vi "MPI2_continious_implementation.vi"() -> ()   [LabVIEW 2019]
uses:
  <vilib>/DAQmx/write.llb/DAQmx Write (Digital 2D Bool NChan 1Samp NLine).vi
  <vilib>/Analysis/baseanly.llb/Mean (DBL).vi
  <vilib>/Waveform/WDTOps.llb/WDT Number of Waveform Samples DBL.vi
  <vilib>/measure/maspectr.llb/FFT Spectrum (Mag-Phase) for 1 Chan.vi
  <vilib>/Utility/file.llb/Write Delimited Spreadsheet (DBL).vi
  <vilib>/Analysis/baseanly.llb/Mean (CDB).vi
  <extravilib>/ChannelInstances/Tag-dbl/Instantiate.vi
  <extravilib>/ChannelInstances/Tag-dbl/Endpoint.vi
  global_variables.vi
  <vilib>/DAQmx/create/channels.llb/DAQmx Create Channel (DO-Digital Output).vi
  <vilib>/DAQmx/miscellaneous.llb/DAQmx Fill In Error Info.vi
  <vilib>/measure/NI_MAPro.lvlib
  <vilib>/Analysis/NI_AALBase.lvlib
  <extravilib>/ChannelInstances/Tag-dbl.lvlib
panel:
  in  "Rotation homing":bool
  in  "Align laser":bool
  out "V":dbl=119.6
  out "f":dbl=60.0
  out "Power factor":dbl=0.42
  in  "Enable power plotting":bool
  out "Waveform Chart":T1(graph)={"apparant power (watt)"=260, "active power (watt)"=110}
  in  "Pumps":bool=TRUE
  in  "Bed motor":bool
  in  "Motor":bool
  in  "Clear plots":bool
  in  "noise floor stop":dbl format="%#_6p"
  in  "noise floor start":dbl format="%#_6p"
  out "noise floor mean":dbl=nan format="%0.2p"
  in  "Notes":string
  in  "Shift amp":bool
  in  "TX amp":bool
  in  "reset daq":bool
  out "Main loop has stopped":bool=TRUE
  in  "Update global variables Button":bool
  in  "sampling rate digital out":dbl=40000.0 format="%#_13p"
  out "Duration of last non-idle state (sec)":dbl=15.425420761108398 format="%.3g"
  out "Start of current operation":timestamp=timestamp(3649930230.9464383 s since 1904-01-01)
  in  "points to cut off (spect, baseline)":i32
  out "waveform diagram":waveform(dbl)(graph)={"t0"=timestamp(3649930210.976007 s since 1904-01-01), "dt"=1.9999999999999944e-06, "Y"=array[1400 elements], "attributes"=variant("NI_ChannelName"=variant(string "DAQ2/ai0"), "NI_UnitDescription"=variant(string "Volts"))}
  out "current system state":string="Halt"
  out "readout pts":dbl=1400.0
  in  "TX cycles per readout":dbl=70.0
  out "fft phase":cluster{"f0":dbl, "df":dbl, "phase":dbl[]}(graph)={"f0"=0.0, "df"=166.66666666666714, "phase"=[0.0, 2.7540425593822215, -0.41774944944908105, -2.9917235526827883, -2.707459047470282, 0.6249454301823627, -2.370005265361227, -0.5147516054486614, 1.6292245581402647, -3.015048559086423, -0.03670352730802006, 2.393200344197681, -1.08044143469344, -2.6803908360592543, 1.0570394839460617, -2.5979273293198157, 0.3746003915660465, -2.5959706251713066, -0.19275351229231943, 2.329251585108698, -0.15760892412814748, -2.619444396039319, 0.6040257569791547, 3.1232384157346744, 0.07286862625539897, -0.8349761222120895, 2.491919747557329, -0.6723952580821412, 1.4219523114985915, -1.8829118421278235, 2.1285349521917487, 0.552356415038526, -2.875631612970751, -0.05342422351139544, -3.1202940735703035, -0.2709814792342252, -2.311185357352345, -1.811383998858392, -2.671748431800669, 2.9870683722179363, 1.2306850799385998, -0.6468134335002678, -1.870147290118833, 2.9036130612188034, -2.3983442820995076, 1.5668696744042487, -1.485293516020373, -1.774984487522115, 2.9625095772350805, 1.2114987717362917, 0.41687473942441583, 2.4687530236172606, -1.3355374526401789, -2.7968528807659343, 2.101943215520195, -0.44240091404557225, 1.9209832862953178, -2.4648296902330324, 1.5814005745822983, -0.011182563965032996, -2.3033844922829383, -1.063349381886634, 2.98362939203973, -1.1699060479297414, 1.692187942816072, -0.9709312181777011, 2.5840242996804395, -1.2778035123496316, 2.1573220622434386, -1.454711675166049, -3.126308692769843, -2.9063943164949992, 1.8154945850625546, 0.5378211152892565, -0.5635004704527551, -0.5179360533926947, -1.0664830762078226, -2.85578162582117, -0.1307304567139906, -1.7830942043670113, 2.168572519489484, 0.2539399701165289, -1.761995933961074, -0.7037883915148042, 2.9248931112795344, 1.8880708587138288, -2.405324710669905, 0.4964528358342285, -2.2335794668638815, -1.8563013263901713, 1.1702254916879868, 1.346821279336611, -2.204173805999831, 0.24371100375848012, -2.7832475464457582, 0.5149589355035561, 0.8642594420795789, -2.138465254643337, 0.9421221120770275, -2.2015830793659377, -2.2320581146103033, 1.3064962642298776, -1.3403297469040394, 2.831661840993031, 1.203650750034212, -0.7830936947340748, 1.8935054792408772, -2.982278658911026, -1.4551705398152555, 1.4824075372105057, -2.0350358049171713, 0.0874608635446794, -3.0012334842500716, 0.7449814218063762, -1.0233846855331499, 2.8169824097043756, -0.8475187075508479, 1.7026399735381448, -1.5828785893756976, 2.411856644890007, -0.8925026524492577, 2.529100008950798, 0.29438318954641246, -0.7911902624060129, 2.7211777807148003, -1.4801195970408665, 0.32176108872110215, 0.8595087554168631, -2.91647820235481, -0.9096511107313615, 2.362809138152293, 2.907293981342496, -0.19224313497452372, 2.021057879936991, -1.0532144735572766, 2.012519718095534, -1.9914830889397996, -0.940305290573743, 1.990900580773453, -2.8166056044414414, 0.009837509283864954, 2.6788318641404985, -1.2304335536026125, 1.4372667618862258, 1.9357764794837633, -2.2510950656975703, 2.4346628297411255, 1.5058836975878664, 1.3396962452554966, 1.447915869036184, -1.6397026839530333, 1.504171455527829, 2.6168212185699384, 1.5694053636606018, 0.8991085911788249, -0.0060969118270417086, 0.704108075898119, -2.194015123877586, 1.9294214533962404, 0.9906316293947478, -0.8888372568865064, 2.289162228251758, -1.011412315749929, 1.7752562681031894, -1.5581078939472532, 0.17859807760715082, 2.874735233191739, -0.15245359027497854, 3.0007011237769623, 0.47492116042589866, -1.9517413705962434, 1.7541787652288416, 2.871211783717952, -0.6988862767001006, 1.6592170814733889, -1.984724345919406, 1.000667097748792, -1.277392682860055, 2.300663190120588, 0.9406642267225795, -2.225627302386333, 0.8369524876201423, 2.1419482177162994, -0.42734478695542544, 0.4971445385035397, -2.7772254798843785, -1.608828736322811, 1.6012576563947614, -1.9311241954870342, 1.1601617761002088, -0.16565949427291773, -0.8987336035561053, 2.7497346870958994, 0.15519553252081572, -0.504666162696194, -2.8946094052857503, 0.278888380464233, -2.5469229535229547, 0.9428862750232928, -2.2147669202386036, -3.0087387411619897, -0.13435457211182855, 1.8814556021187567, -2.821844805764982, -0.23032398091776898, 1.9406188587639086, -1.8842189519459873, 2.2014589910538898, 0.07337478156413231, -0.2911302207205093, -3.0449435192482284, -0.09316913489557556, 2.7136612125692263, -1.3430930954792781, 1.5138143613458557, -1.8498842584956878, 0.5518502747380236, 3.0080618183329366, -0.707945162576425, 2.703170009927386, -0.6497057490505204, 2.855450909859158, 0.26942250168014553, -3.1380634262559677, -0.6082811318546472, 1.8516114361794906, -1.668703750723555, -1.1764032056055431, 2.167716520633288, 1.407463459861506, -1.1939240181202087, -1.96033710810533, 1.187929862874151, -2.1284796193857574, -1.1135935933886567, 2.240393949288565, 0.7996933890629445, -2.57345171230255, 0.8624884057397524, -0.18394354977004865, 1.8027756604193184, -2.6673785459645694, -1.557213278823325, 2.5061775387898675, -0.7343428839851375, -0.17210152756946395, 0.24209791907571915, 2.385818454154299, -2.3543740463234584, 0.6542443429026227, -2.3887773967085653, -2.6994947310507627, 0.16374411301341452, 1.0844343637975538, -2.6690989874740985, -2.1301846552924837, 1.1305365372322789, 0.09211758596205234, -3.0431302638218725, 1.7433946946046488, -1.1964783090414477, 1.8527259341334916, 2.6471322822092316, -0.1747334806929663, -2.4861274055177014, 1.4236536162233422, 0.3224756043586924, -2.282310592209435, 0.3675863113242476, -3.062406752340649, -1.8048033049988987, 1.0339783508118279, -2.09586975663964, 0.7136083863527781, 2.7684330693562704, -0.7197481447382043, 2.670741867219946, -2.7957835404308424, 0.4756994642649445, -0.7547478534353032, -2.68586463998786, 0.11520506082972987, 2.3080887100868286, -0.5193216124366172, -2.9418065387151104, 0.8233942001211878, -2.3666441340336672, 1.9683026725269523, -1.084741955010314, 2.569431696746155, 1.8755768382902336, -1.735947948757583, 0.9158590456066058, -2.2488121057461252, 0.41900190348061833, 3.075960180992822, 2.4449872373857415, 0.3478853662006557, -2.3868864643332484, -0.7271255775728059, 2.4025639827624645, -0.6435555179469675, -2.900614106450232, 1.2388665786563127, -2.177306974845179, 1.2653133914574806, -1.132271539866567, -2.548990032776874, 2.370901279573129, -2.621199170173867, 0.6351848695609148, -2.309600610728719, 2.0369830137151075, 0.3265170729861214, -2.4499662648349423, 1.0087071287256246, 2.933669450086174, -1.417787571775661, 0.9076499105418954, 2.2043305075404036, -1.095109907014107, 2.050631628894733, -0.43008279174513486, -2.646699898696328, 0.5058833203755909, -2.110149021934083, -0.018918678796171286, 1.6366055531490655, -2.9565156100247982, -1.7980864195189612, -1.787336416541855, 1.6658447403981775, -0.6423657898020487, 2.7228871600915094, 2.497696300061502, -0.5646022220607995, 2.5896486310731213, -0.9023305265342931, 1.2845535414267544, 2.491477036620103, -0.793986898054272, -2.3598613453772, 1.8413389615810676, -0.7684267125264834, 2.986826489821479, 0.20901586046963358, 2.6427706874636714, -0.6754994858774919, 0.7912549355498941, 1.7487296459784962, -2.1072546596021295, -0.9966227622577787, 1.6328904486354898, -1.440773592697903, 1.9527647218101232, -0.9457649334446133, 2.4632987804112476, -0.3489955760626715, 2.5485323033875837, -1.005446962543904, 1.8683396278373134, 0.5531580992213784, -2.0682094583995325, 2.1785865491901446, -1.5253052839334211, 0.5315754829936222, -3.1250591763931, 0.15293660563839134, -0.5606359064596489, 3.1207390055910844, 0.25130904796050746, -2.9637815190386334, -2.5906696773361673, 0.743539865125924, -2.0635632215919726, 1.178460956556411, -2.2543432193778905, -0.5532661646812833, 1.7664410828245412, 2.0111450533039394, -1.120565684900094, 1.7986953093227194, -2.5415433153559417, 0.510868468073799, -2.7591935826661134, -1.3427432839709943, 2.0382642767004566, -0.8394413776070548, -2.537338985742467, 1.002033243911298, 1.8091856452425523, -1.7674405584336437, 0.35920606546557676, -2.4706157972378286, 0.7392519149737825, 1.7831960704815513, -1.8258580537840825, 0.7959328221750316, -3.0725238341834538, 0.01686990355077934, -3.0583047227202322, -0.589141148651516, -1.0606439709776083, 1.6681409593854466, -0.8869758395603837, 2.332987799635121, -1.681743700117981, 0.13265483928652452, 3.121424240790634, -0.4302490296605881, 2.0535402105381864, -1.5961317869067708, -0.3662549325580801, 2.416822962602054, -0.2904396313468742, -2.889336327493639, -0.23429968311574736, 2.545959095082067, -0.7096192469411521, 1.964741364163201, -1.730041669682325, 0.7090398077350987, 1.179690399659869, -1.8155853465290495, 1.2571528050807952, -2.6132504193125614, -1.1657097950185642, 0.9898389298050183, -2.1610027927415176, 1.1238212113010064, -2.7622547361674354, -0.38620274248449354, -2.984491475078884, -1.1801494512425614, 0.5079510451233106, -3.023239660006938, -0.14793964854238115, -1.0028641759351438, -1.8298714248779389, 1.431752830327668, -0.372604565289599, -2.111976907728673, -1.6051535714270946, -0.627399219833397, -1.5783940037689044, -1.6151441217412108, -0.9497452635424707, -0.8340388727489995, -1.6981535879152772, 0.38263659597426025, -2.968210990658363, 0.1730726497601832, -1.9153705321290466, 3.057546157287166, 2.205291722470598, 1.6134501828765986, 1.250953281266258, 0.9601343829974033, 0.5343499781125347, 1.3276675906004771, 0.5965879699558632, 0.14414069135444182, 2.8560398694614886, -0.40870446717026343, 1.542638627591486, -1.7960924268234595, 1.7145806375689276, 2.500728281163647, -1.3474489556512186, 0.6253773444357569, 2.1805456021135634, -0.0017853382921967362, -2.3700748617367458, 0.7717998892014187, -2.4682854842096864, -2.688099696833425, 1.4569756741555677, -2.022850117504677, 0.18146352087647405, -2.968035460087035, -0.3241793599380396, 2.2471208533035325, -0.8831825977854595, 2.830504149007527, -0.33506201397387, 2.8351405178488847, 0.2776696262316505, 2.9016066946593515, -0.8334126357193999, -2.507987526741747, 1.7426671623773033, -0.5417289161786527, 1.9224500719008697, -0.41496442296770203, -2.740802203027978, 0.00014411662639131332, 0.9885353149138045, -2.414084469045593, -0.14674622925736786, 2.1172083456191193, -0.5764227996247283, -2.19817138362822, 1.3689091158563123, -1.3322519629050043, 2.083166488628662, 2.75850235428238, -0.49569633158574966, -0.6091556660993676, 2.566654679807459, 0.5386278640586663, -1.7642954489637717, -0.2708519584868171, 2.6279278558234584, -2.76052145328226, 0.48234061791548194, 2.5679926362186523, -2.6064532140875, -0.02976639846895066, -2.3184427483744505, 0.33310384188549014, 2.379566379985213, -2.4465268020446604, 0.39191389408301736, -2.526036530944832, 1.7502630624088855, -0.6756243250094364, 0.7496052763980502, -1.4311402830397941, -1.684638761248864, 2.508989348459718, 2.1318749250863065, -1.627395188562372, 1.69214376606126, 1.3279942776168816, -0.8967371816826627, 2.674525668922968, 0.7278845134135274, -0.7453134817296895, -3.127933580573263, -1.4559858116436293, 1.5324073348385072, -2.2623698937484877, -1.2139904917323259, 0.3321865326835266, 2.774517907470611, -2.3834916405953406, 0.3775992516468575, 2.618557600355517, -1.1193506746267166, 2.4056012218302683, 1.0953081251316885, 0.0807635245525032, -2.8650175176315202, 0.06633059915074543, 3.108255648457706, -2.6281555013584885, -0.6728493883792693, 0.8982170775552722, -2.467911848936858, 0.2251130879432983, 1.3094095682743723, -1.7452461822975973, 1.9037671101602498, 0.2692816197561913, -2.60491544045963, 0.9509370482944391, -1.5596027897702691, 1.4429396515357684, -0.6550794488655424, -2.7970786630866233, 0.9465406749391486, 1.6972717539201554, -1.2358512552745493, 2.859757330129867, -0.651431969761258, 1.7813157508986759, -0.30018991623442065, -2.458829645707201, 2.4969055139900473, 0.13417138886497348, -2.7272428970903015, 0.27959215724505854, -2.713140546404327, 1.353315685896636, -1.4000699525981828, -3.023919861797397, 0.2139738186814114, -2.823704653256064, 1.7619580750329171, 0.14704980762164735, -1.367346362825192, 2.512174923849862, 1.292702694201784, -1.1543087848414244, 2.9685391033225974, 0.7220485420721938, -2.0570513351693864, 2.909710283102838, 0.17750819285937092, 0.9325849307591031, -2.501919311348002, 0.2171392757353715, 2.7197205937735576, -3.0015410466578762, 0.07892066384111603, -0.7734069722456183, 2.7946610195263304, 3.0212781609776433, -0.8017779037675032, 1.1969569933354216, -1.9859464554741195, 1.939696103455967, -1.479006377403267, 0.019995563226488648, -3.1230115438008226, 0.4342424774532695, -0.6952728305939098, 1.0229816409655819, -2.0603758042900426, 1.5631148611946764, 0.08252682658156427, -2.9946476005647775, 0.4541553124739888, -0.9826447835513735, 2.568571608998873, 0.5034463974116944, -2.2512370293978603, 1.9247937512429683, -2.758186529451972, -0.16328327349004884, 2.745227824640305, -0.27600472719070634, 3.0600663251670555, 0.5779793580418898, -1.9351508978905139, -2.944062127388997, -0.20463752723418507, -2.448553547905565, 1.6282989165337824, -1.080180309237574, 2.3032306343237092, -0.9351289289356145, 2.4810288227515636, -1.734998585032266, 1.934163102502813, -0.45517004339773137, 2.6260983195493113, -0.6252942634230008, 2.05345376947151, -1.2052358411757857, 1.5851434346391662, 2.9155968859671746, 0.8752613202637856, -1.6525755089363785, -0.18463853833227828, 2.7234047295485433, 1.0988545465606525, -2.242297665425119, -1.3937619510909733, 1.7504658443134995, -0.7807866519805128, 2.121795666896204, -2.4988185645044565, 0.43643795207773683, -2.5623206804319585, 1.9672319186012786, -0.4313809716611365, -0.7503110065885348, 2.6056452791860774, 1.8652931339656367, -0.485714124275401, -2.539908636212827, 2.1509984636830866, 0.617245296619356, 2.104623489256656, -1.6261802407185368, 2.1039289728202717, -1.470700521706089, -0.2510745221059939, 2.8155156715551573, -1.062791518472392, 0.8526886580626974, -2.2270616100970773, 1.7939297977550315, 0.16220909589713345, -2.7184764916022828, 1.0984464241275225, -2.040486566556227, 1.9740729635161505, -0.6049131727905106, 2.7647763575194975, -0.31890901315428244, 2.6595529123025985, -0.6554028882543155, 2.702171327717349, 0.15427593482135468, 1.9407164797032128, -0.7116792237513718, -2.9193685159956813, 1.1603672499589228, -1.253714460479042, 1.935104327522088, -0.9520698051053289, -2.945208479144284, 0.35300344973637643, 2.992141452530448, -0.9510545269233662, 1.9083188149179684, 1.882296639370573, -1.4127340898414624, 1.6581147173382742, -0.544081968873865, -2.9563735924869357, -0.23792907945643266, -0.08664421899668712, -3.0511665382909405, 2.3505331162555323, 0.3512590798471839, -2.203577644317914, 0.9243401829327751, 0.6905016989305272, -2.3172011699802906, -2.986497393871459, 1.4895757424726912, -0.7053727827563905, 1.4737838061842574, -1.5915714213345427, 2.260194344780683, 1.5371012239548374, -1.3671078645599828, 1.7701943352995453, 2.9799474066776237, -0.6169901641100062, 2.68023055792731, 0.6180074382376435, -1.6846735239867856, 1.021292517899627, -1.0321392572442891, 2.2387531179741296, -2.2775262175929574, 0.6730136922793635, 2.705524130615674, -0.5254342180261299, -2.398299277522749, 1.8867356604206764, 0.11037861917104375, -2.942603830022654, 1.2291602551064613, -0.04643970966507774, -2.6051215703608994, 0.3948810976564284, -2.7638261340669663, 1.3927119884264614, 0.9648717030418312, -0.6733534746885191, 3.0699125697465384, -0.7954344221272802, 2.665745109387664, -0.7524637482497626, 1.8833978480366045, 3.026059640211306, -1.0207202873714734, 2.3918077211986306, -0.4732538429732604, -2.5493565318250697, 0.3097434901148436, 1.4755826933358034, 2.8996652120089963, -0.4639338999555499, 2.6481298733314644, -3.0481693440909443, 0.5639195937204325, -1.758123653081914, 2.0929164865234466, 1.0493983313679878, 0.4312341153399969, -2.5133529048769514, 0.31115309972833816, -2.205936725953789, 2.1468878985231394, -0.19671651990435773, -3.0141022994885893, -0.011128100459949448, -2.5164803826644926, 1.0175456302091626, -1.3745587291818357, 3.0138020218299157, -0.863730804102301, 1.8539905645950367, 2.678613356195852, 0.012121176241664998, -2.9737392540851046, -2.0563045653546963, 0.5660548089094544, -2.839787969747755, 0.7374086590379478, -1.6218177124508901, 1.4298262102156536, -1.771981769179663, 1.7931352101075406, 1.1105421554248707, -1.837566617004617, -0.6081073819394741, 2.5754499806209328, 0.14414269190237375, -2.5381041776371185, -2.1671892146822347, 1.1297651827584954, -1.7667261074505065, 1.2808578780285342, 1.9383859858025012, -0.4572259173897579, 2.8353034618734463, -0.9824569319790475, 1.667026318737601, 3.1215096968456053, -0.773559819860795, -2.9251112684627536, 0.6384286174678868, 0.8474754773092013, 2.9824953300218984, 3.0981295192162523, -0.5756120764182968, 2.5802849339589327, -0.5168310323829991, -0.07536248392628349, -2.543567087752712, 1.330719873268674, -0.672328576433985, -1.7115541995753467, 2.4084502255455558, 0.17957388304270258, -1.0380143874522993, 3.1252796220180765, -0.13901807785019424, 2.900568902256346, -2.6746660644621723, 1.6812325032291666, 2.5936178017610914, -1.0577483903197933, -0.8583091787121501, 1.515660036925533, -2.288459367658298, 1.3343629995939172, -0.4274448443593649, 2.4571136013982002, -0.4514562840751234, -1.2459111684655748, -2.4490661605501023, 2.5527831908431486, 0.5136959710916381, -2.1107549720777308, -1.0368956909031488, 2.9033136714750096, -0.21460476883399254, -2.689728080190454, 3.0439216936452156, -0.09795262227017294, 2.495749703976162, -1.7337508509795796, 0.25146923034204327, -2.0885774040569083, 0.8030869762721157, 2.919646309739889, -0.6783614578476972, 2.65700015425027, 1.6630001934159717, -1.2705251868450735, 0.7130202847030426, -3.0636444516065895, 0.011216775739950453, -3.1074220264578942, 0.010653244934669395, 2.176503184995665, -1.042058025631164, -2.67562504444696, 0.9654930883022897, -1.4312407947889514, 0.31867196180608687, -2.888467320932099, 0.613547057450556, -2.7482398180779217, -0.34003922390177443, -2.8630408227079833, -1.4663748131970828, 1.1978104188470686, -0.338750516641942, -2.5354950119151165, 0.39584642658634744, 2.2511823430250395, -1.5206567069495636, 0.5330347182308556, -1.6083717577366752, -2.475568169172881, 2.2796480203603227, -1.5156290974975193, 0.8345075361033615, -1.3669377623560492, 2.529509560230595, 2.09492643521411, -1.0205181753606163, 2.2327577001586647, 1.9726293368884513, 0.2029707975484194, -2.962900764202443, -0.5912851593807913, 3.105708278247044, 2.057255299370193, -0.3900127338099452, 1.7886451892465023, -2.059711724130614, 1.3011946673805337, -1.5158133970234138, -3.071927339455458, 1.0784354873987443, -1.4414952745849792, 1.9024703445658466, -0.38953015878567476, 2.315543251618792, -0.3270227324776918, -1.819402089828396, 1.1714367420411165, -1.7380447678460644, 2.0226154246428876, -0.5656353587346558, -1.6388821641965623, 2.6647644706072753, -0.3697828832600953, -2.5990669276454588, 0.3394265001700578, -3.0871215131184915, -0.03350977552078354, -0.47388143557915846, 2.148618508348748, -2.460425643942731, 0.43227270022262343, 3.1306384331474457, -1.1054930079495384, 1.2915146249735612, -0.555730780954817, -2.5163788057804783, 1.5968331686665074, 0.2477077194166366, -1.4569263346723451, 2.8151633575495674, 2.458755159018332, -2.059473678369277, 1.9881149241942575, -0.10954623369266984, -2.638069181200175, 1.884271559232175, -1.638827624975623, 0.9442813603265399, -2.8954472852291118, 0.6539096133858422, -2.025487143592496, 1.3076127014601728, -3.110745479326435, -1.8108764067652123, 1.2535816088577916, -2.200309258511845, 1.7704029552736777, -0.10815007670568688, -2.1757302998662493, 2.069671606981699, -0.4040626261929413, 2.313319809828219, -2.8691010275234, -0.11070784799500669, 0.7580114702723455, -2.6368150447497802, 0.7786284956298831, -1.1688754608227738, 2.916639989523171, -2.968274492665614, 0.4757893735327881, -2.7930321897916777, 0.33977081228081796, -2.360076014238439, 0.784272132681561, 0.3816169080494048, 1.4138255765856176, -2.2095040314658436, 0.6429916063604616, 2.7099700619726868, -1.3024182827089108, 1.4084463395259685, 2.0120981573443775, -2.4824353152453513, 1.1189687853754873, -0.6621056013313161, 0.17405887909554316, -2.811518724102276, 0.5404116271585312, -0.971592405781462, -3.1101754651938243, 0.424513927079209, 2.8877867311961305, -0.5701659100467101, 2.161845744491495, 1.0255431872389773, -2.885417486370385, -0.6725110302329639, 0.7605370190311493, -2.1756109466854046, 1.39592471681857, -1.18718719947846, 3.071881788840178, 0.06928131896478305, 1.5515471497920168, 2.2534137223650204, -0.7509931241834826, 2.9870296745806155, -0.9699385683796223, 1.690007832778289, -1.5566776002508034, 1.9742269720166967, 1.5123133398558415, -1.1211534391671651, 2.775941078499385, 1.824535890111235, -0.627882744192828, 2.0628455538485078, -2.7163450356766727, 0.3900351550836249, -2.3565912542326815, 1.5862569686623909, -1.6820567568245655, 1.2656930128045998, -1.248767728135985, 2.3269802892746276, -2.643033485675305, 0.17989784769887698, -2.1922092890411435, 1.4690893308703339, -1.5379352487014688, 0.6572453052429962, 1.6842351250708696, -2.365675887125544, -0.31369855067107055, 1.7403172098317616, 0.5746113943672305, -2.250536359076875, 1.422406633442669, -2.406467601746575, 1.4163252865729303, -1.0137162472144192, 2.8248943291717987, -0.4829320883796166, 0.9556509464491407, -2.2728204359978195, 1.0958698376082479, -0.6943175232570544, -2.070141542478213, -2.6302750708447316, 1.0480219071710373, -2.6654695672821624, -0.3026625700254163, 2.411045156197171, -1.0747427904257583, 1.2585000062890082, 2.5376691764983175, -0.5072232455501554, 1.7118305492921926, -2.19296103703589, 1.5654690366761803, -0.8063444602960661, 2.346707883955403, -1.010870306036241, 0.26652490258268285, -2.6988212917660372, 1.214597876704182, -1.505599104941634, 0.9543231399620783, -1.9837536099576925, 0.9247294624069821, -3.0448114616357485, -0.16654781886801737, 2.7048675120923535, 3.0162008538548313, -0.6920223381518189, 2.136141031576818, -1.3435825844179943, 1.7613672789484416, -2.1323832154962212, 0.8937603953136487, -2.551934824567234, -0.032141997296331146, -2.0702708085515096, 0.3569935562951153, 3.138823246315803, -0.28677655612910685, 1.0937418839126127, -1.84696097134991, 1.2565218073270858, -2.1285667574718055, 1.7121777620402516, -0.7402364284457075, -0.5091012029515373, 2.679852230441668, -0.4663018106384946, 1.9646665176016138, -2.3490534053699594, 0.7434703495975993, -2.9270735344351753, -2.2192593699371357, -0.20343072390159692, 2.245202462760766, -0.8495160616648074, 2.736318754992669, -0.21926089395165413, 2.5895536433032396, -1.7070096330032456, -1.0158083234055626, 1.452082148142477, -2.7189201079413565, 0.6923374549122202, -2.202556430943985, -0.9598405920890763, 1.788887017419821, -1.2338374014075575, 2.5965353632046546, 0.24860417664545903, 0.8924295752251784, 2.4073221061901533, -0.8770193558937903, 2.7618139550642233, -0.4435649705201455, 1.6471660768484968, -1.9748071660682311, 0.44248007716085386, 2.799384288444242, -2.226381010413999, 0.9494920655618904, 2.5196130139941197, -1.4032319700724956, 1.156495437663549, -1.8652931884384618, 3.0734659384121423, -0.26951929480409204, -2.8799692983307814, 1.303443303659596, -0.01978267175402987, -1.46811291567088, -3.051808792277222, 2.172311436021013, -0.8633480637476854, 2.431690186189021, -0.502751629385919, 2.9201500020941165, 2.5238871360192436, -0.4358777467265639, 2.5031055651863485, -1.5261691124512629, 0.8474355529033445, 1.8119516925067631, -1.695209497216864, 0.6062659246966707, 2.9278478628266438, -2.9096310368197797, -0.5264754350964214, 0.9743930725392232, -1.3552922412853734, 3.0768304028614333, -0.3045539459195762, 2.545587789637512, 1.0324084035309868, -2.8613728394988107, -0.22277134258671846, 2.1245439525922727, -1.7238869923731035, -1.4627701565418878, 1.5086505616512276, -2.794863290434653, 0.15568451237741993, -2.195604094562416, 0.7216988967484212, -2.8572756589490513, 0.07357909971429183, -1.8287009331454764, 1.9966034479124604, -2.0598928673726524, -2.7896496017022465, 1.0676418569974464, -1.743983906588147, 0.9794982349133036, -2.7542212982327983, 0.9422963219469825, -1.4370521423633564, 2.385856217689936, -0.7786724496108143, 2.551264284658099, -0.7874950333562143, 2.203748769329088, -0.7485047904414031, 0.8825489131884457, -1.4784413322922143, 3.13523734436019, 2.228584933254406, -0.5794369723331801, 2.1424595963295383, -0.6590298006070042, -1.7673187970416888, 1.3699134662551367, 1.0695962209127687, -0.960581932847277, -1.0390943138184625, -2.449443096911296, 1.614483550033886, -0.9830076477571836, 2.168992450309726, -1.370685572931924, 1.3565172872579825, -2.336386965297111, 0.6197910802692542, -2.344161346619624, 0.17559552046889557, 2.313696728982058, -0.5684404265838676, -0.7749491636146788, -3.08615199767987, 1.9320643623556393, 0.6634529752684392, 0.06654448657712722, -3.0846790730979867, -0.5053088046114536, 1.388371216006345, 1.5136242882194861, -1.51033316842799, -1.9438280385585442, 1.4695412483933843, -2.7450529165441306, -0.5450429483514694, 1.08821543163101, -1.1536503086138679, 2.453191802448807, -0.14335654642151924, 3.052322964862365, -1.7233507784018072, 1.3309913884654867, 3.1226591858947144, -1.9563531633252866, 0.14333284809700247, 0.6654675074875196, -1.7833475498409017, 1.5282033576705654, -1.0656760212139198, -2.7320419116991714, 1.6261894703171715, -1.934384938212058, 0.7871542119401843, 1.6891205955520372, -2.965472955499157, -0.3967496308230906, -3.0209591975850385, 0.7063283717786318, -1.413839697723809, 2.3047235633751937, -1.3456233748583486, -2.310748993303288, 1.3380455605483028, -2.252353133687334, -1.007578212142689, 2.3192984231574747, 0.9829741984675008, -2.3883495102595895, 0.985764991350256, -0.23856867868005707, -2.383074033654719, 1.4666665363684508, 2.9017309889736675, 0.3525688778641894, -1.757333800399145, 2.050124180950513, -0.4334326096421342, -1.9602427501701536, 1.929307400330661, -2.267822856698649, -0.7073421157798139, 2.4611492749524975, -0.36640557450473993, -2.6181500528549475, 0.40311055493507936, -2.434224007134926, -2.6465143721565436, 0.7134239266934059, -2.9196238148015814, -0.09897049078233182, 1.2226737642483225, -2.1801890748649915, 0.9638460741031623, -1.0292078704281071, -1.3161387756552627, 2.131340361529748, -0.7366771588514918, 2.6785776346815053, -2.431888850726272, 0.8510075408044548, -1.7215064324000349, 2.271449613138369, -0.9397678306538603, 1.4176857754442111, -2.458316780997201, 0.3333479386073043, 0.6466892932019946, -2.4887283094011505, 0.06595588362458445, 1.7759416516491897, -1.3156378756967018, 0.681677176848216, 2.767500360407054, 2.4290074442463867, -0.5584934107391647, 2.2838355888640103, -2.6693746295278897, -0.721500161550526, 0.8305472686604598, -2.888838211223999, 0.36049127801667946, -2.954461068886556, -0.29106076906884115, 2.4473111593457317, -1.1653984597050084, 1.6454200188089136, 0.1378818071348789, 3.124422709808076, 0.04655850838229611, -2.9936604660172463, -1.687842044638684, 0.33737683243916466, -3.081329400775572, -0.38940882241971325, 1.607881826268852, -1.4847441989561796, 1.6828010851600108, 2.727607794269626, 0.773393474612303, -0.939151684254625, 2.749308071835674, 2.4307800176874363, -1.396012027360456, 0.9399631537318961, -2.7377937319746755, 0.5961403313257109, -1.3913579604427555, 1.8523201530045845, -1.5796704556798358, 1.4513031618879204, -1.2044533178095884, 1.3291082982313418, -2.6513554186879857, 0.6763463839115226, -1.3223224094413768, -0.9027729644935903, 2.5402903148445195, -0.5026447652791285, 2.3899878465783746, -0.5887832929819106, -2.817503179132805, 1.1009979435117832, 2.2974331248869606, -1.2080094832204378, -2.2872069739795218, 1.5575981437099562, -1.9878334777061717, -0.038678558051125085, 2.989398615266818, -1.4773564061913294, 2.7737627042041018, 0.5980708974361006, -1.3624946494378485, 1.7763885881955879, 1.3667932276339032, -1.4625626897188568, 2.878017820047102, -0.11019615609114743, -0.21195385518571583, -2.8310117596111644, 1.1315727312499262, -1.1563589526596563, 2.40762124116393, -0.5690256392438064, 2.3944419607360867, -0.4956887515079857, -3.069507078353702, -1.0410117525010907, 1.130387664652052, -2.1975704116127805, -1.8636668302021266, 1.044772750789791, -2.9994187336065674, -0.7615262200237719, 0.4372035572332126, -2.1754524438731413, 1.7419915463934326, -1.1888370085726094, 1.1430422422881916, -1.614199113484965, 2.3859546088241785, -0.6687711925523698, 1.6593150552017215, -0.8217719041293505, 2.297889400522578, -0.5980122260232852, -0.030868183427800257, -2.8379302107248097, 0.89747935739299, -0.6849577627070423, 2.306817241582839, -1.4091867620722667, 0.15565424042509343, 1.957221035234614, -1.9367384535278211, -0.9734280147034378, -2.12430784881939, 0.9159536225275885, -2.189467486661428, 0.7078939097471529, -2.3986898995946593, -1.5683999989094228, 2.183702732591611, 0.047984705354305365, -1.1985977902963327, 2.3459461687072842, 2.164583253229524, -0.7529445870625288, 3.0021777991611143, -1.0097920527194986, 2.3810424364901537, -0.12342570756526414, -1.0740703664218525, 1.8949006922375287, -1.1214960989448763, 2.215564246850753, -1.4748614852061788, 1.3618809852566327, 3.120188806624154, -0.8508708903014319, 1.168379273243559, -2.445796003750018, 0.202400316559645, 2.999193446426725, -0.1894216674062962, -2.6000397626931386, 1.3115030806337187, -1.5295304473323301, 1.4445198466548173, -1.1222069380003843, 1.2476829207573232, -2.4211544681343677, 1.344471534164131, 0.7439596447231648, -2.9031710679521052, -0.06576970000470049, -1.569925849484693, 2.2423593955489034, -0.9691866068739777, -3.133832899196044, 1.2362132726018655, -1.8363430644515046, 0.38224286375236094, -2.7297120299135744, 1.073909406326477, -1.8094074377887333, -2.16647704505428, 0.8379742129973163, -2.8677096274666805, 0.0914608497055886, -3.0419340053702015, -2.7650747242481453, 0.23681574608022923, -2.835734101467477, -2.02158524567706, 2.4080064173132616, 1.5730195632065045, -1.4778688355793552, -0.36303301687268197, -1.4057781374689775, -2.8884924811780364, 1.290145701837535, -1.3133809334787196, 1.536818216317374, -2.351388669904487, 0.2948797207736677, -1.663353362631088, 2.8734673058340725, 0.7002148139700289, 2.911734354686056, -1.5149789152715065, -1.9601639064457783, 0.7583223995676716, -2.59053564326091, 1.755829764903252, -1.6007208412621265, -2.2676024351517583, 0.7397083027550687, 2.762988681409429, -1.923385581440203, -0.24646772608763412, 2.763215765590017]}
  out "fft magnitude":cluster{"f0":dbl, "df":dbl, "magnitude":dbl[]}(graph)={"f0"=0.0, "df"=357.14285714285813, "magnitude"=[0.0008504053868740763, 0.00038817631685509143, 0.00024200224947985637, 9.528178631548858e-05, 0.0002637879165738081, 0.00021266182371736548, 0.00026328121141686847, 0.00023246712294296184, 0.000170218058535424, 0.0002214629029401282, 0.00018340054429958835, 8.001472603600311e-05, 0.00013754196060766958, 3.217049878774864e-05, 5.537673098252246e-05, 6.655938865999862e-05, 4.616030095470193e-05, 2.1630531609063795e-05, 4.179763229329e-05, 1.8814796240273995e-05, 1.3861298250629736e-05, 2.9069300780021175e-05, 2.8472339253991566e-05, 1.8424246742207424e-05, 1.753088012974326e-05, 1.306056803504805e-05, 3.4577365984582725e-05, 5.301188067480479e-05, 1.6759110050633133e-05, 2.3101475044572646e-05, 5.177641082400739e-05, 3.394906563604761e-05, 1.3132867773952802e-05, 3.1681502670681254e-05, 1.9715168809233675e-05, 1.3985884261973671e-05, 1.837749235084362e-05, 1.9973617836840333e-05, 2.4255481464396008e-05, 2.4665173812009865e-05, 4.707620481503321e-05, 6.311647801194837e-05, 4.488684282424727e-05, 1.2885634548615734e-05, 2.4922302761336312e-05, 2.1431564830585327e-05, 2.786224096563646e-05, 3.020467484373902e-05, 2.054604085520399e-05, 3.169567673791574e-05, 2.0207728536922567e-05, 1.065141938217561e-05, 3.146617247110547e-05, 2.7916144407665383e-05, 1.4918503266654084e-05, 1.779704199661841e-05, 3.234136307047193e-05, 2.1721669900347797e-05, 9.931596116906507e-06, 3.259678771803358e-05, 2.1427156650808268e-05, 8.384285064686837e-06, 1.0228306764216333e-05, 5.611321058406616e-06, 2.207236556629755e-05, 1.3171723022762692e-05, 2.752768826710181e-05, 5.5957918917806525e-05, 4.502029999159639e-05, 0.005619981982229031, 0.011292260760809582, 0.005683551354431588, 4.169306727389849e-05, 2.7117617973734804e-06, 1.4351011125243378e-05, 3.8809428679766734e-05, 1.5026431605937022e-05, 4.477546265331766e-05, 6.044557416810212e-05, 2.17198760471519e-05, 2.9394807773491078e-05, 1.6546392552319972e-05, 2.4304501237231662e-05, 7.978493975242355e-05, 0.00015200741145628816, 8.851111017295075e-05, 4.01574178811118e-05, 1.4405739900073762e-05, 2.763186956702801e-05, 9.968710859956455e-05, 0.00012944367932850922, 8.373195405705675e-05, 2.5275541765656555e-05, 1.0649556422770253e-05, 1.2917727847079208e-05, 5.069113356592643e-06, 2.3994304009489225e-05, 2.187398289490739e-05, 2.096656747147603e-05, 4.423623994969366e-05, 4.1171463397910596e-05, 3.482156326989098e-05, 5.942741930762911e-05, 5.762216782730335e-05, 2.4321721886006758e-05, 5.704237228851119e-05, 4.2162101788859934e-05, 2.0603941385693077e-06, 2.3183737704646296e-05, 1.8358904874439327e-05, 1.8590670877773975e-05, 3.8885496597937974e-05, 5.5762053114025594e-05, 1.4795480266028205e-05, 2.949768542674144e-05, 3.5873556009240995e-05, 1.743836998440714e-05, 1.976981196044153e-05, 9.476564055011497e-06, 2.9238815828459964e-05, 6.449774684554353e-05, 4.207101647278669e-05, 3.142037692906569e-05, 5.299537341734831e-05, 4.633675735520215e-05, 2.3030155931717667e-05, 2.957672935163901e-05, 3.5212076306819656e-05, 8.920359888175078e-05, 0.00010229123186171714, 3.300444707240487e-05, 3.728184837628863e-05, 9.211726462222275e-05, 7.646964959447946e-05, 4.510166130725302e-05, 2.3660451819198002e-05, 7.280570680797218e-05, 0.00010304538586984465, 2.9559511964213285e-05, 0.0005302612178855428, 0.000957086970092551, 0.00039360471273656365, 7.939489173698186e-05, 8.052585547959751e-05, 9.818866379572031e-05, 3.652935902651936e-05, 5.050188736488592e-05, 0.00013718448142148118, 0.0005650845059801568, 0.0006688540170989411, 0.00020038969741937782, 3.5727710854349185e-05, 8.313583611856988e-05, 8.882564867739533e-05, 8.617858072815891e-05, 8.402619438125791e-05, 7.858205505848314e-05, 6.910274162172801e-05, 2.5445264798726963e-05, 3.374198789293683e-05, 8.01833040632245e-05, 7.768312604919405e-05, 6.108191397131242e-05, 2.4075771656088893e-05, 3.7410501260855885e-05, 6.591520518094664e-05, 6.402691133532337e-05, 0.00010847162480758214, 0.00015097701789772215, 5.54900845097092e-05, 5.82925246503782e-05, 8.502563495808675e-05, 9.410116125085737e-05, 5.062652087588863e-05, 4.0084336561493394e-05, 8.765242406699333e-05, 6.069280635502966e-05, 7.656586480117282e-05, 8.11655228618997e-05, 6.747021509081193e-05, 0.00013422141683655178, 0.0001198062145826111, 0.00011684791990073103, 0.00014844152847970344, 7.533987610526805e-05, 9.660461409681184e-05, 8.271380200944031e-05, 0.00010772005891389226, 5.1536215571431944e-05, 7.907349311220803e-05, 0.00011008713821217489, 5.611143506588776e-05, 6.835418850072209e-05, 6.468717931347631e-05, 7.011773167523613e-05, 7.844663236948679e-05, 0.00011517819669445895, 5.112016444436995e-05, 6.622821340550411e-05, 2.9948995853194973e-05, 2.0673669166364874e-05, 7.104805661608881e-05, 3.8231616126054805e-05, 7.757726527849755e-05, 0.00011120353079157232, 0.0001156544499805909, 0.00010321312170049135, 6.859189348948907e-05, 5.0093322970591856e-05, 0.09805481810720634, 0.19607444971142848, 0.09799131522534363, 8.185703633936342e-05, 9.023862981719941e-05, 8.33336613677052e-05, 3.072478653277527e-05, 6.91951632818372e-05, 0.0001193101316893837, 0.00014466470350483788, 0.00011092785548138803, 0.00010875137480783978, 0.00011969914531948508, 8.215402993794012e-05, 7.47869906957124e-05, 7.506346710047723e-05, 3.6922531938318056e-05, 2.798938380465293e-05, 4.476831381615353e-05, 7.397689244431366e-05, 4.251343909200035e-05, 2.125111643631236e-05, 0.00010354912674592199, 0.0001270532559199752, 6.246344224111225e-05, 7.544781595175229e-05, 8.934076974148615e-05, 9.245571713511173e-05, 9.194522743291552e-05, 9.269169948924399e-05, 8.940079122321851e-05, 8.413424002863418e-05, 3.569935933953516e-05, 5.2801825202616964e-05, 8.767393321188262e-05, 3.7093000702971066e-05, 2.0675807126056224e-05, 4.075699404161345e-05, 6.439280412661862e-05, 3.403202221626089e-05, 4.2125591233896484e-05, 5.551201427825648e-05, 1.514552491215281e-05, 7.667450752192568e-05, 6.660014083982042e-05, 2.7945379422364662e-05, 4.771594881983721e-05, 6.384064302783832e-05, 7.260835647492111e-05, 7.661940271132592e-05, 9.111068904890714e-05, 0.00010221905190175964, 4.166199919025971e-05, 2.376701383640949e-05, 3.8650808014525085e-05, 6.076001099427476e-05, 4.5788622084527096e-05, 3.088411725824502e-05, 5.2208172418654514e-05, 4.832997375680953e-05, 8.713855871748613e-05, 7.350415802712401e-05, 4.96541807530671e-05, 9.524379395252615e-06, 5.137184367304492e-05, 0.00010501977699402518, 0.0001420005982818947, 7.17138902652235e-05, 4.082250059735444e-05, 2.930210205538657e-05, 7.806720602514079e-05, 0.00010572842456426828, 8.096781583320538e-05, 9.510101184099318e-05, 0.00012592698016664847, 8.700092065809788e-05, 7.26066698595426e-05, 8.1782888095692e-05, 8.395272671305381e-05, 4.224770711871406e-05, 1.106995608081516e-05, 9.735532011103209e-06, 2.752067047021845e-05, 3.389009402906295e-05, 5.771250370036166e-05, 8.377723533434321e-05, 7.885387480125367e-05, 8.175670855436304e-05, 3.1600655612276425e-05, 3.450598909324276e-05, 4.290939774602672e-05, 2.6669391405114603e-05, 1.68522685967845e-05, 3.067982411031092e-05, 6.618659933038466e-05, 5.890041202681141e-05, 3.3847427911004505e-05, 2.416357143729828e-05, 5.378864338343087e-05, 0.00010485575228436024, 0.00010679460636927175, 6.235105363152511e-05, 3.5083076992758505e-05, 2.107406800742241e-05, 1.3643219728132798e-05, 3.0218836958947234e-05, 9.97024613781021e-06, 7.284950775457467e-05, 5.888651837412118e-05, 3.1798575870669756e-05, 8.158835166962577e-05, 8.962841353592735e-05, 8.585227163170281e-05, 5.5251147437784776e-05, 2.4121475161745472e-05, 4.93902500008769e-05, 1.950784341157193e-05, 9.66089261607798e-06, 6.890657493671837e-06, 3.1691775305223734e-05, 4.984740860185563e-05, 6.80353365408807e-05, 4.635014677054849e-05, 1.1835456329046845e-05, 0.00011900358050276759, 0.0001736711495213785, 0.00010111643667807346, 2.2198435819156723e-05, 2.7245105291417147e-05, 2.8229880152154535e-05, 4.054801820655859e-05, 1.4382785180247931e-05, 1.5969161307833768e-05, 2.2182213282728042e-05, 4.080347943463341e-05, 2.2234539668015663e-05, 1.2084971742605094e-05, 3.4316295494870145e-05, 3.670131560604153e-05, 1.6522860414520775e-05, 0.0005621855389392655, 0.0011356153109112618, 0.0005602914992824028, 2.5748031929675336e-05, 3.234209580549303e-05, 1.8826547170253713e-05, 2.80179066118143e-05, 6.820735393106553e-05, 5.508699792990793e-05, 3.0759346790288734e-05, 7.887914570387843e-05, 6.51701106922191e-05, 1.578292527457717e-05, 5.45020849734267e-05, 5.5694022062020294e-05, 4.6649772844886225e-05, 1.7283341404481173e-05, 1.028135108369353e-05, 5.585402391581478e-06, 4.5837578402369435e-06, 4.147931600126257e-05, 4.0202474065237335e-05, 3.166550631285438e-05, 1.7522614797695876e-05, 3.675341615834371e-05, 5.654836662448283e-05, 2.9684504589810096e-05, 1.8505556776919318e-05, 1.9136672812110446e-05, 1.768687700025057e-05, 0.00010809887977772355, 0.00017157487256434258, 4.833875665458884e-05, 4.8195550082155284e-05, 3.2247474474266684e-05, 2.8672173125613267e-05, 6.0884915638085164e-05, 5.602582274265342e-05, 2.5136238130678358e-05, 3.0415878632626595e-05, 4.543500978571658e-05, 2.7523964958585348e-05, 1.3386469008341228e-05, 5.4481619750101e-05, 4.646549255049017e-05, 1.151712538043073e-05, 2.6594414717295054e-05, 3.9666462427249815e-05, 8.900916346302209e-05, 0.00011184523880524173, 6.472635456014294e-05, 6.293479214924482e-05, 7.90811970183533e-05, 5.072803860129079e-05, 3.564046677987454e-05, 4.455846935125458e-05, 2.9364130445938775e-05, 3.212833041701605e-05, 3.581395252186786e-05, 5.8920552302750855e-05, 6.45996372951413e-05, 4.133376937005957e-05, 4.329886554525526e-05, 5.184334023142847e-05, 2.7424027626615903e-05, 2.0722945412498233e-05, 5.7158264530575136e-05, 5.27154073650942e-05, 1.935031224140796e-05, 3.089144286482608e-05, 6.160386992408601e-05, 0.00014746999328063543, 9.787542838493302e-05, 4.250435285254949e-05, 4.850204772869474e-05, 6.015330509580535e-05, 7.697386154134657e-05, 8.47750856428371e-05, 3.6594004857034096e-05, 2.4634825251164935e-05, 1.2769973518829531e-05, 1.60726077274541e-05, 3.5052709710912144e-06, 1.621976796916352e-05, 3.346264913041568e-05, 1.2827095751445078e-05, 4.6638511347322723e-05, 7.082701936700689e-05, 5.411978136925765e-05, 3.232025031229762e-05, 1.8547067903120952e-05, 2.9654809049573197e-05, 5.0472519607220736e-05, 2.7249092411692796e-05, 9.451239182563512e-06, 4.631696290538907e-06, 2.262099725639708e-05, 3.5427758789188625e-05, 2.6120838986808535e-05, 2.3772028723659084e-05, 3.25285488892181e-05, 5.396220335393653e-05, 4.371666831077389e-05, 2.913937020415729e-06, 1.1783834520303908e-05, 3.372532273285364e-05, 4.006804247953713e-05, 2.4042536866740067e-05, 2.4208066832615308e-05, 1.2362630968953705e-05, 1.350039513060691e-05, 3.7761874154309614e-05, 4.1973610634724215e-05, 3.2691619832150533e-05, 1.920539637566862e-05, 2.7164647213573363e-05, 3.634885030058057e-05, 4.504260711138182e-05, 4.335765403743918e-05, 2.327667301735946e-05, 2.6594993210638327e-05, 3.1133510738257684e-05, 3.926424019641516e-06, 3.078593878537193e-05, 1.7129283213898597e-05, 1.4288716593122456e-05, 6.391391665020673e-05, 6.275392662229087e-05, 3.1276493657505075e-05, 3.9113252308029405e-05, 4.194130558662805e-05, 4.302577350013769e-05, 2.9287255251252534e-05, 2.729791003655694e-05, 6.311314894487285e-06, 3.897728145406585e-05, 5.1268709760377625e-05, 3.576743621063281e-05, 1.0736936807043658e-05, 2.697134551141146e-05, 6.0191721476928825e-05, 0.0001439962378613182, 7.089966737334804e-05, 6.0608715480504826e-05, 7.663653401127794e-05, 2.2968911536415492e-05, 1.407027475189235e-05, 4.2372631474794e-05, 6.323245937576039e-05, 2.6337346366455088e-05, 2.8687019693985878e-05, 4.884782077029467e-05, 6.016658931742248e-05, 4.389443722679097e-05, 4.930099040893071e-05, 6.977151650782863e-05, 5.5062847782042744e-05, 1.6657132584743386e-05, 2.821629144641e-05, 4.8847259024579965e-05, 5.29865574551323e-05, 4.5453031478849455e-05, 2.2119244720076292e-05, 2.4800013316223815e-05, 1.7244631916191004e-05, 2.0701341058876933e-06, 3.681508498315361e-05, 4.301581971641044e-05, 3.0155639925542608e-05, 1.8061751205122377e-05, 2.4458012310502822e-05, 3.666385859534377e-05, 2.719410648094183e-05, 9.719001941892732e-06, 1.3826911660513322e-05, 2.2268447279996255e-05, 3.677061895664705e-05, 5.3049378363271676e-05, 3.607478811996826e-05, 1.3005751564593839e-05, 9.694954308124905e-06, 2.185895734337635e-05, 8.516677512829474e-06, 3.620430988931048e-05, 3.391567764971882e-05, 8.159046876776452e-06, 3.745781123007715e-05, 4.512815914443282e-05, 2.7912897280011637e-05, 6.282926231640148e-06, 1.9329347485299545e-05, 6.382133200139153e-06, 3.4189071423608084e-05, 5.567373548876568e-05, 2.883316748479494e-05, 1.6961771365628007e-05, 2.2433548689378163e-05, 1.5500884645303603e-05, 3.905156707169317e-06, 4.611957830613902e-05, 3.578827199958023e-05, 1.9434597480102564e-05, 3.145357964822395e-05, 6.0484736975962806e-05, 2.697536361348745e-05, 2.2452497062002406e-05, 2.2676833757295275e-05, 8.786566906500735e-06, 1.4643327204809236e-05, 7.9464662053584e-06, 4.735725200129054e-05, 7.234908313674271e-05, 6.235857535880426e-05, 3.257298376787719e-05, 9.296489340621918e-06, 3.1723235638130686e-05, 5.451918428291688e-05, 1.9274835271163513e-05, 3.208928330921603e-05, 3.0647063683683584e-05, 5.6801735726904286e-05, 6.714926749135017e-05, 9.305123346489931e-06, 2.0712052667821738e-05, 2.3774170289866914e-05, 5.6247718898855103e-05, 3.6460059399431974e-05, 3.5769115063194e-05, 4.195369989804205e-05, 5.1997160949290534e-05, 5.2015351379594674e-05, 2.1678348096713724e-05, 2.1570989517678162e-05, 1.643668917006741e-05, 1.4757022221229601e-05, 1.4783226911561635e-05, 1.321318212263641e-06, 3.0210585345182437e-05, 5.874362206721414e-05, 5.3172727899739295e-05, 1.3877898817333884e-05, 3.8161416405948144e-05, 3.3285033624813245e-05, 6.493997417096367e-05, 2.0744213793617707e-05, 1.7290257645911593e-05, 4.623138095352887e-05, 7.312836314927594e-05, 3.5852013981307135e-05, 2.2840578947657882e-05, 4.096748387798644e-05, 7.056071962307607e-05, 5.3285300638257326e-05, 2.6925842188115915e-05, 7.366957294430061e-05, 7.589581552833306e-05, 5.346548466536431e-05, 4.288298371628986e-05, 6.9921308968029455e-06, 3.515772140843475e-05, 4.3415847049174674e-05, 1.5440731614705207e-05, 2.3178370179579255e-05, 1.7201064201752106e-05, 3.1940563673175365e-05, 3.567010618726042e-05, 7.625315156501738e-05, 4.505294839275999e-05, 3.240197868481592e-05, 5.086239154781749e-05, 8.317105708544406e-05, 7.670133023678373e-05, 3.825841464188153e-05, 9.780909580195786e-06, 1.3985552726049318e-05, 2.8404107317782432e-05, 9.08354984816106e-06, 2.0618951098742127e-05, 1.594039511257178e-05, 2.47969765574026e-05, 4.079258554467134e-05, 5.468870777678257e-05, 3.9789393097952594e-05, 2.9647959131283526e-05, 6.997084715111444e-06, 2.631816172707088e-05, 5.078461620016969e-05, 3.593975703226265e-05, 2.751908753889979e-05, 4.2331408471695736e-05, 1.5415829287916997e-05, 2.356877813067819e-05, 5.3643696263827614e-05, 5.692739362717622e-05, 4.051848890519875e-05, 4.89834416669171e-06, 3.175567940302411e-05, 2.1824082193118197e-05, 3.5962746544065484e-05, 2.7732689212500068e-05, 8.948247058813237e-06, 1.2664529158273063e-05, 2.197238997754255e-05, 2.47544186034455e-05, 6.595592224436512e-05, 8.7954064655534e-05, 6.553591357765335e-05, 3.2061190149070775e-05, 2.0521980631400808e-05, 1.858781521375096e-05, 2.517892629824566e-05, 2.5516780842969552e-05, 1.7721279245148152e-05, 4.171770620879201e-05, 2.1864658070805503e-05, 1.2354047953016916e-05, 3.447493793138386e-05, 4.9610847224823115e-05, 8.073958759076097e-05, 0.00011348781046906026, 0.00011644189498858225, 6.19736432250079e-05, 2.6881895641903e-05, 2.0814102764006646e-05, 2.104182003413624e-05, 2.2089285346742604e-05, 6.842510763740099e-06, 1.4641252990510959e-05, 1.764337100429778e-05, 1.8231997929899562e-05, 2.4057659628292184e-05, 2.314952061142295e-05, 2.6892806492727255e-05, 1.5095401338525022e-05, 3.68138033269325e-05, 5.0509583921083104e-05, 5.874545086543323e-05, 2.876727690985915e-05, 5.614637527698609e-05, 5.2096394899762796e-05, 1.7728581574712396e-05, 1.9991682445634104e-05, 3.940282490343328e-05, 2.4510179559949423e-05, 3.852522663189162e-05, 2.060510581985858e-05, 1.9033714508901862e-05, 9.17402159137269e-06, 3.6658441755534646e-05, 2.466397389441931e-05, 4.486953676472393e-05]}
  in  "sampling rate":dbl=500000.0 format="%#_13p"
  in  "RX max amplitude (V)":dbl=1.0 format="%#_6p"
  in  "RX frequency":dbl=75000.0 format="%#_6p"
  in  "TX amplitude\n(peak 1 ch)":dbl=3.3 format="%#_6p"
  in  "TX frequency":dbl=25000.0 format="%#_6p"
  in  "stop":bool
  in  "Tab Control":T2(tab)=enum."Continuous imaging"
  in  "Save spectrum":bool
  in  "Pre-capturing readouts":i32
  in  "Baseline state":bool
  in  "Averages for baseline aquisition":i32=1
  in  "baseline magnitude":dbl format="%0.3p"
  in  "baseline phase":dbl format="%0.5f"
  out "current run":i32=100
  out "current RX magnitude":dbl=7.332822158634302e-05 format="%#_6p"
  out "f0":dbl
  out "df":dbl=166.66666666666714
  in  "N pts":dbl=50.0
  out "mean of last N pts":dbl=0.18767206857641183 format="%0.2p"
  in  "Save":bool
  out "standard deviation of last N pts":dbl=0.001285296995141931 format="%0.2p"
  out "RX magnitude last 150 points":dbl(graph)=0.1885932883138741
  out "RX magnitude over time":dbl[](graph)=[0.18071171426033708, 0.1806295862382275, 0.1805945439666382, 0.18065499912102864, 0.1806672291624708, 0.18068042999091788, 0.18065973956882186, 0.1806512627878157, 0.1806551534633707, 0.18071675128045425, 0.1806581448603021, 0.18061607799288348, 0.18073954056068664, 0.18069537449202294, 0.1807752004118897, 0.18067404932176095, 0.18067504427965456, 0.18077701968666124, 0.1807577166992314, 0.18078053486695478, 0.18066538523977957, 0.18073862826840398, 0.18069523602990617, 0.1807389886746621, 0.18082444371241782, 0.1807765898168463, 0.1807214417904601, 0.18077377886296683, 0.18077125051158946, 0.1807725552143666, 0.1807196322152533, 0.18074920650997867, 0.18071451667318186, 0.18073865692031144, 0.18075885233519176, 0.18072088129522215, 0.18076714322931708, 0.18067290550111323, 0.18073306330655844, 0.18076089616995158, 0.18077162836661828, 0.18082131459574285, 0.1808108615426075, 0.18087100197051845, 0.18074153862778608, 0.18085947146046183, 0.18087775655078359, 0.1808315268826828, 0.18083616926845966, 0.18087509115613135, 0.18080915175640838, 0.18083975477065833, 0.18085815353545137, 0.18084466514728742, 0.18087762137200689, 0.18092203695040435, 0.18086649771817406, 0.1808010293160264, 0.18081952617493618, 0.18082332894230918, 0.18086525416851706, 0.18082482961817548, 0.1808380479541731, 0.18092867783339306, 0.1808022613484011, 0.1808389211535022, 0.1808550361352409, 0.18085929399125278, 0.18094075026877685, 0.18083124043418383, 0.1808101602562139, 0.1808620719540214, 0.1809020985516764, 0.1808974333160103, 0.18093216031637005, 0.18091719370608766, 0.1808749600374749, 0.18097532722564502, 0.18083758735914673, 0.18089137083936033, 0.18093281803710287, 0.1809113682324388, 0.18093278622543904, 0.18090921017478753, 0.180956287719744, 0.18089772845823274, 0.1809290310068297, 0.18093117888625798, 0.18088233438895854, 0.18091213465638142, 0.1809106793814596, 0.18092438367655403, 0.1808818191911428, 0.18085678959311136, 0.18089667059281986, 0.18084724118247505, 0.18094879711244793, 0.18093062459505416, 0.18085138937647854, 0.1809643465876604, 0.18098510853373329, 0.18096845817011292, 0.18097027891432474, 0.18095821809331888, 0.18089935733060622, 0.1810412021855796, 0.1809278969560062, 0.18101007623388052, 0.1809386477311126, 0.18099345228743477, 0.1809503278414204, 0.18097047943498315, 0.18093987316466495, 0.1809393686232731, 0.18095113334994276, 0.18095279383213497, 0.18102818052993064, 0.18096637182298264, 0.18098404668609752, 0.18101940877246483, 0.18092058237260591, 0.1809862478311434, 0.18104725210051414, 0.18099054427757763, 0.18100387919268282, 0.18097619816221233, 0.1809679946055421, 0.18099632198195753, 0.18098101516624387, 0.18107389045503353, 0.18099201651863878, 0.1810831595759299, 0.1810550370560156, 0.18103517831083296, 0.18106079959205265, 0.18102857223279747, 0.1810483046917502, 0.1810567883882256, 0.18105986991681558, 0.1810112068256704, 0.18098897094520977, 0.18104339065356373, 0.18107676843929418, 0.18099960031535128, 0.18108504651173887, 0.18106105552711266, 0.18097471472648952, 0.18107227865970982, 0.18102648839825752, 0.18102474047476058, 0.18107152477911206, 0.1810429071820323, 0.18108219277861543, 0.18104279337648163, 0.18112277208424277, 0.18105492912591267, 0.18108698393336142, 0.18101082775457988, 0.18106132242689724, 0.18107408686462945, 0.18109787452688308, 0.1811270309410559, 0.1810596816470227, 0.18107165405033976, 0.18101853601839477, 0.181041943860035, 0.1811471067448838, 0.18106453783475995, 0.18106447451732977, 0.18113220247680242, 0.18111022528378157, 0.18105242910907188, 0.18107494685415032, 0.18106840837096105, 0.18109183884604382, 0.18102933681871589, 0.18109400408238846, 0.18107291882813167, 0.18104816677643124, 0.18110658490923404, 0.18114429336715906, 0.18114672035892684, 0.18110891414946378, 0.18108561035712564, 0.18109910162645368, 0.18107449957964888, 0.18106596396870311, 0.1810982709548884, 0.18114316734395056, 0.18107227001433596, 0.18107518449872126, 0.18110691187270023, 0.18108053024092616, 0.18115055555070805, 0.18105651195544184, 0.1810857041062547, 0.18105216069249683, 0.18105546542724088, 0.1811470430587457, 0.1811023228771779, 0.18108203475392098, 0.1811704651394306, 0.1811133219832466, 0.18115603819181034, 0.18124293337150355, 0.18118119377864053, 0.18111771129770898, 0.18115042168563136, 0.18110895982974162, 0.18116103844439424, 0.18115954823401278, 0.18115446344655767, 0.18115136857230543, 0.18116424629580893, 0.18116025327181046, 0.18114770725844218, 0.18110873328728236, 0.1811703870570109, 0.18116493210102802, 0.18117228281402123, 0.18121661651212, 0.1811857205010417, 0.1811876430261571, 0.18121230765055119, 0.1810941850490393, 0.18123124157032025, 0.18116968987650456, 0.1811533580457282, 0.18122659518407322, 0.18113790285589737, 0.18114822360131852, 0.18119144769545772, 0.18111422732868557, 0.18116335730590782, 0.18123322057772864, 0.18108787525234746, 0.181130382677336, 0.18118831504630287, 0.18121896989812844, 0.18121602105098356, 0.18118050369106914, 0.18116023508267917, 0.18121514490190396, 0.18118905597018184, 0.1812856704544695, 0.18123193035499363, 0.18122432437052027, 0.18120700295640277, 0.18127247000410734, 0.1811871290645795, 0.18109481481928746, 0.18117820619201447, 0.1811972928444361, 0.18115832927203435, 0.1811914133758988, 0.18113867501487946, 0.18121777534296532, 0.18117495479235898, 0.18114399913806659, 0.18111753215900253, 0.18116563314375045, 0.1811075653300969, 0.1811793564186496, 0.1812604543809976, 0.1811994967952489, 0.18111705938825506, 0.1811484429923335, 0.1811544986858272, 0.181148042386368, 0.1811292640508785, 0.18118909094843444, 0.18121262154021245, 0.18125234645230517, 0.18119229272865164, 0.1812340495224647, 0.18124456618285337, 0.18116828178524547, 0.18122701748432526, 0.1811897161800677, 0.1812037880108952, 0.18118161812124717, 0.18119856634379355, 0.1812003179692586, 0.18128792368006644, 0.18124627172605431, 0.1812787744546825, 0.18121783752988405, 0.18117795797567496, 0.18124109662881543, 0.18115451081226042, 0.18123680538244052, 0.18121670927364622, 0.181231635753146, 0.18128307872666577, 0.18130627971246044, 0.18108737502985117, 0.18128233652026507, 0.18127961943754037, 0.18124666026375025, 0.18121589903357557, 0.18125792403995689, 0.18128614217222977, 0.1811836492653025, 0.18128878565889348, 0.1812911532655779, 0.18122135931034683, 0.18130246991738594, 0.18123706401573514, 0.18128276950728492, 0.18125263915655881, 0.18118740121482518, 0.18126134700654076, 0.1813246571666952, 0.18126858997012207, 0.18127163723938938, 0.18127694378083004, 0.1812466109922302, 0.18128891650960682, 0.18134493158105897, 0.1812680136444105, 0.18129174686590507, 0.18127633257594888, 0.18135523668026268, 0.18130591092021556, 0.18133922088943533, 0.18124486816398053, 0.18124131240080074, 0.1812459167186123, 0.18125504005850107, 0.18123090495522806, 0.1812459412103266, 0.18134618610992032, 0.1811777832252072, 0.18117976305311712, 0.1812402748378442, 0.1812577783845129, 0.18124089929570894, 0.18129145349294096, 0.18131361533212542, 0.18127945335085763, 0.1813007658092286, 0.181239551855934, 0.18134146100181187, 0.1813191686479976, 0.181301720348739, 0.18130645308857854, 0.18121554413344373, 0.1813828962221768, 0.18132307340215703, 0.18133596607425922, 0.18132024954742743, 0.1812416764330517, 0.18135921315380854, 0.18132896639365653, 0.18127083483630746, 0.1812886682064729, 0.1812485139258228, 0.18126396086859536, 0.18123922523982655, 0.18125583162114164, 0.18132450966958616, 0.18129287131508773, 0.1812473366329377, 0.18135237072518717, 0.18130749676600105, 0.1814126424408844, 0.18130876520856778, 0.18137830887006892, 0.1812444743631227, 0.18131603898944149, 0.1813433309254331, 0.1813549202272179, 0.18132670987406274, 0.18132948709553323, 0.18126591514905044, 0.18132330908512004, 0.18128253199202554, 0.18131459827908927, 0.1813071422056732, 0.18124006639524562, 0.18131841434695936, 0.1812908451060215, 0.18127933688953282, 0.18135072676165015, 0.1812457897959418, 0.1813763170063063, 0.18130868866935684, 0.18131201054395538, 0.1812604864428751, 0.1812876319913642, 0.1812514227682337, 0.18129683756681814, 0.18122930990190475, 0.1813519529831781, 0.18134364617894969, 0.1812806618673501, 0.1812953625130372, 0.18130279285938763, 0.181257050348257, 0.1812406777538768, 0.18124170341804335, 0.18130833735892446, 0.18121750044935195, 0.18126300340333829, 0.1813374190384183, 0.18128235954407895, 0.18134325409009053, 0.18129545590440546, 0.18132058745397933, 0.18123898009527215, 0.18132137183239483, 0.18112246701852566, 0.18119189927067675, 0.1813419190259655, 0.18125706724673873, 0.18120632286032132, 0.18120411328034494, 0.18120365008034178, 0.18118574095203802, 0.18117275082702455, 0.18116231925903994, 0.18110746546983192, 0.18113845483494384, 0.1810344452596594, 0.18097097613228857, 0.1808794273233946, 0.18063848066053495, 0.1796385655353898, 0.17659203063866258, 0.17891552393564572, 0.1896492460647321, 0.19036454606183806, 0.19030571303368818, 0.19029426686251275, 0.1900860939427929, 0.1900793487234843, 0.19001735078820434, 0.1899937723160163, 0.18994180670751332, 0.1898898106532242, 0.18986133014282502, 0.18983033435381386, 0.18979537845410757, 0.1897164401789632, 0.1896556865146549, 0.1896140450523229, 0.18966226748499881, 0.18956816251068176, 0.18953844844199116, 0.18956369154842895, 0.189456989945009, 0.18943640388372035, 0.1894231052695876, 0.18947343755851795, 0.18944924617707132, 0.18940091957607377, 0.18936696999747996, 0.18935049395000092, 0.1892481598546331, 0.18933033405993377, 0.18925849429537173, 0.18924571641118, 0.189246769837628, 0.18918710703026562, 0.18917065653973292, 0.18917649270201695, 0.18914676603745967, 0.18913391820564018, 0.1891733459910634, 0.1891182195524257, 0.1891020754480345, 0.1891338018465054, 0.189089402833859, 0.18906094941774795, 0.18906125400604185, 0.18904029860034594, 0.18905078707328601, 0.1889637024051632, 0.18902343966304336, 0.18895852288388162, 0.1890126308317865, 0.18900073503868361, 0.18894650593777337, 0.18895397770001962, 0.18898337764154988, 0.1890377074325248, 0.18893438705148613, 0.1888474577699048, 0.1888163278848133, 0.18880717337626812, 0.18869876523419715, 0.18880871200440286, 0.1887269825400869, 0.18873845756515564, 0.18873551596248486, 0.18876044124381813, 0.18869281233539248, 0.1887877373693509, 0.18879856059314443, 0.1888565495712424, 0.18869844910199968, 0.18872129145072072, 0.18866556740429405, 0.18867756464702545, 0.18870826376874653, 0.18874054708893165, 0.1886969429396912, 0.18874103888738947, 0.18867678161089071, 0.18870087483420697, 0.18868566676305268, 0.18874606734568605, 0.1887248754388333, 0.18873856257242203, 0.18865644249188074, 0.18871107560953287, 0.18869759441889103, 0.18865526859671378, 0.18864157983491533, 0.1887274562646163, 0.18868360903166953, 0.18866200485361612, 0.1886919707692388, 0.18872158094691618, 0.1886833392004735, 0.18867219647168051, 0.18864536901068563, 0.18864463027037487, 0.18863115337482583, 0.18868914244067544, 0.18869882119834655, 0.18875346769804072, 0.1886601713366264, 0.18863726158866667, 0.18866638717427775, 0.18864887264025879, 0.18869750643597463, 0.18868318945472207, 0.18866741287251906, 0.18864170345340014, 0.1885976688696802, 0.18860101764116094, 0.18871192984070997, 0.1886505145603867, 0.18657358725036932, 0.1867940335449478, 0.18680043692216672, 0.1867579490210215, 0.18674910815993676, 0.18668167001641736, 0.1867735552890255, 0.1867299003682922, 0.18680792866496576, 0.1866278832978421, 0.1866902995342341, 0.18662416444121852, 0.18668297294429362, 0.18666326246435358, 0.1866803831958475, 0.1865644993706959, 0.18664105341749562, 0.18654090097138837, 0.18661599599982892, 0.18850144207909247, 0.18852481927557568, 0.18850388870064363, 0.18850608626702534, 0.18853499375352767, 0.18857327690806722, 0.188550245343189, 0.18853110482203927, 0.18860780971782706, 0.18856334432243668, 0.18851516322069825, 0.18855365835092777, 0.18850954896040073, 0.18858784830183065, 0.18846550273494997, 0.18854619392536473, 0.18588264559809173, 0.1858803788754565, 0.18593823209196084, 0.18585896021500212, 0.185871653082074, 0.18577272198981346, 0.18584540524341212, 0.1858363825711705, 0.18582983378459128, 0.18583561132814624, 0.18578199172792284, 0.1857482227754216, 0.18582587163113315, 0.18571073936369822, 0.1857359306750168, 0.18574047415158698, 0.1885203529936169, 0.18851107515624946, 0.1885122388418007, 0.18849939679452804, 0.188548705629937, 0.18856560974984007, 0.18853841603734037, 0.18853799389474174, 0.18859107015588406, 0.18851834911272367, 0.18858177780064522, 0.18853145532174667, 0.18853601877550533, 0.18852293817317237, 0.18856094659566133, 0.1885496318546354, 0.1885565045771865, 0.18855659423777837, 0.1885738237153145, 0.18853666422053394, 0.18859728845397725, 0.18860330526734218, 0.18858225332196057, 0.18857297732725176, 0.18847429562269996, 0.1884941419535366, 0.1885932883138741]
  in  "Start spectroscopy":bool
  in  "Update delay (ms)":dbl=100.0
  in  "stop 2":bool
  out "RX phase over time":dbl[](graph)=[-2.8596571196179235, -2.862323765463129, -2.86170278821058, -2.861828574960492, -2.862011401078119, -2.8616851606405342, -2.8617297413304006, -2.8616772114270757, -2.8612615794852925, -2.861681140167931, -2.8614665053007267, -2.861700640305066, -2.8614172345779636, -2.861444910027151, -2.8615778734579305, -2.861387589517673, -2.862136468645685, -2.861741278051226, -2.8614610323741, -2.861657279303831, -2.8613403747714896, -2.8613999686778753, -2.8617566189053063, -2.8615550756748553, -2.8612651009388785, -2.8614121825019936, -2.8614608030438755, -2.861521560135374, -2.861271805719829, -2.8617442197725778, -2.8615395236398116, -2.8615384443587106, -2.8616648488875076, -2.861619902487982, -2.861627630130816, -2.861563641378739, -2.861590817119336, -2.861757978315799, -2.8612002948202666, -2.8610999011189406, -2.861396138918561, -2.8614135556794014, -2.861101778906441, -2.8615162871593993, -2.8615789276533494, -2.861130159873596, -2.8610259103641096, -2.8612883518958308, -2.8615671513778187, -2.861518975045063, -2.860653454236013, -2.8616107612304393, -2.861474730820532, -2.861527289206144, -2.8609443246783197, -2.861416720953039, -2.860989118830583, -2.860943925964109, -2.861794515489786, -2.861314195146116, -2.8608758560920466, -2.861188283830703, -2.861024867513237, -2.860949675534225, -2.86123020703676, -2.8611869950014523, -2.861228822027011, -2.860891264231838, -2.8609481772966365, -2.8608477997378294, -2.861414801045146, -2.8612655982194117, -2.8609782020031758, -2.8612539965972963, -2.8608906645814622, -2.861171187161276, -2.8611967815705395, -2.861459120961476, -2.8614573683849946, -2.8611157044291686, -2.8609747259528477, -2.8614312426048394, -2.8613158378867634, -2.861185433226435, -2.8609917956670925, -2.8612473449889686, -2.8614415029012843, -2.861338182938724, -2.861319861522479, -2.8613165255399626, -2.861549833332613, -2.8611970035231953, -2.8611692388907786, -2.8611672962280563, -2.861274970717225, -2.8613220918940994, -2.861081861924192, -2.861401734245385, -2.8613093053159675, -2.861066577449263, -2.8610574375182285, -2.8613090715826655, -2.861321966024755, -2.8609403403345564, -2.8615605958068966, -2.8608469035310855, -2.8611336350987977, -2.8612721045079375, -2.861043867532413, -2.8608946109608473, -2.8608553272442543, -2.860964291041657, -2.8613411856607307, -2.8604745655772756, -2.8609023314683975, -2.8611599166425887, -2.861136758049831, -2.8610304789136007, -2.8607142321618175, -2.8608459299788973, -2.8608414741564037, -2.8617119019573996, -2.860690043195053, -2.8610937041468367, -2.860903295320639, -2.8609921298994703, -2.8609086013803537, -2.861283022426353, -2.860977028274479, -2.8618875406386133, -2.861256783731831, -2.861107717827371, -2.8610919749290056, -2.8610117625339315, -2.8606357042428727, -2.8610648200662463, -2.861188028527306, -2.861078673302018, -2.860842269325409, -2.86121911666453, -2.8604638173702988, -2.861145673944098, -2.8610899309255804, -2.8611770298188404, -2.86120616924844, -2.861036231555652, -2.861510621721016, -2.861112713964093, -2.86096675708872, -2.8611828481989687, -2.8611100823263746, -2.860572798499327, -2.860748248476926, -2.8607653769532, -2.8608966880907296, -2.86056760682939, -2.8613153535622944, -2.8608066555176976, -2.861024492993169, -2.860978002908593, -2.8611560415388504, -2.861072673901436, -2.860818355930893, -2.86095431685624, -2.8608740923215508, -2.8614967825805633, -2.8610361290142805, -2.8608187175639106, -2.861041136329764, -2.861236834106591, -2.8612293215276097, -2.861156352807614, -2.8612308004220974, -2.8611978938363514, -2.8609981935508575, -2.861261374186174, -2.8612398877597367, -2.8612945485816184, -2.86122701151401, -2.8612286818908292, -2.861224744788875, -2.8613337250350437, -2.8611805106679173, -2.8610432529427015, -2.860785702321269, -2.8614180002112968, -2.861230654088324, -2.861431014422059, -2.8614931923720794, -2.860986820315221, -2.86123885799673, -2.86119684512977, -2.86118625124614, -2.8607102627684746, -2.8612569663498917, -2.860958333575973, -2.8614619051180195, -2.8612432876580756, -2.8611909183551725, -2.8610787564955356, -2.8610216717323276, -2.861393429469502, -2.8607887917515593, -2.861196080863081, -2.8607208834306648, -2.860772863694099, -2.860966139963485, -2.860884877173167, -2.86130033741333, -2.860990589817347, -2.861317731280927, -2.8608351641116183, -2.8611273281632634, -2.8613260284448394, -2.861352762061404, -2.8610024466965847, -2.8609651292437666, -2.8611468997018514, -2.8610271250576527, -2.860610583974425, -2.861059863021833, -2.86136753167809, -2.8611790521861575, -2.8611502472645816, -2.8610942804839667, -2.8612018197307862, -2.8613980511249384, -2.8611036311931133, -2.860643925848332, -2.8609580324149877, -2.861151538695118, -2.8611192533583374, -2.860655129177655, -2.8612777044193294, -2.8607543885096955, -2.861546569014621, -2.860617248705374, -2.8613094843038938, -2.861007244569941, -2.861125132690763, -2.8614657541293007, -2.8612638861273156, -2.8608158583773755, -2.861075662874817, -2.8610787606704524, -2.8611879066771944, -2.8611586729285445, -2.861221267468657, -2.860777915266636, -2.8614328635086865, -2.8611219817222393, -2.8614581367140777, -2.8612264494171002, -2.860685813556829, -2.861039010042807, -2.8612300296841364, -2.8612019338462815, -2.8618520630414928, -2.8615782653409902, -2.861175162849438, -2.8614018029806974, -2.8614075300496924, -2.861217122381261, -2.8609809592579443, -2.8609841522919783, -2.8611404970457124, -2.861524117940169, -2.861188415115197, -2.861055811194346, -2.861423803421479, -2.8614159541298636, -2.861091105517175, -2.8614986397267783, -2.8611193304372375, -2.8608564131262555, -2.86125703292145, -2.861120435475263, -2.861133801604772, -2.8612071286145278, -2.861215525160664, -2.8610499960304407, -2.861452890939004, -2.861029837856134, -2.86121546978976, -2.861002301477109, -2.860829023312776, -2.8608385200666966, -2.86142178234212, -2.861293354240247, -2.86141992697942, -2.8612743701944523, -2.860476549235463, -2.861164006256009, -2.861279269249068, -2.860801137554809, -2.8613073575837524, -2.86085722804152, -2.8608598746690608, -2.8606832814926015, -2.8605973500929744, -2.8607618316714043, -2.8614576142246646, -2.860992842414469, -2.8612381865379555, -2.861235840647215, -2.8609073987152915, -2.860674036770495, -2.8608554162859225, -2.860945447991803, -2.8609546465087106, -2.8610601263477924, -2.8608428295994877, -2.860982115994759, -2.8613447314570686, -2.861052319988664, -2.8609856094860384, -2.861095350709741, -2.86065654895628, -2.860850690241891, -2.8608421930340375, -2.8609371588191292, -2.8608381239136063, -2.8609100153964224, -2.860882071394383, -2.860923279919965, -2.8608632261247395, -2.861222681218485, -2.861370995677928, -2.8609374266020904, -2.8610838760915276, -2.860958527373827, -2.861261208913744, -2.8611824260537673, -2.861085117524928, -2.861470366169364, -2.8613056968358808, -2.8613518478049476, -2.861153576570214, -2.861318486134273, -2.8609086337657956, -2.861298942574489, -2.8608304030525096, -2.8611117057164885, -2.8610123029449537, -2.8610171105855278, -2.8611708070872193, -2.8611829203364305, -2.861250068198196, -2.8613392348390563, -2.861700337879425, -2.8610211479844656, -2.861335186528882, -2.861012766483764, -2.8609455241124464, -2.861118973826703, -2.8610692741794677, -2.860711356636741, -2.8609405175366893, -2.8611024096358353, -2.86091025971498, -2.861014587204627, -2.8612850547349082, -2.8610274006918845, -2.860962360117887, -2.86093891153352, -2.860868405910219, -2.8608240429681597, -2.8613102564140176, -2.8609280434941935, -2.8612718122451106, -2.8611444642063026, -2.8613035515020293, -2.86073883254065, -2.8610949536079353, -2.8615857347353244, -2.8613156628278684, -2.861303952436204, -2.861230088235236, -2.8611321464518444, -2.8612193922204074, -2.86103140430392, -2.861572419524833, -2.861411523617615, -2.8615374384440586, -2.861315041478173, -2.861519582182388, -2.861761602528982, -2.8618057765520626, -2.8620239500777203, -2.8618286714988543, -2.861809456991183, -2.861777213702431, -2.861732313763203, -2.862110236199369, -2.862144524926653, -2.8617962096173803, -2.8616950384747404, -2.862263472976193, -2.8622825589037797, -2.8620686664164623, -2.8622726426231058, -2.8619493752865637, -2.8620894484330193, -2.861946880754778, -2.8621318757781546, -2.8622369100287157, -2.8620610101855006, -2.8625252952227114, -2.86154888593852, -2.8621821711675746, -2.861978563333011, -2.8624914070943386, -2.8623997221574955, -2.862571622047542, -2.862468419522348, -2.86270363731941, -2.8638499682817335, -2.863614982600467, -2.8623613811761297, -2.8623896572496443, -2.8628302321436343, -2.8625800898868174, -2.8625215042773897, -2.862754160682743, -2.8624280126982113, -2.860143309626619, -2.8577199601399252, -2.852600825797482, -2.842676817093324, -2.889783890051961, -2.988181874182653, -2.994221474937847, -2.994101978023332, -2.9927429076608862, -2.9925962063420597, -2.991667470231598, -2.9908974208716064, -2.9906445487882376, -2.9899030013317045, -2.989009589528313, -2.988633451922044, -2.987988564475887, -2.9872058443563096, -2.9871385037974263, -2.9866682826296054, -2.9862757350493596, -2.9858427443649793, -2.9853196615708226, -2.985391302343089, -2.984619980782481, -2.9844652424411455, -2.9837932597025354, -2.9837930524474343, -2.98335037460759, -2.9831405501862833, -2.98244404257898, -2.9828771251535797, -2.9822741677676627, -2.9820944588566083, -2.9817451005769615, -2.981691176787803, -2.9817897761681253, -2.980906089306404, -2.980607960106911, -2.980444489308288, -2.980607431870683, -2.9797196541955695, -2.980299299918824, -2.9798826144934445, -2.9799208015176157, -2.979356139749316, -2.9791953786945484, -2.9789230075815487, -2.978977884099307, -2.9788820267041904, -2.97862299815012, -2.978257235977707, -2.978335039239495, -2.9782845036725183, -2.978204130609513, -2.977892803419651, -2.9774510666514957, -2.9775448006752696, -2.977635066746888, -2.9773681105998437, -2.977276662171207, -2.977367034248695, -2.974536386561933, -2.9754039379491797, -2.9750815315491637, -2.974960346931717, -2.9747706348208376, -2.9746774569822447, -2.9743670664703385, -2.9746214243708002, -2.9743755437940718, -2.974097187891662, -2.974289645930741, -2.9745357838419535, -2.9738179298592846, -2.9742189232253775, -2.9735436613421062, -2.9735962157963436, -2.973849461985707, -2.9738174804202986, -2.973526165278322, -2.973435228620171, -2.9736813716376833, -2.973345560775806, -2.9733293870582114, -2.9732834124864516, -2.9731986299081425, -2.973018964386412, -2.9732532219129277, -2.9731375436778578, -2.9727564318199007, -2.973178269772945, -2.972778063331446, -2.972805540960119, -2.9727405308630575, -2.9724933171423134, -2.972509257713678, -2.972606913628341, -2.972428500597984, -2.972063825944276, -2.971896827473686, -2.9721319002347446, -2.971961523935226, -2.9719178543275606, -2.9721397561591396, -2.9718461764495325, -2.9715816520103906, -2.9717628855893303, -2.97156479877739, -2.97209387432493, -2.971225002329705, -2.971366174872713, -2.971499769205417, -2.9712159300316814, -2.971520736534657, -2.9715101261263612, -2.9709929318738455, -2.9709202974039304, -2.971394378286905, -2.9565306109150282, -2.9582378613851024, -2.9580179279855705, -2.957866142619506, -2.9575520333780334, -2.95730128219044, -2.957256333507507, -2.9570709558352646, -2.957375363002056, -2.957016744435458, -2.956787353545047, -2.9565347358461302, -2.956570204251436, -2.9564255905248698, -2.956435528938666, -2.9566416338759596, -2.9562901277911893, -2.956319921849815, -2.9560413700196246, -2.9700296876773122, -2.970378981900704, -2.970372887263842, -2.9705197427556493, -2.970149700638254, -2.969815938746915, -2.9700803447209654, -2.9700456148696284, -2.969883295870365, -2.970096431489268, -2.969931891626459, -2.9698313873390734, -2.9696423504716964, -2.9697786431388096, -2.9694415790387025, -2.969318206328848, -2.950826011645512, -2.95022125950892, -2.950524413538848, -2.950369234839547, -2.9502499768949604, -2.9496710384225575, -2.9498318727102313, -2.949132470833036, -2.949840450058807, -2.949260774724531, -2.9495058966040886, -2.9490129266984555, -2.949253037240115, -2.9485393858476674, -2.948967663317832, -2.948405800262922, -2.968934662403142, -2.968807892629948, -2.9690912929416724, -2.968546237415698, -2.969158403532218, -2.968709217214828, -2.96878385307042, -2.9683070172521515, -2.968427266947735, -2.96874899976643, -2.9684554414019453, -2.968444355609964, -2.968268537848087, -2.9684111774260873, -2.968188824728025, -2.968225849223435, -2.968411076168734, -2.967971305646961, -2.968120740704402, -2.968265745454912, -2.968013485111833, -2.9681981536662847, -2.9677744987055923, -2.968124964006254, -2.9681771515253335, -2.967824551462982, -2.968210990658363]
  out "RX phase last 150 points":dbl(graph)=-2.968210990658363
  out "Measured repetition time":dbl=101.1366999882739
  out "saved in file":path=path "C:/Users/MPI/Desktop/tmp.h5" caption="selected path"
  out "Current readout #":i32=622
  in  "Shift delay":dbl=0.018 format="%#_6p"
  out "Projections completed":u8(slide) max=1 scale=0.0..1.0
  out "RX phase over time (1000 readouts)":dbl(graph)=-2.7047178811798154
  out "Imaging time":dbl=1.0
  out "pulse duration (T/2)":dbl=0.0009950248756218907 format="%#_4p"
  in  "Do recon":bool
  out "RX magnitude over time (1000 readouts)":dbl(graph)=0.14278572594648362
  out "Shift current":dbl(graph)=-0.002471926914444426
  in  "Save time\ndomain":bool
  out "Rotary position 2":cluster{dbl, dbl}(knob) scale=0.0..359.99
  out "raw sinogram":dbl[][](graph)=[[0.14278572594648362]]
  in  "current sense type":string(combo)="Imon IECO XPA175"
  in  "Save?":bool
  in  "name identifier":string="test"
  in  "Path":path=path "D:/MPIdata"
  in  "waiting time":dbl=0.8 format="%#_13p"
  in  "rotation duration per projection":dbl=0.4 format="%#_6p"
  in  "pulses per projection":i32=201
  in  "Rotation orientation":bool
  in  "Projections":i32=1
  in  "ROs per projection":i32=1
  in  "Ramping ROs":i32
  in  "Waiting ROs":i32
  in  "Shift stop":dbl format="%#_6p"
  in  "Shift start":dbl format="%#_6p"
  in  "Start imaging":bool
  in  "Shift waveform type":enum16{"None", "Stair", "Ramp"}(ring)=enum."Stair"
  in  "Abort Continuous aquisition 2":bool
  in  "shift delay":dbl
  out "Rotary position":cluster{dbl, dbl}(knob)={309.375, 36.63651315789473} scale=0.0..359.99
  in  "Time domain saving":bool
  in  "shift waveform":enum16{"None", "Stair", "Ramp"}(ring)=enum."Ramp"
  in  "Online recon":bool
  out "raw sinogram":dbl[][](graph)=[[0.0002520344919742642, 0.0002392251901874092, 0.00027427671512168485, 0.00012386443403863617, 0.00012743365849351166, 0.0001747686061692988, 0.0002657033389229414, 0.0003701157289063776, 0.00017216828913243538, 5.233399801548113e-05, 0.0002084394693673602, 0.00023925305089992624, 0.00020018812322713744, 0.0002135896610014819, 0.00019395655841452562, 0.00011420099914828882, 9.589020643281905e-05, 0.00019649691436760417, 5.9091751442979774e-05, 5.844557978420556e-05, 0.00017659848490247864, 0.0001324556778373849, 0.0002119191210536238, 0.0003696931318356979, 0.0002185464337020538, 0.000144340436877245, 0.00021428274555834853, 0.00040222616003528835, 0.00013204878511429346, 0.0002190564720573597, 0.00014935853186356807, 0.0001520577022765577, 0.00020791322776795174, 0.0002678722485329298, 0.00012377117223896442, 0.0001361871124286189, 0.00023292353398679294, 0.00020872313498227453, 0.00016481240606940604, 0.0002839576811193804, 0.00015584916298042248, 0.00011261284628910222, 0.00019770980319029372, 0.00014790439093411854, 0.00013515879420000903, 0.00016025004813855447, 0.00027444516142176425, 8.870043520895435e-05, 0.00010168661615864421, 0.00023878124279189851, 0.00017053496200841156, 0.00023052035441066147, 0.0001261416709536549, 0.0001538730018423611, 0.00017259091215145268, 9.856633688171829e-05, 0.00021021290846389085, 0.0002641220556796143, 0.0004161645379233865, 1.5059465094679794e-05, 0.00024582443183713637, 0.00022905460774567336, 0.0002707153026160613, 0.00023614892945249448, 0.00021692928437576825, 0.0002206694022698635], [0.00011937224785074532, 0.0002719684061273256, 0.00015289039053053994, 0.0002259509134566374, 0.0002647758152804597, 0.0002467066499382107, 0.00017765341836444126, 0.00011471992115914542, 0.00011201341560213609, 0.0001966265735321319, 0.00014834269169334373, 7.399001299090761e-05, 0.00012798850015182723, 4.919641751989194e-05, 0.00017465621145736844, 0.00012180044528953202, 0.0001366633842563154, 0.0002440462551220006, 0.00011522359734736639, 0.00022428101153556098, 0.00026920771171241436, 0.00025979936867439745, 0.00023690626374869823, 0.00021405350346453213, 0.0003317023946335758, 0.0001571755176092315, 0.00022051547230396792, 3.417428968227834e-05, 0.00025529759109221107, 0.0001859832673729814, 0.00021968583640419445, 0.00019447127792396953, 1.7650794982295124e-05, 0.00025231477394449715, 4.590248415427172e-05, 0.00029466956231871135, 7.251005726740787e-05, 0.0002171210396758677, 0.00014336731963410777, 0.00011340335549597944, 0.0002850107133786276, 0.0001756363020400664, 0.00013897426640444051, 0.0003043350691137698, 0.00019029076812396832, 0.00018571307503478283, 0.00029117588709761885, 0.00018971847915850477, 0.00015888654679300723, 0.00018284738632710218, 0.00010550370773963397, 0.0001877960663976608, 0.00013547580000702831, 0.0002816737770652221, 0.00023184969485034218, 0.0002266676885087277, 0.00016699531280656892, 0.0002607136905672485, 0.0002549028565229409, 0.00021811377109800075, 0.0002542756831955996, 0.00026712983228339087, 0.00012564374441126182, 1.1867423791704764e-05, 0.000251365854400131, 0.00018980541681521687], [0.00021101875599463955, 0.00020572186086650752, 0.00032921459953635777, 0.00024121149469453218, 9.905385124060501e-05, 0.00015832802779643015, 0.00019692296461964494, 0.00014947967096184034, 0.00023027052593794698, 9.992366807728154e-05, 0.0002952363253487392, 0.0001506858153328397, 0.0003101639421841099, 0.00013742322942535622, 0.00022881996545133165, 0.00017632180895223957, 5.6807537838283445e-05, 0.00020080206557481056, 3.377050558198256e-05, 6.695288292677049e-05, 0.0002322689577806874, 0.0002061673644257358, 9.231907200196298e-05, 0.0003669498056504682, 0.00023467934046455619, 0.00031306847806288936, 0.00019980644866270943, 0.00013407644635000574, 0.0001128009775864915, 0.0002798581063822435, 0.00031912099294962605, 0.00012071475638412842, 0.00019681181723660128, 0.00022942039215520976, 0.0001694267370459873, 0.00025354358884785655, 5.860646410660556e-05, 0.0002977298608866392, 5.751029707019648e-05, 0.00022550476339647363, 0.0002605513863114075, 0.00039648764703260924, 0.00020059238516525923, 0.0001505638658858161, 0.00024299421620701007, 3.057912923001116e-05, 0.00025067086914078255, 0.00017384323679596597, 0.0002748354188558557, 0.00012577920754872453, 0.00026331002638823377, 7.665885065037568e-05, 0.0003039808471694409, 0.00015568018004269286, 0.00025625422392926654, 0.00015172314683393678, 9.411688269950368e-05, 0.0003240873977255382, 0.0002723581423210947, 0.0002670024039442544, 7.818552650434377e-05, 4.0429437560505375e-05, 0.0001941721608222018, 1.302163503387773e-05, 0.00018150740340902187, 0.0002904369574225654], [0.00020200489264514211, 0.000296096463860825, 5.218598309663571e-05, 3.9536153566544235e-05, 0.0001836495007990095, 2.5490668378822403e-05, 0.00016569049399916402, 5.215689303421203e-05, 0.000149957200979745, 0.00016570121867623988, 5.049694873241188e-05, 0.0001703184440347066, 8.187210489867187e-05, 0.00011683789313346894, 0.00027776120913820617, 0.000119292012426013, 0.00017266802328772454, 0.00037931374642811234, 0.00020495757611646798, 0.00010294875420827071, 0.00013056530445999302, 0.00016716141494897327, 0.0001834901055913139, 0.00017439714962805785, 0.00026977234801867214, 0.00031928584478784145, 0.0003195888285431045, 0.0001683011861999516, 0.00030054679321006583, 0.00023971899557697786, 0.00037838656909142923, 0.00016873488476944784, 0.00012394155843811652, 0.00026578929298701356, 0.0002469067287284912, 0.00021967325020772334, 0.00024377312206525447, 0.0001912478010409971, 0.00017712998683113226, 0.0001669746332538392, 5.36462652658983e-05, 0.00022766440626159856, 0.00024272997110008824, 0.0001960831743411004, 0.0002880831130982354, 0.00021072269056507815, 0.00027468064447588945, 7.831143051971846e-05, 0.00011891594681769671, 0.00032360037423611086, 0.00035076868351735106, 0.0001673592314412177, 7.861547844325284e-05, 0.0001486842617800369, 2.9334014530663342e-05, 0.00017929459609388569, 0.00014154683446862822, 0.0002630526702055203, 0.00018097964009055101, 0.00015817305848877766, 0.0001036760811735975, 0.00013262021230859704, 0.00014586837904252467, 7.596025625684861e-05, 0.00011199734914463765, 0.00015462188020112357], [0.0003498975166676139, 0.0002973863847418687, 0.0003719993816218166, 7.858648303916362e-05, 0.00018804844835352907, 0.000282913760487601, 0.00021001055935868253, 0.0002112537745650918, 0.00023118521058016934, 0.0002927797798678436, 0.00035793889356169916, 0.00025155099222862697, 0.00019940560387648033, 0.00010664746057643955, 0.0001367837003462159, 0.0001520334419423297, 0.0001377815753592892, 0.0003157913558469038, 0.000250729825729532, 0.00019268075033278213, 0.00017483918806171774, 5.161730597567142e-05, 0.0002259241521396099, 0.0001241304005241871, 0.00010058191353420369, 6.752957764810239e-05, 0.00017915241545057132, 0.00010895630513926133, 0.00019470306287751627, 0.0002904642771769316, 0.00012241923582889024, 0.00020292078153773754, 0.0001636900128039699, 0.0001886271584972396, 0.00019856242315715585, 0.00027478232866211185, 0.00010157195712834866, 0.00015144851174585244, 0.00018762025233997178, 9.636999168039638e-05, 8.930162980742315e-05, 0.00023850131857682569, 0.00010842295752267314, 0.00012557952312724718, 0.0002556518135133353, 0.00013762074298890716, 0.00015663183277782455, 0.00018240950589497933, 1.6737839106231343e-05, 0.00033427928407848495, 0.00014608752406417827, 0.00011416568736282396, 0.00011622566810624525, 0.00021075638018343428, 0.00019666031187439076, 0.0002830440199958871, 5.827819747931926e-05, 5.501939584647938e-05, 0.0001658399406780088, 0.0002519700400430311, 0.0001846656041670625, 0.000285412181575088, 0.0001815958057016008, 0.00016159609524099666, 0.00020745568341074482, 0.0001206107293562154], [0.00021150579928310513, 0.00021986575459484537, 0.0003726265648068155, 0.00012110121273136194, 8.891707371801662e-05, 0.000312667191786764, 0.00019952349930438818, 0.0001266377912464029, 0.00011141451831495018, 0.0002495700953521742, 0.0002204776580444092, 0.00018423411472655925, 0.00013340497089380353, 0.00016059030868465334, 0.0002188156956715471, 0.000188171905839312, 0.0002157770807595594, 0.00021093848240571016, 0.00022237452184963234, 0.0002458848600729314, 0.0002643199041127756, 0.000181129323105082, 0.00022869311355971933, 0.0002615801284864831, 0.0001565718444257736, 0.00016563007520725812, 0.00020379291976307053, 0.00011982830646068133, 0.00022422289331560237, 0.00019302723290414754, 0.0003247223667284921, 0.00014133313158078964, 0.0001894881776995954, 0.00019285382813101522, 0.00017940045987657868, 0.000283522993697429, 0.0002843029592009321, 8.870769097035304e-05, 0.00034671934452149374, 3.5125762828703376e-05, 0.0001056541238302979, 6.851720897179962e-05, 0.00017296812829706754, 0.0001355419858681389, 0.0002027467287662181, 0.00015248455365984154, 6.508583281910386e-05, 0.0001563759529196497, 7.804462477160674e-05, 0.00029102365618746174, 0.00034591649436644696, 0.0002189032208116657, 7.737468086016422e-05, 0.0003742451795736056, 0.0001176531635734581, 0.0002269688247275097, 0.00020539994096723104, 0.0002132239699702824, 0.00027962520971139786, 0.00013256791650175951, 0.0001120571779429732, 0.00015349431647708188, 0.0002922443540332294, 0.00031098581969362803, 0.00018759756287828235, 0.00013427733421062622], [0.00038396386476260237, 6.559632922585503e-05, 0.0001647357539794786, 0.0002561175670896943, 0.0002445170395185292, 0.00032677774682878685, 0.0002458176746582054, 0.00021281269147635168, 0.0003104449380773708, 0.0002625483392489122, 0.00018677873249028608, 0.0001346810966485976, 0.00024606037670214705, 0.00020944771973090546, 0.00015376378572616543, 0.0002452488741968373, 0.00019326255826173673, 0.00012094653042906274, 0.00022355868158393662, 0.00018181309172793822, 0.0001724204302685257, 0.00017009656160525943, 0.00027291141402746685, 0.00028747878532492225, 3.973068508454545e-05, 0.0002635455573881934, 0.0002508244565969619, 0.0001571132427913017, 0.00013934172677851063, 0.00019296130596874056, 0.00018286642223934067, 0.0002130094156906907, 0.00012009840508830479, 4.56463549533984e-05, 5.137623529455702e-05, 0.00020614096514605794, 0.00017041953090186736, 9.656633915411619e-05, 0.0002221575713586313, 0.00015467272486744942, 0.00018489739743701106, 0.00012521460345131486, 0.00018593584900800244, 0.00018260763804294156, 0.00024293094855856932, 0.000156730148713988, 0.00015293051454663174, 0.00024157442688324537, 0.00010990080037603486, 9.317531401466753e-05, 0.00011710815426051719, 0.0002287164312256537, 9.421346177750172e-05, 0.00014503360920234775, 0.0002197340895764594, 0.0001388174213561448, 0.00022244746845210555, 0.00013113535657601941, 0.00019012531851081738, 0.0002547130693428105, 8.923499389882032e-05, 0.00016218366364547862, 0.00019994416359080772, 8.577548462270514e-05, 0.00015762816437863648, 0.00016555735005126484], [5.347494022026095e-05, 0.00031673004841145435, 0.00019114246029399231, 0.00021157370889885393, 0.00014298536439558642, 0.00014645211698627127, 0.00017022616695907124, 0.0001516737006045931, 0.00013065065459306246, 0.0001857497338442924, 0.00012833440456004784, 0.0001804040897771135, 0.00014049896006218117, 0.00011238059640190039, 0.000319500503116038, 0.000272210632849516, 5.304144987256627e-05, 0.0003315447791290014, 0.00021707111536020505, 0.0001202181964568813, 0.0003041780568929337, 0.00033730667572916983, 0.00015661197621863682, 0.0002799459314216504, 0.00018865726306267901, 0.00023432042812824395, 0.00015261305747690232, 0.00020944954958920537, 7.868536173582876e-05, 0.0001823070396595564, 0.0003984806288551552, 0.00023548319984967344, 0.00015366188193009412, 0.00010180411850124418, 0.00023015163371665017, 0.00021980734754000606, 0.0003593467119740215, 0.00011157320929783333, 0.00021029792278706285, 0.000276759817771882, 0.00020085931704547484, 0.00025001215004125896, 0.00012124990300701361, 0.00030194983384880227, 8.564066731671638e-05, 0.00028489175868373, 0.00016929236486448512, 0.0001399398560790169, 0.00025398432600783603, 5.5948004189077044e-05, 0.000255856675229221, 0.0001836382779400721, 2.7075455853929512e-05, 0.0001866552134329059, 0.00024712500142893136, 0.000295663909653608, 0.0003252758142243577, 6.904609034879416e-05, 0.00016878344859970303, 0.0003771382358283982, 7.527116938898227e-05, 0.0003187309836020001, 6.913203039714634e-05, 0.00020649110901955922, 0.0001271194443756484, 0.00021046030390424513], [0.00041347274657891486, 0.00010333808018215385, 0.00023970209780756557, 9.968400884529122e-05, 0.0001597584351651507, 0.00015193576771182143, 0.00016937393386256514, 0.00023323874843459623, 4.472708427375161e-05, 0.00018550797257886573, 0.00023003672871576205, 0.00013656386799270226, 8.014188590662531e-05, 0.0003397032810183936, 4.22193263055308e-05, 4.638390912382208e-05, 0.00013580498869606984, 0.000200327250164735, 0.00012454557994070453, 7.195185825113714e-05, 0.00014143481801832077, 0.00013104538170073096, 0.00020912064483801591, 0.0002105670334532992, 0.00014026987348616268, 0.00020279799221540085, 0.00023392764607858995, 0.00024400177061466335, 0.00031724125848123805, 0.0003864432078987363, 0.00019355731822859172, 0.0002495325990684387, 7.710248070289443e-06, 0.00013899642023349116, 8.147854410001723e-05, 0.00021698281435626488, 0.00011480149173725359, 8.482268420570011e-05, 8.977908261050236e-05, 0.00012675659167534962, 6.828574916018078e-05, 7.97996895034143e-05, 9.255994654237313e-05, 0.0001233183416350233, 0.00017082732250297785, 0.000325007737194015, 0.00010239906762479313, 0.00015611052737868057, 0.0002040325661242027, 0.00014732991956501002, 0.00019245240522453605, 6.92733838348965e-05, 0.00031054776478096305, 0.00012378849130372253, 0.00017175298651147757, 0.0002398003473731094, 0.0002143865750347127, 0.00017601076057455211, 0.00028218609038128674, 0.00020361935596331586, 0.00012330665102595382, 7.027367879034552e-05, 5.50769151935929e-05, 0.0002553596674863948, 0.00016992012023568892, 0.0001363595157579659], [0.00020362411386125296, 0.0002652912087903292, 0.00014654077611417842, 0.0003128695729590925, 0.00017333510719528227, 0.00019451013457955332, 0.0003055231969034568, 0.00032190398467257244, 8.303170749510013e-05, 0.00030401430001632474, 0.00022036675024334314, 0.00020434907770253675, 0.0002868243643798202, 0.0002993431526102582, 0.00014202590134591812, 0.00021303348720551265, 0.0004026463232600366, 0.000127991272050639, 2.0286289389858016e-05, 0.00016323647591212805, 6.648340579572122e-05, 0.0001435975601935589, 0.00035064677660120807, 0.00015223955711758265, 0.00033474492779251983, 0.00015637329683641665, 0.00027994854437804755, 4.096130734536303e-05, 0.0002108223797796339, 0.00019378711802132015, 0.00020486708100861007, 0.00037618138023414236, 0.00015228807251757513, 9.45052183012338e-05, 8.207375118149889e-05, 8.294550918886177e-05, 5.1821662785587675e-05, 0.0001431637710295545, 0.0003131530837582569, 0.00023446487780087066, 0.00016812514596494175, 0.00011711626514146226, 5.831287845540081e-05, 0.00023590484038380337, 0.0002269285641337681, 0.00024310896999516534, 7.338247981360298e-05, 0.00021302317427591855, 9.251526226768381e-05, 0.00021691612539974242, 0.0003693813132688302, 0.0002356575889010219, 5.1896984783017115e-05, 4.825459852342287e-05, 0.00018940951786263296, 0.00010251926651204464, 0.0001336097303263307, 0.0002548394446654841, 0.00020478810872992783, 0.0002462008627178753, 0.0002412005492778365, 0.0002337836184208563, 0.0003561930472507815, 0.00021165138537719124, 1.5118419462926238e-05, 0.00012043478385502724], [0.00021418800156153977, 0.00010753858735332461, 0.0003123738485064704, 0.00012163216183043805, 0.00023701376489822348, 0.00010853562749362758, 0.00029900702284947075, 8.601557754289603e-05, 0.00027048761755970316, 0.00015054383908242434, 0.00021602974786056814, 0.0001991337827970168, 7.143986980503157e-05, 0.0001704070390205019, 0.00011954724819324891, 0.00017907255492664902, 0.00015933039944790694, 0.0001785642498617774, 0.00020079771006216755, 0.00010305059857418913, 0.00012371490208438568, 0.00021274884827126404, 0.00010312821384892894, 0.0001772224486238434, 0.0002444251095153567, 6.964994706288653e-05, 0.00022264995650789234, 0.0002897205435271426, 0.00020508425002821302, 5.5240443627243454e-05, 3.8581316539053055e-05, 7.073373285983503e-05, 0.0003275927136823958, 0.00011301761750726653, 0.00017349566606568003, 0.00017322934576877684, 0.0003033553175449023, 0.0001656347360265496, 0.0001968124628955638, 0.0001153081002410111, 0.00021775793279122323, 9.204320247776634e-05, 0.0002737572864736736, 0.00015859670401156012, 0.0001889408258431826, 0.0002853793293512355, 0.0002793693594209517, 0.00017837400668409061, 0.00026143017978139035, 0.0002600086975555779, 5.385815585305511e-05, 0.00010649716773225473, 6.63244870534803e-05, 0.00015376261142434846, 0.0001318581932398952, 0.00012332832676118148, 0.0001610395265185759, 0.00026984280756833686, 7.372927883422066e-05, 0.00015102664974521682, 0.0001646203221074504, 0.0002877852039343774, 0.000186518315446727, 0.00017587788909158848, 9.157997763273869e-05, 0.00024248247862106894], [0.00012190713341317102, 0.0003063080001444291, 0.0002006166516705697, 0.00021158129672810413, 0.00025218316135910756, 0.0002082496764460119, 0.0002366989062343007, 0.00023825539404072804, 0.0003038284893163175, 7.303630751798147e-05, 7.491570497437393e-05, 7.6795485068746e-05, 0.00021205140331909656, 9.029336705098933e-05, 0.000158523259564453, 0.000190098539261227, 0.00016755593456721054, 0.00014731529163458686, 0.00031738147006343353, 0.00011918697974797465, 0.00017423589334926215, 3.1043181747418094e-05, 0.0002971051861863114, 0.00017667747418325047, 0.00019753263181475662, 0.0002667102173796532, 3.83896156607485e-05, 0.0001758786502987496, 2.519717845103413e-05, 2.6048711826394854e-05, 0.00021407602478459774, 9.063278669717704e-05, 0.00023662452535578156, 0.00024266241182820054, 0.0003016058636259916, 4.368460596654394e-05, 0.00018830523578174872, 0.00013474675826064556, 6.37120203463393e-05, 8.464669911743341e-05, 0.00017342305542224245, 6.183505995374773e-05, 0.0001810054984574156, 0.00017884277576353782, 0.00017874125971097866, 0.00016860108252131497, 7.972677629646529e-05, 0.00013844485342165116, 0.00018298059651408727, 0.00014267339090781738, 0.00031628455755270676, 0.0001860085058293014, 0.00012231786028111814, 0.0001929547480117297, 0.00010884207815585749, 0.00015310177368992695, 0.00018024464521440093, 0.00027400936625950815, 0.00023201200026728497, 0.00022820544619627788, 0.0002632754121105999, 0.0003049357008875231, 0.00011226956994085297, 0.00014115417886574112, 0.00021689966925684577, 0.00020294224255247264], [0.00021391927935946755, 0.0001289282427015137, 4.7526408356385516e-05, 0.00010891614406748632, 0.00035698769145506314, 6.36059119081397e-05, 0.0002035151362040064, 0.0002618852121254337, 0.00013254055396619155, 0.00023386650100757126, 0.00035172264738296457, 0.0003467484053142214, 0.0002913419740344722, 0.00015102247648074226, 0.00016796532244088246, 0.00015784047723428816, 0.00017417843733988857, 0.00015666239763866067, 0.0003510110199244796, 0.0001550271175419939, 0.00014057784947509226, 0.0002703210086213272, 3.855063692147461e-05, 0.00017264997244147097, 0.0001527420032498936, 0.0001537582244512635, 0.0002429048282175626, 0.00012563341299608627, 0.00016293732626460362, 0.0002112601963582417, 0.00014225816119471733, 0.0002890700258395413, 5.325522042090415e-05, 0.00015452898503810018, 0.0003016103622942094, 0.0002712945418561776, 0.0001788471477214375, 0.0001946109278809558, 0.0003488714746366663, 6.789453746853486e-05, 0.00019096179076729555, 0.00013396213845903287, 9.44588299294714e-05, 5.464090441848195e-05, 0.00029792451761934265, 0.00034112168024661924, 0.0001894863968571357, 0.00021057253546884796, 0.0001687427247044011, 6.191006730956037e-05, 0.00010118656651461108, 0.00016559181304768702, 0.0001803784476265058, 0.00024038348726813602, 0.0001520620554599467, 0.00028403199596618877, 0.00017610611042690266, 0.00024716645967101544, 0.000102072777712464, 0.00026607790570371437, 9.420870971748731e-05, 5.2259789833838777e-05, 0.0001303844818709276, 0.00010947521404157074, 5.939765927983638e-05, 0.00019384426730232975], [0.00011211280110228875, 0.00015517100513819156, 0.00019698021050293038, 0.00014900196701783354, 0.0001507957379196028, 0.00016091859840710275, 0.00015032902012943787, 0.0002189232348728043, 0.00015177315447213708, 0.00015798911653039244, 0.00022964094290898928, 0.0003705010630059375, 9.969250479072789e-05, 0.0002010089779367766, 0.00010363778265498043, 0.0001330815162233624, 9.551013622224652e-05, 0.00013010103855407758, 0.00034137664948944867, 0.00011904816511703803, 0.0002647803230943665, 0.0002564056329021994, 0.00019033010962000717, 5.0845391446880985e-05, 0.000274840890312479, 0.0002880702674515737, 0.00018898316757821318, 0.00013637803290024645, 0.0001180240106252033, 0.00023797385673021877, 0.00019012303654355518, 0.00015478651531687708, 0.0003985722221542952, 0.00027557208254860795, 5.244736806963044e-05, 0.00016940778889542604, 0.00020581298139680487, 0.00014638422837282895, 0.0001128399263018979, 0.0002527602025723739, 0.00011648200127900636, 0.00022172240094745733, 0.00010897906359450721, 0.00019387657066569975, 0.00015702508578370158, 0.00031199073512514733, 0.00025808015784675373, 0.0003122837198481137, 0.00017707765814096814, 0.0001264304627200105, 0.00017210086342971185, 0.00011418125944659405, 0.00032599766777299295, 0.00016247695626325288, 0.00015926620527590056, 0.0003505507729833773, 0.00020889959030003628, 0.000256989979246258, 0.00021366022130134878, 0.00010272040243045949, 1.9730010021108156e-05, 0.00011869426398124104, 0.00025758390030574286, 0.0002472718640203504, 0.0002767589911410999, 0.0002337680127079602], [0.0002395053245734177, 0.00016855423708686347, 0.00011349701719713033, 0.00029572434992536936, 0.00025153470036565553, 0.00023530100381327648, 0.000236276291615045, 0.00023828344089384478, 0.0001912780808785324, 0.00010142831471095562, 0.00022223829304380993, 0.00021318031371658796, 0.00025853699843502527, 0.00018758871262431693, 0.00024770124663965707, 0.0003480400615633877, 0.00014157225395477487, 9.998947914784477e-05, 2.3697801600034435e-05, 0.00013267606996328641, 0.0001619561343480096, 0.00013033468247923533, 0.0002754291466310944, 0.00023590609292995808, 0.00012534597876850997, 0.00013560184241734604, 0.00020032806987473927, 0.00016500266775503955, 0.00011311793505496951, 0.00011173023040815421, 0.0001187370846254074, 0.00025822640349352013, 0.00019622830524357283, 0.0002134865686084045, 0.00019554065517125765, 0.00012836541507946138, 0.00017204172121994016, 0.0001767837217732019, 0.00019875440207180818, 0.00018639077365631562, 0.00013358407163432734, 3.8091543855946496e-05, 0.00021684339920192524, 0.00021481562242000275, 0.00034910524553510597, 0.000300715173186934, 0.000342992767595513, 0.0002429716577427914, 0.00016915091680880223, 6.833439669399815e-05, 0.0003446724069654124, 5.0788477370729984e-05, 9.313200826822073e-05, 0.0001730202121045075, 0.00020366333513275632, 9.768916338897441e-05, 0.0001680508508711809, 0.0002639196411836486, 0.0003445641270083052, 0.0002758132206009291, 0.00041356155122307273, 0.00023606908663071027, 7.914592271910375e-05, 0.00015970981728955926, 0.00019792137696853732, 0.0001276409363627914], [0.00010027549636222205, 0.00017517925539211937, 0.00011016267506079678, 0.00019239585374086074, 0.0002197595638696512, 0.0004021038246202908, 0.00013138138746964949, 6.210546421884403e-05, 0.00022248945482391107, 0.0002898642511373359, 0.0001560806914650115, 7.184586563769268e-05, 0.0002252005119509021, 0.00013981839025372665, 0.0001065691775239145, 0.00013743039851396504, 0.00012575435530005514, 0.0001703125923722699, 0.00018480011345850105, 0.00021365627388237804, 0.00012191228695386144, 0.00011782246762823394, 0.0002711335419537922, 0.0002993564021799183, 0.0001919491546053182, 0.0001358570461349546, 5.491663238068893e-05, 0.0001761311080420339, 0.0001477054894431699, 5.254046775751607e-05, 0.00010864697640818548, 6.73293302169782e-05, 0.00028954236805298853, 0.0003742267607875452, 0.00019617759171275615, 0.00028267657760481195, 0.00015522544285743992, 0.00036047648707449265, 0.00013046315855736736, 0.0002928399767389843, 0.00013443165547393548, 3.9469012566255177e-05, 0.00016487417212606112, 0.00018142728664163345, 0.00022686094060739604, 0.00010833646837687723, 0.00010396489048275338, 0.0003220333738285162, 0.00023178638194560047, 0.00017985582186066818, 0.00012184826222353973, 0.0003107761609655587, 0.00039247317196270493, 0.0002572089266840132, 2.1737824799400615e-05, 0.00015908750207220697, 0.00019368899273703726, 0.00010999103250866171, 0.0002591220254397075, 0.00022408948362966015, 0.00016102461973846994, 0.00012344482966620207, 7.546010418502652e-05, 0.0003419458788371139, 8.476114755639746e-05, 0.00016533273829081688], [0.0001071959225360941, 0.00019579233628296819, 0.00042078251702261187, 0.0001470661280582238, 0.00025513916104456596, 0.00016864848476597538, 0.0002275469465957082, 0.00010403401800604727, 0.0001970956340435115, 0.00010622535352341603, 0.0001635867193342596, 0.00018284650451609222, 0.00015079961777651467, 0.00019735587569034302, 0.00027415925085164355, 1.2580212838365323e-05, 0.0001355925899744754, 0.0002595590285403571, 0.0001787106109537199, 0.0002458081907220341, 0.00013995128870737702, 0.00029356922709737816, 0.00019309374305244282, 0.0001934750006012583, 0.00020849488412695628, 0.00010091268764540047, 8.206036009874693e-05, 0.0002853846578373628, 8.57851116224766e-05, 0.00012936752533315255, 0.00016944237774460177, 0.00026206708183156897, 0.00026639413247928957, 0.00022531119369108936, 0.000209072008643009, 0.00032836969245078444, 0.0001336236237253826, 0.0002863362904281232, 0.00019380856795401548, 0.00026216233051242236, 0.00022276696406030067, 6.983799340766692e-05, 0.0002105214983553283, 0.00015410073441068025, 0.0003924733805394494, 0.00028143927145069816, 0.00031929749826828076, 0.0002047351279843967, 0.00022213870508467406, 0.00022842634327486212, 0.00022132039672403264, 0.00022995513382737245, 0.00018056382833497083, 0.00011898671344161059, 0.00021329742438586907, 0.0003003356623135767, 9.115450322436631e-05, 0.00015029785995932044, 0.00014286971456182982, 8.03696930026604e-05, 0.0003011449750610645, 0.00014155461361969247, 0.00021570171631748184, 0.00035609015926698116, 3.272090896917208e-05, 0.00011563268234582227], [0.00029435633930748376, 0.0001156715990523805, 8.812306387825728e-05, 0.0003209669042721289, 0.00012589422707003304, 0.0002722836899944156, 0.00015061284947155237, 0.0002188090025646225, 0.00018621590069560303, 0.00013809287837718555, 0.0002779383681654464, 0.0002182155501740673, 0.00022837786246533416, 0.00010747739204354573, 6.629579625295352e-05, 0.00024476669323917336, 0.0002450975212198626, 0.00012230720590135206, 0.00019572863393890123, 8.225929628155127e-05, 0.000261915801550554, 0.0002557329767153307, 0.00011590393664168333, 0.00011193849510099367, 0.00012043941842554927, 0.00014919372500903774, 0.0002088880860604928, 0.0001840334562030579, 8.324230490363637e-05, 0.00022807922933940644, 0.00025369587605486186, 0.00026188668577782447, 0.00019733254304435104, 8.695852923987315e-05, 0.00012719787290916691, 0.0002621746414081519, 0.00023610095173258615, 0.00016577954160433605, 0.00016609218213553892, 0.00019347368546168686, 0.00029522622477438465, 0.0002315784034834263, 0.0001504285347680098, 0.0003311868014689179, 0.0003465967076614175, 0.00034037173198810913, 0.00022043663054169483, 5.458847293845347e-05, 0.00015939377548721692, 9.283462079960531e-05, 0.00032531294760820584, 0.0003571860626770056, 0.00017485424692222415, 9.890001218893979e-05, 0.0002395094401336625, 0.00013574813965483526, 0.00012431052548097685, 0.0002905554753748517, 0.00031112661963444976, 0.00012712106173609047, 0.00027497487609646907, 7.974217260133296e-05, 0.0001872376675200961, 8.02746075763675e-05, 0.0001553251514184199, 0.00023670598929042928], [0.00021587512203119909, 6.484874485462764e-05, 0.00023755474082699972, 0.00022110962612750828, 0.00019973141452872106, 4.967034448230485e-05, 0.00024346990247005513, 0.00017127587010858854, 0.00020591238962016262, 0.0003644173568183504, 0.00015233653911073876, 0.00013755374314831763, 0.00010566727626348876, 0.00016304560347098115, 0.00017177573458055924, 0.00015650044621156193, 0.0002917825898096208, 0.00028730746852701736, 0.0004088002618024239, 0.00016216754348532598, 0.00020914573989234443, 4.657333526610495e-05, 0.00017978702062466364, 0.0001377394877244123, 0.00026169673131062096, 0.0002885604089747442, 0.00010063498702338688, 0.00010331023448669053, 0.00024785164444728866, 0.0002310686197634721, 0.00018828279049457367, 0.00011650823412565966, 0.00011046285606837903, 0.00013027490867138043, 0.00021158837919078803, 6.842196566202615e-05, 0.00016176001641650888, 0.00018091944738453462, 4.012385422313394e-05, 0.00023713254987190856, 0.0001210577460178057, 0.00022384401086627753, 0.00021536167703393823, 0.00015888154848715135, 0.00029366611528393907, 8.14971766544313e-05, 0.0001457801677882983, 0.00018013975862051618, 0.0002290689704345468, 0.00023022175754618425, 0.00025403926587277005, 0.00018061093244558634, 0.00028015961520725063, 0.00010609615470559544, 0.0003316551060937302, 0.00014016841666554224, 8.102601734345943e-05, 0.00016878021775600745, 0.0002574009028853193, 0.00012416550598061169, 6.667208987842705e-05, 0.00019903643526928194, 0.00015393592577287658, 0.00021261766244027648, 0.0001704756077335506, 0.00039571538379501567], [0.0002296362364958285, 0.00014830205813486729, 0.0001086802182550272, 0.00022975398618412492, 0.00028531703515726284, 0.00013384310846415503, 5.0341111651847244e-05, 0.00014680438710875794, 0.00014684874204377665, 0.0002533354509343738, 0.0002351186947526514, 0.00018396043253255756, 0.00011767630395270027, 0.00022525204202680947, 0.0002189953854244711, 0.00011561187996321948, 0.00023453467237471092, 0.0001535478203318279, 0.00028627922714487145, 0.0001817634600260064, 3.9815626281552684e-05, 8.784357805559431e-05, 0.0002316698046751224, 0.00013575355214177914, 4.617182925809603e-05, 0.00011959320454411296, 0.00014741073806185344, 0.00022064723279350428, 0.0001080050142151553, 0.00018919065951937867, 0.0002203821847638718, 0.00022024352569214808, 0.00019797299605020047, 0.00024800969057984433, 0.0001491909727452349, 0.000355167540683687, 0.0002921778655208145, 0.00022594994226972958, 0.00023016957632657824, 0.00010886785726022761, 0.00021996615922765777, 0.00019781517214229066, 0.00010310680606093366, 0.0003959018520985811, 0.00022073961516820703, 0.0001770655159660477, 0.00028522502896823743, 0.00013301316611266827, 0.00024009634432619898, 0.0002032027479979359, 0.00013494011230181187, 8.42135691749183e-05, 0.00020606635684196128, 1.3752091617219546e-05, 0.00018996899973071861, 0.0002548632133336567, 8.163192855245638e-05, 0.00014098538103129182, 0.0001148007936589669, 0.0001229536266393755, 0.00021354159041385993, 0.00015037886433948936, 0.0002495870976780894, 8.772496886996581e-05, 0.00018727620187751858, 0.00012532455715035044], [0.00020798617941945774, 0.00013133720661881703, 0.00011745616601305039, 0.0001035535229083765, 0.0003330265349530744, 0.0001305421613003023, 8.704206217324099e-05, 0.00013173041162385185, 0.00031905557738587273, 0.0001630748027665616, 9.839082637043471e-05, 0.00032546246719608834, 0.00019070705703754914, 0.00028198685498583443, 0.00013954062829202695, 0.0002860775783684732, 0.00022864136575844062, 0.00020646290287218164, 0.0002747366117253661, 9.826947117060893e-05, 0.00020519067466684822, 0.0001459361041416755, 0.00022166282149303044, 0.00013764647551241563, 0.00012982318699692954, 0.00011342262821883512, 0.00026704498281908406, 0.0002796661312281741, 0.00017966780230887727, 0.0002863267352490457, 0.00037252621615447944, 0.0002541705405294019, 0.0001910759514976959, 0.00016619115483703642, 0.00028981633020939453, 0.00017452698751759018, 0.00025470284926015915, 0.00040699170181534715, 0.00020294665117708599, 0.00018240093065706908, 0.00024175002932199855, 9.692640933091182e-05, 0.00014315738949854397, 0.00010153561790235853, 0.00017496221591222568, 5.211891972388272e-05, 0.00021920699694821176, 0.0003056520078623817, 0.0003100805287975374, 0.0004143535781173285, 6.528351164768683e-05, 0.0002526394297502327, 0.00012526671985588084, 0.000112473279420572, 0.00020824345138606106, 0.00015242500135935548, 0.00032024746190228623, 0.00011453683714827475, 0.00018813271212750167, 0.0002172926458837534, 0.0002514400646392744, 0.00014871925062147102, 0.00024847605379368714, 0.00017339116528226314, 0.00023478195527502172, 0.0001466667137845355], [6.134096342826363e-05, 0.0001785847153031786, 0.00016927456449728485, 0.00024357625130527793, 0.00014268916191898868, 0.00019166183931794203, 0.00014771185914420925, 0.00016638856319127577, 0.00015645453760773883, 0.00017135898436727818, 0.00026265211676609765, 8.471395122505397e-05, 0.0001243258103431333, 0.0002667897650025494, 0.00013423973828196464, 0.00013285003042948728, 0.00017157937331795645, 8.624086091117816e-05, 0.00015754883282249795, 0.00013076575265577126, 0.00026242138809145235, 0.00026753508229292346, 0.0002598589631304061, 0.000322888941039104, 0.0002821302054079261, 0.0001688488247141177, 0.0003325880473138452, 0.0002333683106135055, 8.119430688667559e-05, 0.0001530514496160135, 0.00015866590632174741, 0.00027487026318429475, 0.00010604242169219699, 0.00025076621533513663, 0.0002852609459781383, 0.000243527355163965, 0.0003492842537488168, 0.00011552050248608842, 0.00020235281791351344, 7.929572162087816e-05, 0.0001741766298841308, 0.0001356793354739961, 6.65840620060005e-05, 0.00024744490742914537, 0.00021141454485641218, 0.00016018003970745694, 1.957382812254098e-05, 0.0002429774281622478, 6.708069421131186e-05, 0.0002554077557128126, 0.0002686585806835437, 0.0001519459855160178, 0.00010059088786684458, 0.00017598913431131634, 0.0002647594492473439, 0.00017113025441958847, 0.000340204663047452, 7.517906887594327e-05, 0.00023582378037660494, 0.0001758397911119648, 7.653919878298512e-05, 0.0002428774366163319, 0.00017329397134673268, 0.0002651649477531775, 0.00017931078686058072, 0.000281979241185083], [0.00013760239136313625, 0.00027859950432632103, 0.00035097252880626783, 0.0002684307326482456, 0.00022723082702377358, 0.00026258044078561726, 0.00019819749673872256, 0.00022839467796658007, 0.0002678698406242378, 0.0003648795777009287, 0.00014884355167768128, 0.0001578422523549695, 0.00019417398741042405, 0.00024590599830296654, 0.0002371930307183096, 0.0002851358506931702, 0.00023080418755883005, 0.00016069819782378093, 0.00012052673358685614, 0.000382128038300539, 0.00015598824562763748, 0.00016627424591742808, 7.860722673206304e-05, 0.0003805246513237446, 0.00013472053497620034, 0.00017049345172244837, 8.62893872450106e-05, 0.0001230101920381096, 0.00015580146807178455, 0.00023271489252897528, 0.0004079356376055671, 7.146114676101797e-05, 0.0001174754964083839, 0.00035780173525428637, 0.00028700413562255853, 0.00021192080469480267, 0.00044429823893760574, 5.9212398109367014e-05, 0.00025692688166360105, 0.00014985500809078751, 0.00015644296166971434, 8.884399018257839e-05, 4.824205620354887e-05, 0.00016023385742499114, 0.00024084973854940318, 0.00013909115939520842, 0.00015722234429047525, 0.0002081853873442893, 0.00014706450170406824, 0.0002718708144600228, 0.0001390997856101677, 9.347479370232087e-05, 0.00016079657392586037, 4.478987302820714e-05, 0.000135221305409036, 0.00023958850620724506, 0.0001951034952909737, 0.00022492912525256078, 0.0001333085909401691, 0.00019390933441796454, 4.081531000388871e-05, 0.00023462460110947658, 0.00028003663801238397, 0.00020886008487218995, 0.00013988008666582366, 0.00025464567104606215], [0.0002278445145535245, 0.00035985749378283227, 0.0002640891184304369, 0.0001850066765048952, 4.8954762814791245e-05, 0.0001484182672767134, 0.00013018083432321428, 4.087391382336111e-05, 0.0001817872691597016, 0.00024971278319353815, 0.00026892122496215257, 0.00029615809164372145, 0.00017059816693416153, 0.0002117609739944073, 0.00023928090476970894, 0.000249309081166052, 0.00022042409690471585, 0.00035171586920672396, 0.00013310665394211093, 9.069939399311352e-05, 0.00020706017929645882, 0.00028599868075003103, 0.00014605398422893985, 0.00020366328688130032, 0.00025738745939760994, 0.00012783042220198054, 0.0002631802160293458, 0.0002569033608361631, 0.0001737330746384783, 0.00019017899867089286, 9.57745100313453e-05, 0.00023734930326393649, 5.741720172510755e-05, 0.000276896539750326, 0.00018212002088407702, 6.80850887689653e-05, 0.00010160840238258775, 0.0002654885976179928, 0.00012980768760680305, 2.8590038582235264e-06, 0.0001902105727425846, 0.0001733219465787003, 0.00023392385990340264, 6.724762038003263e-05, 0.00017559850013381482, 0.00022569055114673986, 8.576466185761301e-05, 0.00033320840916898644, 7.525615795494953e-05, 0.00017063280424444338, 0.00015050787387926764, 0.00016353916020028555, 0.00012926338071738734, 0.00013387044531620415, 0.0001265790365498811, 0.00014056259941089665, 0.00020045406627514163, 5.5873287860655944e-05, 0.00011073961701118832, 0.00028730310380553674, 0.0001856844460480152, 0.00022555841813801428, 0.00024673309338718916, 0.0002635571825533992, 6.602284477491463e-05, 0.00030743730905621994], [0.00027979350185013775, 0.00011788375155194212, 0.00010500993077176784, 0.00020008516218906268, 7.569629579753652e-05, 0.00022979635199820467, 0.00022814631660982444, 0.00016361316579288946, 0.00022273457705776842, 9.370032340801638e-05, 0.0002149865668507043, 0.00020261415092131868, 0.00010739056562381261, 0.00027644241829260797, 7.64839252803822e-05, 0.0002413457612924892, 0.00011212893689248762, 0.0003565010816734081, 6.68952644359375e-06, 0.000271164226743062, 7.851423810405915e-05, 0.00016398666405561567, 0.00017047307731233642, 1.615944558253179e-05, 0.00013089651947741608, 0.00011831212747061151, 0.00028398758814389646, 0.00013318209635631786, 0.00045795347797704904, 0.00024787476012972417, 0.00019921631222300366, 0.00020610917450028326, 0.0001605173898358449, 0.0003164625850974614, 0.00033772331236294975, 0.00012311959762526483, 0.00010950017767353133, 0.00013515519441898794, 0.0003234225919866282, 0.00026226451530280136, 0.00014279392397975122, 0.0002614055211426866, 0.00010621062159496917, 6.500430128987115e-05, 0.0001685532998793131, 0.00025733323432838357, 0.00010226330687218444, 0.00021759683706384342, 0.00018297610956637385, 0.00028652528405844765, 0.00014825294233867473, 0.00023027238688862442, 0.00018081110033394112, 0.00022291146659494964, 0.00018340331134876803, 0.00032593355834916864, 0.0003098676400418868, 8.978028575509798e-05, 0.00029142221834869893, 0.0002836099268623741, 0.00018433582490808652, 0.0002039313973219544, 0.000147284748121667, 0.00027851806406037344, 0.00029501093139706864, 0.00026068173631896106], [0.00031106336869794467, 0.00014463172005575595, 8.934537995461602e-05, 0.00021376082907999477, 0.0001957301870518714, 8.875900287392326e-05, 0.0004428825414038402, 0.00021759795592440564, 0.00023402437617684035, 0.00013317376358309537, 0.00018859970013873875, 0.0003147580461651552, 0.00014951519595102027, 0.00021740194534969478, 0.00023865927970625995, 0.00025708059992903134, 0.0001345864308479865, 0.00035765748502805244, 0.00013463375050368093, 0.0002665310007014655, 0.00020920224484655752, 2.4557717805522102e-05, 0.0001082462798225774, 0.00018930794388121786, 0.00024917188445040226, 0.0002613851099986191, 0.00019596584641854778, 0.00013692536068715352, 0.0002750546058591742, 3.8694403567461776e-05, 9.354433398704485e-05, 0.00021131914248632917, 0.00020190072272734366, 0.00022823548053327894, 0.00019037361131349104, 0.00012226869492662775, 0.0003667440179744244, 0.0002719601685013388, 0.00014610706657325985, 0.00032315453110267337, 0.00011925448657897247, 3.7437052609132234e-05, 9.43789586675348e-05, 0.0002621216022109447, 0.0002961639581364244, 0.00015278462584184172, 0.0001626088997225662, 0.00015660569725743425, 0.0002306983466085236, 7.809981145952143e-05, 0.0003028550823939565, 0.00026685332054025103, 0.0002557335625084758, 0.00020343398356224994, 7.998031433940808e-05, 4.8408844460270273e-05, 0.00014567580470453234, 0.0002309496410322721, 0.00014105664843915182, 9.984834619080395e-05, 0.00015702836941081127, 0.0002988352031088428, 0.0003186370570832686, 0.0001881341740511767, 0.00023025447099617367, 1.1337325209365225e-05]]
  in  "Continious baseline set":bool
  out "RX phase over time (1000 readouts)":dbl(graph)=1.2344327608269208
  out "RX magnitude over time (1000 readouts)":dbl(graph)=9.741807744388551e-05
  in  "current sense type":string(combo)="Imon Techron7548"
  in  "stop 3":bool
  out "motor pulse duration (T/2)":dbl=0.0011274336283185842 format="%#_6p"
  out "Rotation on":bool=TRUE
  in  "Disable rotation":bool
  in  "Rotation orientation":bool
  out "shift on":bool=TRUE
  in  "Enable shift":bool=TRUE
  in  "Start swinging imaging":bool
  out "Images completed":i32
  in  "Readouts per projection":i32=66
  in  "Shift start":dbl=0.505
  in  "Shift stop":dbl=-0.635
  in  "Ramp ROs":i32=16
  in  "Wait ROs":i32
  in  "projections per image":i32=26
  in  "Number of pulses":i32=6780
  out "Readouts per image":dbl=2548.0
  in  "Max images":i32=20
  out "shift voltage over time":dbl(graph)=-0.0023831443093680228
  in  "Save enable\n(before start)":bool
  in  "Path":path=path "D:/MPIdata"
  in  "name identifier":string="data"
  out "image repetition time (sec)":dbl=5.669999518431723e-08
  out "imaging time (sec, calc)":dbl=15.288
  in  "Patch enable":bool
  in  "Baseline set":bool
  in  "Time domain saving":bool
  out "Rotary position":cluster{dbl, dbl}(knob)={70.3125, 202.53700657894728} scale=0.0..359.99
  in  "shift type":enum16{"Sine Wave", "Triangle Wave"}(ring)=enum."Triangle Wave"
  out "shift voltage over time":dbl(graph)=3.554769813848372
  in  "current sense type":string(combo)="Hall sensor"
  in  "Shift field delay":dbl=0.016 format="%#_6p"
  in  "Stop continuous imaging":bool
  in  "Abort Continuous aquisition":bool
  out "raw sinogram":dbl[][](graph)=[[0.19549226273406128, 0.19538181614559044, 0.19530040464410808, 0.19539359726509595, 0.19538880471847528, 0.19542296055711336, 0.1955502580659331, 0.1954381492244175, 0.19553773212044398, 0.19562191910742396, 0.1956324738402911, 0.1955279533279669, 0.19556186031946823, 0.1956264585836143, 0.19565544746727553, 0.19576355613897797, 0.1956914359248519, 0.1957318600646704, 0.19586291457924251, 0.19599562776994217, 0.19609615896790072, 0.1964833396054637, 0.19720806176532107, 0.19818533747948971, 0.19937328167140958, 0.20067599475410736, 0.20185625389283282, 0.20256128319892447, 0.20276381064588175, 0.20264505087807966, 0.2022118405510993, 0.20175540485207344, 0.20148624197549247, 0.20115991658013369, 0.201303280858969, 0.20163533364282887, 0.2023324142778564, 0.20376565439038763, 0.20580715196119315, 0.2086256528209724, 0.21228532905022168, 0.2153821290241441, 0.21656123416393183, 0.21518533442937238, 0.21253378469606524, 0.2087533142784679, 0.20446499530699538, 0.20054671952815334, 0.19762610623765767, 0.1961257704787953, 0.1953917567781755, 0.195173944295948, 0.19505117616403536, 0.19504185415439634, 0.19510884853872063, 0.19512225400732403, 0.19518503967346199, 0.19539466689757393, 0.19523745351237973, 0.19523899395367322, 0.1953233470308697, 0.1953089826992995, 0.19537033289687486, 0.19529581533722357, 0.19521238163606575, 0.1953097771971158], [0.19545013388052976, 0.1954320949992509, 0.19546170156158363, 0.19546912234703137, 0.19552443655590465, 0.19553181948013829, 0.19560633433891234, 0.19557005354865553, 0.19558794349944592, 0.19565358393470056, 0.19557844290515272, 0.19551636067088263, 0.19565905344377496, 0.1956544031158922, 0.1956853915307911, 0.1957993697577148, 0.19584947115368434, 0.1958851877569113, 0.1959117601139635, 0.19610793267236076, 0.1963936641964479, 0.1970013083708546, 0.19801018804703638, 0.199095734661593, 0.20044142324920042, 0.20162982269900748, 0.2024922180079537, 0.20277866981108203, 0.20277780456973193, 0.20229605980442925, 0.2019021198635188, 0.201462109346816, 0.20146923513018283, 0.20167763577915282, 0.20205797342994072, 0.20280996557358494, 0.20394993846183565, 0.20537948898953431, 0.20717515854158636, 0.20915215795856734, 0.21130459499949755, 0.21285730639390746, 0.21319548794156756, 0.2118901745972201, 0.20919779263160312, 0.20599695926037884, 0.20281985091665405, 0.19998001740622887, 0.19764733975233048, 0.19611909714458112, 0.1953202061637305, 0.19515581192280906, 0.19493729176853616, 0.19501240651460822, 0.19518480102285884, 0.19500622212875782, 0.195167357789126, 0.19507308976091417, 0.19514603340360015, 0.1952488486342525, 0.19523423768842196, 0.19523964843227376, 0.19519892359289545, 0.19525648092214068, 0.19527901452491853, 0.1953625974304368], [0.19553945066922918, 0.19566035763021752, 0.19549800983360524, 0.19554090174580827, 0.19556539780027912, 0.19558926359600418, 0.1955200106641303, 0.19569364627948624, 0.19550550614348386, 0.19562175942974866, 0.19566553343570414, 0.19565752371279652, 0.19565529823840255, 0.19569828355724692, 0.19575614911979883, 0.19589699780045758, 0.19583325634338594, 0.1959473343902328, 0.19598181595192268, 0.1962281475608839, 0.19683498312887607, 0.1975825544759194, 0.1987107842484649, 0.20001875398877406, 0.2012168031727526, 0.20224074842691642, 0.20268417711175116, 0.2027094418759796, 0.20252731213335567, 0.20219690456951334, 0.2018636285363957, 0.2017792797022445, 0.20201642120296096, 0.20228181992296235, 0.20296993261654303, 0.20384046116001642, 0.20496385194932587, 0.20604390852956658, 0.20720332750590154, 0.20850487849036847, 0.20971098558129656, 0.21068024703516167, 0.2109057420594212, 0.21040601402310397, 0.20860673174751945, 0.2061367527013964, 0.2035156979364943, 0.20092245006025178, 0.1986728425694953, 0.19671915430653175, 0.19581091290075878, 0.1953103266611753, 0.1951859705269937, 0.19522045648431152, 0.1951130861863159, 0.19512098751549345, 0.19521202326815063, 0.19517996914388952, 0.19531154528284836, 0.1952334390533388, 0.19535349288717654, 0.19527045245030605, 0.19534167913701264, 0.19528164367391593, 0.19526515200344624, 0.19530926029778528], [0.19557821742101844, 0.19553611751440053, 0.1956020149705838, 0.19555307549927595, 0.19550236030318124, 0.19566908276553047, 0.19562772604603207, 0.19570105621025216, 0.19562313167739187, 0.19570318451085192, 0.19564931638404376, 0.1956773353417936, 0.19575513624817048, 0.1956900534128699, 0.1957666417868161, 0.19575336219661085, 0.19591447374118262, 0.19606653229646043, 0.1962263546256377, 0.19665747279807913, 0.19740863583629667, 0.19840863486031643, 0.19962509081539062, 0.20080416094193254, 0.20199195922097787, 0.202609777862462, 0.20276661551610542, 0.20263321474100193, 0.2024417515771603, 0.20217195349998607, 0.2022534206531523, 0.2024109480383498, 0.20309289936215943, 0.20375843402245342, 0.20457975149253557, 0.20539014519175913, 0.20615366371932894, 0.20670571500549073, 0.20708698875455733, 0.20731696412226064, 0.207590361813468, 0.20766664840107843, 0.20771269106914253, 0.20717764406795802, 0.20615430406608817, 0.20427611854876251, 0.2019952924487371, 0.1999567226598653, 0.1981738894091872, 0.19673330981373588, 0.19577194668349496, 0.19542183279220465, 0.19509308787314342, 0.19500738349434144, 0.19513577551992062, 0.1950917543850516, 0.19516256497912102, 0.19522972057983634, 0.19523026233874338, 0.1952650133536124, 0.195235416758105, 0.19524476117056652, 0.19527327085030674, 0.19533219896113496, 0.19532546243966428, 0.19536981893853414], [0.1956716049819938, 0.19557979838606482, 0.19557141531656272, 0.19565857019176572, 0.19564163919923946, 0.1955800760550643, 0.19565147800110347, 0.19567641940545139, 0.19564699754131884, 0.19578941996878058, 0.19578043250654062, 0.19579747863778604, 0.19590929204161942, 0.19586037945406798, 0.19581269534809526, 0.19590164837805213, 0.19601817709643463, 0.19615409776374226, 0.19646065388378614, 0.19717119705285371, 0.1980172986171058, 0.1990578254586359, 0.20025278396930943, 0.20147866379855098, 0.20227883892164453, 0.20262641635199488, 0.20292237608143596, 0.2028586098746582, 0.20274035301422888, 0.2027108778121989, 0.20299392243389844, 0.20359913646675085, 0.20419584263883042, 0.20471698240332648, 0.20545315211718462, 0.20597902848878627, 0.20634646736338444, 0.2064639677901736, 0.20638489634974452, 0.20634020369840594, 0.2061513345578927, 0.20620152522106175, 0.20636150838648792, 0.20623860909685135, 0.2056100355912695, 0.20432079276385962, 0.20238035374351795, 0.20059257560460123, 0.19893080233627436, 0.19741010826569186, 0.19628388513212158, 0.19563852954863117, 0.1953282783625807, 0.195103062287851, 0.19519227276295803, 0.1952876530832093, 0.19518839961741416, 0.19531434262283978, 0.19534544114318478, 0.19540296634326584, 0.19529713450205366, 0.19534094892351755, 0.19526386547894795, 0.1953492279913631, 0.1953670510243499, 0.1954135534420298], [0.19555973461971607, 0.19558977335419575, 0.19565379049481935, 0.1956117017642111, 0.19566867176575667, 0.19567155028975755, 0.1957709425737125, 0.19567783609829198, 0.19567104907499372, 0.1958646807587309, 0.19573533298022908, 0.19586274007064214, 0.19589469886185715, 0.19593675563462984, 0.19597383185077763, 0.1959629188538957, 0.19609724376071286, 0.19628349613161128, 0.19680431279132898, 0.19750526601126525, 0.19841776814152867, 0.19971235585673922, 0.20090309077618265, 0.2018912484606632, 0.2025941463765954, 0.2029704346043427, 0.2030525888902015, 0.20322383832811936, 0.20335497080624523, 0.2035964422125877, 0.20410544837531594, 0.20468175510219427, 0.2053222342441563, 0.20568711524666364, 0.20601174390950142, 0.20600752996515628, 0.20588608769215358, 0.20562745633903687, 0.20529010458830257, 0.20475732966882731, 0.2045820286661195, 0.20445863418711002, 0.2046103735373898, 0.20454664595824873, 0.2038752662605164, 0.20272055847512646, 0.2010685116252333, 0.19940463501760008, 0.19801717077697245, 0.19694744038508402, 0.1959497274823825, 0.19544050488186598, 0.1952614732647389, 0.1952229745192129, 0.19529035787776944, 0.19523186303941079, 0.19534304153558743, 0.19533479891151934, 0.19529533140511765, 0.19536237713016158, 0.19526292801582892, 0.19533460227091642, 0.19527234286882098, 0.19537748673195257, 0.19536793889186152, 0.19537149022012074], [0.19556168998011536, 0.1956136236816117, 0.1957191028087368, 0.19560034843318974, 0.19570152137667182, 0.1956448759512887, 0.19570437256672374, 0.19563458991662155, 0.1957394229874114, 0.19573352130032035, 0.19579535528343198, 0.19586258850106628, 0.19580310794323674, 0.1958630641383197, 0.19586163412452465, 0.19606722257069964, 0.19626408675398688, 0.1964711949316961, 0.19708743432356818, 0.1979854300270073, 0.19898434321835012, 0.20024793352376288, 0.20141410276686966, 0.20242204494457078, 0.20305864980252883, 0.20354188649812213, 0.20385172141006597, 0.2040261381619223, 0.2043116188580864, 0.2047146878734997, 0.20494254400061468, 0.20534990891721278, 0.2057080131475956, 0.20599673209985161, 0.2060393828038637, 0.20578787061237042, 0.20555719253160623, 0.20505557374816796, 0.20456750271535304, 0.20413982598217034, 0.20394885958205383, 0.20375915291684632, 0.20390911078844698, 0.20400817132462548, 0.20357516584834803, 0.20247388871074032, 0.20116886458364594, 0.19959954493633378, 0.19831016101133025, 0.19723981647775493, 0.19634764779514166, 0.19565080840178184, 0.19535786426900517, 0.19530061576491717, 0.19525173885073782, 0.19536031640916454, 0.19538340008053023, 0.19536511081329563, 0.1954506209265686, 0.1953310761042483, 0.1954608676793766, 0.19536429214735826, 0.19546181778545102, 0.19532286245593158, 0.19533703301724814, 0.19543939656096368], [0.1956495233343685, 0.19559233478479443, 0.19568402770486032, 0.1956688698607975, 0.19573567783307963, 0.19569344735145022, 0.19567212059828012, 0.19576696441241034, 0.1957732035241121, 0.1957518069998699, 0.19581985218654951, 0.1958516677371906, 0.1959182033426052, 0.19590165302257942, 0.19598480895311537, 0.19619385956948016, 0.19638240056262818, 0.19669480823023933, 0.19748572946621892, 0.19839838345205796, 0.19964667067341324, 0.20083743220130765, 0.2020230007239202, 0.20302915594249255, 0.2036970796270424, 0.20422112903088593, 0.20465549735585145, 0.20471570957231533, 0.20497207089860803, 0.20527452164258345, 0.20552025924058193, 0.20587524787500122, 0.20602034053026896, 0.206098078276505, 0.20588584050610398, 0.20547742536761907, 0.20480915380546866, 0.2041770992944929, 0.2036284768383642, 0.20323384063119518, 0.20312369879533845, 0.20312816739238973, 0.20307518122403742, 0.20299636398747875, 0.2023103687383546, 0.20100232906437177, 0.19957625568603568, 0.19832665392579774, 0.19727675624112456, 0.19657275408629082, 0.19575190609098803, 0.19545601308806318, 0.19529693290642003, 0.19527084310988585, 0.19529484347252887, 0.19531764306201352, 0.1953992964116272, 0.1954744105963827, 0.19539530843808, 0.19541023629842558, 0.19537856655226227, 0.19536734309269166, 0.19540495148753542, 0.19536406269927592, 0.19553204800740864, 0.1954699624214713], [0.19572194334305906, 0.1957794035118349, 0.19574449584032025, 0.19583445278606562, 0.1957576139046684, 0.19576427518279768, 0.19582845872425186, 0.19578678780196945, 0.1957562728569285, 0.19587574959676052, 0.19593386776810268, 0.19598436224606466, 0.19604947409849505, 0.19608977636634783, 0.19607214128719475, 0.19627858372753154, 0.1964863077181192, 0.19694476584288187, 0.19776586332151452, 0.19876904335907247, 0.20015412881441458, 0.2016114595203914, 0.20291547615696837, 0.20387046551980664, 0.20472081671584208, 0.20519390832545625, 0.20537884181085592, 0.2053199681576998, 0.20541974164363275, 0.20554349979192627, 0.2059078783210052, 0.20600441998372757, 0.2061437361373141, 0.20635572062632399, 0.20602775854321745, 0.2053216552959123, 0.20458721612584438, 0.20391957576513967, 0.2033118155449042, 0.20297423346410245, 0.2028812125559748, 0.20284213109530502, 0.20284341587971816, 0.20256423699306045, 0.20198650936126444, 0.20089410045955605, 0.19956120690918938, 0.19853489477181901, 0.19745620964513536, 0.19659764672731495, 0.1960077697656232, 0.19553754824708056, 0.19543820376170634, 0.19531400622273537, 0.19540576216826028, 0.19535929170960833, 0.19540788720073987, 0.19540411799663474, 0.19543836627202407, 0.19540086890279038, 0.19541863395333736, 0.1954751932837114, 0.1955466930924993, 0.19554194704341057, 0.19541630827872178, 0.19546869467114503], [0.1958717599960696, 0.19579478209490264, 0.19585907689656365, 0.1957272105733347, 0.19569365722128004, 0.19581416921622768, 0.19581557210443962, 0.19582939705218505, 0.19594569662596875, 0.19590346796369995, 0.19590029410511572, 0.19610734659540258, 0.19601028847734378, 0.19604186109286895, 0.19623541578684753, 0.1963590589094464, 0.19660139522618406, 0.1972682983924159, 0.19806391088136693, 0.19930359217905272, 0.20084918168564636, 0.202381233103685, 0.20379891839863717, 0.20475518070042553, 0.2053457499287837, 0.20557389484506552, 0.20565080945358719, 0.20552366893961324, 0.20553106692101522, 0.20572866651257238, 0.20609967563277845, 0.20650193872946473, 0.2065442572230518, 0.20642526514906223, 0.20579985628997738, 0.20493977543096598, 0.20406589391999286, 0.20336690233098054, 0.20280883822433668, 0.20263050984183775, 0.20268706682219223, 0.20262694489860333, 0.20230372188996468, 0.20154820220565814, 0.20051133332198107, 0.19911790978821856, 0.19797034782538658, 0.1971173172386386, 0.19644286585301954, 0.19590033092961118, 0.19548834884967434, 0.1953253374233339, 0.1954716353751195, 0.1953328117910422, 0.19537126248876777, 0.19541127856185106, 0.1954525200737372, 0.19538829574987265, 0.19552560137911787, 0.19554331559869742, 0.1954462056948411, 0.1954562430832691, 0.19546894613393312, 0.19551939844067803, 0.1954702635019266, 0.1954896038488016], [0.1958544545897466, 0.19586828385333566, 0.19589156519970993, 0.1957967934344686, 0.19581074673945817, 0.19592553233539295, 0.19578869776570546, 0.19592290026760745, 0.19592567502163913, 0.19603289572965157, 0.19601279243754166, 0.19601799078702908, 0.1961461620967549, 0.1961377144408917, 0.1963117823794953, 0.19647789569319793, 0.1967528247780253, 0.19752485394988603, 0.1985189209595054, 0.2000249453209134, 0.20160725560425496, 0.20326549415325165, 0.2045737215159951, 0.20532633581679144, 0.20573523837002558, 0.20577866522433214, 0.20566552064834784, 0.20546780887950555, 0.20574506509153007, 0.20615761258273332, 0.20665705505088866, 0.20703998522863726, 0.20710919092542526, 0.20665223391487886, 0.20605579919394992, 0.20503529914039365, 0.2040220849825147, 0.20325527466911197, 0.20275154592257805, 0.20254046606004672, 0.20250348802871834, 0.20251676744703298, 0.20206391226777787, 0.20122054049038204, 0.200107293260657, 0.19895372051655202, 0.19785553361720937, 0.19712926454999716, 0.1965216411206966, 0.1958935622647422, 0.19553205568669876, 0.19555838577150478, 0.19542225106474215, 0.19556549098874712, 0.1955975507941777, 0.1955180815995767, 0.19548940063741924, 0.19556915622757767, 0.19551499828879018, 0.1955018748623988, 0.1955455336456706, 0.1954625120476559, 0.19553794676160866, 0.19551312219608474, 0.1956065177641797, 0.19550938985569463], [0.19582284090403976, 0.19588879912444615, 0.1958747159812398, 0.19578590533689086, 0.19587920327284677, 0.19590101451355701, 0.19597900138594174, 0.19594054885243728, 0.1959951924629498, 0.1960122452628873, 0.19612457663567923, 0.1961017422658942, 0.19616693357787754, 0.19617995267365124, 0.1963775129040337, 0.19657435951591232, 0.1971850492346625, 0.1979436417877702, 0.19926235907175063, 0.20077260734556474, 0.2024906373131278, 0.20400490007205224, 0.20500846820851554, 0.2055578958404222, 0.20573820669145135, 0.20561088272796918, 0.20538330099183533, 0.20559096676611832, 0.206120646416252, 0.2065998364940158, 0.20736285111422742, 0.2077483204042097, 0.20752246221458948, 0.20687691979643258, 0.20583272772234987, 0.20464471668129522, 0.20387114780990784, 0.20323606181442078, 0.20275809041023374, 0.20252578602569596, 0.2023439179222697, 0.20158399975910518, 0.200743642911267, 0.19941895847572721, 0.19836353293323092, 0.19736972813780532, 0.19669368426224698, 0.19598867565042832, 0.19568049434298004, 0.19563512509591124, 0.19550282664824517, 0.19557164806517444, 0.19556833313719044, 0.19563953640553486, 0.1955857055446456, 0.1956123277869323, 0.1955300203627159, 0.19549977665605922, 0.19557194203935768, 0.19566778413964037, 0.19560174876142494, 0.19564577881226916, 0.1956018643868073, 0.19568263540378808, 0.19557222113266545, 0.19542228524396754], [0.19588639224705506, 0.19586083221832767, 0.19587302984566918, 0.19590858732730215, 0.1958819368087013, 0.1959141802781214, 0.19592328122525365, 0.19588327546865605, 0.19600100185446484, 0.19602927176118917, 0.19606655990728722, 0.19611584097522244, 0.19616747501708448, 0.19632797604085148, 0.19650598006027648, 0.1969387086037985, 0.19751433573346688, 0.1984605584160461, 0.19972176406241535, 0.201290183956671, 0.20291535749188352, 0.20413730281640072, 0.20506684163575792, 0.20547842799789698, 0.20551778534925583, 0.20541503895850521, 0.20555391087478636, 0.20578718490278486, 0.2064568066014357, 0.2074561120897459, 0.20812481830608004, 0.20846937610841068, 0.20825220805553007, 0.20741295621636407, 0.20634703315646669, 0.20506702284284117, 0.2041551961889835, 0.20348864441080144, 0.2030426211363886, 0.20266041896468406, 0.20212431133822614, 0.20131478660331234, 0.20006328065688322, 0.198995924877175, 0.19802525053245645, 0.1972658574279644, 0.19658442352535185, 0.1959509465965461, 0.19569379740612444, 0.19549981729594995, 0.19556550072604786, 0.19559758049867085, 0.19551937443866746, 0.19557472661198924, 0.19559423736838355, 0.19561191479704312, 0.19565373119305876, 0.19559207634235867, 0.19569904397131446, 0.1955687185185958, 0.1956134079560739, 0.1955898931303983, 0.19564508307854145, 0.19561354588744778, 0.1956284890765389, 0.1955831331115866], [0.1958463568866597, 0.1958789419645674, 0.19590953742043227, 0.19589661877117398, 0.19591606962245045, 0.19601584617956513, 0.19596895270143913, 0.19594715695206721, 0.19605965697050326, 0.19615097428917067, 0.19616444298217134, 0.19610142796972926, 0.19622842958247946, 0.1963124443610207, 0.19660738633390482, 0.19706765854211158, 0.1979819418893161, 0.19912415626349605, 0.20049161300013674, 0.20190173971769898, 0.20326399455381897, 0.20434058022478405, 0.20497026527561485, 0.205259957699235, 0.20535837578546956, 0.20537892414191644, 0.2056873233430645, 0.206292908699465, 0.2072171565726776, 0.2081156466639216, 0.20901600033471954, 0.20927367356530188, 0.20878075125763393, 0.20774464959101105, 0.206617212694377, 0.20533556636421973, 0.20426159515859516, 0.20358780374931174, 0.20279955609431988, 0.20180342364081288, 0.20057921335797696, 0.19932248089321403, 0.1982372455911601, 0.19735129293591522, 0.1965401955537252, 0.196030744463701, 0.1956723642798791, 0.19561302527506017, 0.19561407275408685, 0.19567551834980285, 0.19564524090514948, 0.1956667103863022, 0.19563566485236597, 0.19570645125187178, 0.19572572344462622, 0.19568441221610702, 0.19570844857088218, 0.19567896675853924, 0.19565541507936526, 0.19565915134343762, 0.1956559667319494, 0.1955866144573994, 0.19562212277029908, 0.19560579893144678, 0.19570168828658985, 0.1956386121503105], [0.195940677155256, 0.19597613412383896, 0.1959318194139399, 0.1959809179573061, 0.19592752783154063, 0.1959969658005287, 0.1959934999291508, 0.19611119479548988, 0.1960267583416537, 0.1960361228935789, 0.1960938775146089, 0.1962180676669232, 0.19625754911807222, 0.1964900244927408, 0.19691224335314444, 0.19758837602174822, 0.1984315202277232, 0.19948136371682554, 0.20062323985844466, 0.20195698185556704, 0.20317858123749996, 0.2040654946686594, 0.20465898062065496, 0.20494693473830392, 0.2051468407839373, 0.20540414504337268, 0.20604973710883184, 0.20675263709045366, 0.2078715950075408, 0.20883577673514686, 0.20983652135554892, 0.21013399719080972, 0.20978117526147078, 0.2088710357654419, 0.20758334736430936, 0.2062329217166634, 0.2049524156745254, 0.20375020926771045, 0.20250605743251382, 0.20128780408895203, 0.19993825868315312, 0.19868069897418422, 0.19778577092746646, 0.1970270394659555, 0.19637375236126553, 0.19594555605275593, 0.19577046891606836, 0.19568562287236593, 0.19565296132738327, 0.195792877160424, 0.19584309768734265, 0.19584458470711116, 0.19582240709930743, 0.19573318313741203, 0.19590659162324095, 0.19584712271186053, 0.19585559770514624, 0.19571450309661798, 0.1958538957508728, 0.19579175087913167, 0.19572907842679182, 0.1957189320685667, 0.19578095259655165, 0.19567882523143418, 0.19573895153607568, 0.19568448438023522], [0.19583716741193502, 0.19588223112132494, 0.19597285469842016, 0.19603460659594815, 0.19605133072385328, 0.19601127037137123, 0.19587645572458054, 0.19602103286024897, 0.19604795807269065, 0.19601398675220583, 0.19617356902452765, 0.1962739076944452, 0.19638449158709573, 0.1966665077534511, 0.19710497213637937, 0.19788880811405415, 0.1988260546203749, 0.1998731880730205, 0.20117570916374825, 0.20228173884039638, 0.20332291162497684, 0.203881927156118, 0.2045158254475691, 0.20480287830591049, 0.2052232156573071, 0.20570290348036688, 0.20634648044685466, 0.20744755947429874, 0.2086743055792497, 0.20983676187117994, 0.21087102300926416, 0.21113723342948387, 0.21068646910825953, 0.20969649540032587, 0.2082753045065102, 0.20653273403236322, 0.20462627798338673, 0.20265171870022197, 0.20070963716292453, 0.1991187247089967, 0.1979952600562779, 0.19706220010983894, 0.19630528016223142, 0.19596692842067429, 0.1957146880767778, 0.19574324288623848, 0.19563091750203168, 0.19570888231865446, 0.19573761365623538, 0.19580216665197855, 0.19586773366175997, 0.19586771172027156, 0.19580021672504425, 0.19580377512823155, 0.19581670445607446, 0.19581348746990884, 0.1958118927919954, 0.19574080361521973, 0.19582119350618835, 0.19580630565086712, 0.19578542087878656, 0.1957344506910497, 0.19586163351774488, 0.19567091102999684, 0.19574920580923508, 0.19577814956041442], [0.19578133150386356, 0.19595849466571508, 0.1959753345127492, 0.1959244156004831, 0.19591885765427364, 0.1961011390666176, 0.1960322836801786, 0.19592788129629712, 0.1959624101420403, 0.19600364123938957, 0.19611316997341624, 0.19624831456367942, 0.19634818711922658, 0.1967206044704017, 0.19724261825655726, 0.1979584088167016, 0.198791407608125, 0.19996358752811283, 0.20107456722764305, 0.2021781192914683, 0.20308877178119128, 0.20372915070455858, 0.2042585660617817, 0.20463069576667842, 0.2052036503745199, 0.2059176998586735, 0.20677349790446722, 0.2080192600546677, 0.20945353239887826, 0.21074416653615421, 0.21187162411320226, 0.2124299115532118, 0.21202210548076564, 0.21097999976349555, 0.20918555872710776, 0.2069644297252227, 0.2043670706116968, 0.2019695463532055, 0.19999104137892365, 0.19854690642210512, 0.19749689222778555, 0.196662169169937, 0.19612952074647177, 0.19591241015195335, 0.19584361103383288, 0.19577597557626378, 0.19594418630099236, 0.1959084396850241, 0.1958967983438435, 0.1959815666352245, 0.1959574390739173, 0.19591678341496185, 0.1960104564903604, 0.19600533272502288, 0.1960373519462258, 0.1959481390071381, 0.19598905573203929, 0.19586574986355007, 0.19583129273117028, 0.19583284402706624, 0.19585972812916147, 0.1958565161297468, 0.19582707638473532, 0.19581627030060308, 0.1958472067141843, 0.19583257299177068], [0.19591475326353802, 0.1959263908161005, 0.19596499723034472, 0.19592676378958743, 0.19610252726516922, 0.19601663016896764, 0.1959997291931047, 0.1960777164235078, 0.19612442754995965, 0.19609200199442398, 0.19617118731426567, 0.19633197952688186, 0.1964915609382948, 0.19682974264029807, 0.19748095034670676, 0.1981802376646756, 0.19925472730678018, 0.20024894054780748, 0.20136473825520848, 0.2023536750015567, 0.20315261410144567, 0.20372725226340518, 0.2043081937023146, 0.20476237466112848, 0.20544158087428452, 0.20636239085361843, 0.20752074082591376, 0.20902283061626345, 0.2104431216009846, 0.2118117648400966, 0.21297455546049449, 0.2133646468161322, 0.21282794686111342, 0.2112430093646763, 0.20852544051114788, 0.20553131255484824, 0.20259479770932812, 0.20012024825173602, 0.19823005583333778, 0.19710243566460445, 0.19625821594204443, 0.1960949036012485, 0.19579940340083313, 0.1959240132522234, 0.19590301625565654, 0.19597155201828798, 0.19599273030244002, 0.19591441236451798, 0.19606355567747114, 0.1959421481238774, 0.1960115309608997, 0.19602782743037064, 0.19592417458055, 0.19599163316860224, 0.19593047418816273, 0.19590668886156662, 0.19580276506255737, 0.1959277981743506, 0.19590910844205453, 0.19592980542395746, 0.19581535010123552, 0.19573431080867718, 0.19567388842530378, 0.19575635310917583, 0.19574961349797146, 0.19578564634038395], [0.1959506896156131, 0.19592470902513215, 0.19594898578594144, 0.1959522649311971, 0.1958952314459901, 0.19591156626455095, 0.19602581202009245, 0.19603443749186317, 0.19610171086284853, 0.19602176281806977, 0.19610971747375003, 0.196115799878689, 0.19633799196553373, 0.19676628296317464, 0.19719345488226253, 0.19790530536902146, 0.19889725409901102, 0.19995138088529363, 0.20124992830713, 0.20230821629284684, 0.20330438058687106, 0.20391044134828784, 0.20445260205091736, 0.20517761953318644, 0.20593452937445486, 0.20700430920831336, 0.20843413384686263, 0.20999676209149748, 0.21149014631640173, 0.21294045878933088, 0.21380173230647675, 0.2137394360009825, 0.21269237919378264, 0.2107341707386367, 0.20797031479560646, 0.20498546040183183, 0.2022608486606614, 0.19981032827254636, 0.1979672552605319, 0.19696673199842685, 0.19638206998172916, 0.19624109625709105, 0.19612519363743008, 0.19612705725575302, 0.19615846268602571, 0.19608882215431583, 0.19605374548131574, 0.19609506224802511, 0.19616715881822458, 0.1962003374229375, 0.19617538686231473, 0.196231299524568, 0.19610883867602208, 0.1960306101223107, 0.19608904015066245, 0.1960313990370314, 0.1960802518943368, 0.19602784130231532, 0.19600367683012546, 0.19592864934957643, 0.1959382783518424, 0.19594280616185236, 0.19595644586565328, 0.19594224818161068, 0.19582608676698635, 0.19582731818606205], [0.19593038474616883, 0.19597524285640125, 0.1959661469134497, 0.19601089600896254, 0.19600419818666492, 0.19609339784396426, 0.19604669677091852, 0.19608516539247947, 0.19604751934092174, 0.1961191941440965, 0.19612810183751506, 0.19624710857866756, 0.19637618605664034, 0.19680856663845278, 0.19730856274038003, 0.19812443594823304, 0.19904908524930984, 0.20017378471998803, 0.20143060604727805, 0.20259681255571532, 0.20349928344891152, 0.20421654441891618, 0.20502494554153822, 0.205766151251103, 0.2067028613043059, 0.20810536921982514, 0.20967037931593646, 0.21143296735775252, 0.21291102827544495, 0.21376787821374738, 0.21357445739402175, 0.21255377795999456, 0.210788348026082, 0.20854152211721827, 0.20597776070380905, 0.20336163015402053, 0.20106810284161894, 0.19909829252151043, 0.19791717849172996, 0.19691208633204016, 0.19639066450480597, 0.19622852506853508, 0.19613078816412172, 0.19609942711506767, 0.1961011567864362, 0.1960181549290901, 0.196087512213321, 0.19600991487483319, 0.19611511490076258, 0.1960212519120363, 0.19611341258736956, 0.19602159989734952, 0.1959933290682106, 0.19605763380621352, 0.19613106232875943, 0.19603396474115697, 0.19601412452486344, 0.19601579427331253, 0.1960552403975275, 0.19587304982835418, 0.195843386217069, 0.1959237528385215, 0.19587795345314832, 0.195808011626421, 0.1958914324859299, 0.19591656646084646], [0.1960481034319594, 0.19593576466014415, 0.1959685661346937, 0.19601479810122255, 0.1958616671637085, 0.19595395075242492, 0.19599759317915721, 0.1960375234388699, 0.19609697992119596, 0.1960712564041331, 0.19607655294607643, 0.19612829870676515, 0.1962719429625012, 0.19636873215381104, 0.1967430222951325, 0.19736933577910687, 0.19818007164136442, 0.19934406284612724, 0.20092081224421085, 0.2023882312305243, 0.20382611917524218, 0.20521783642720864, 0.2062898506778971, 0.2073083320572061, 0.2085682611953272, 0.21006543930940869, 0.21148556893653458, 0.21261567812290094, 0.2132795779775117, 0.21297511815397727, 0.21182685852496763, 0.2103414175305243, 0.20875917828853674, 0.20689984485450671, 0.20503307227154946, 0.20343771710233233, 0.20158673067995228, 0.20004519505702595, 0.19877584302362317, 0.19767692062866715, 0.19700293807571173, 0.19661244175926632, 0.19640305253042303, 0.1963182483136667, 0.19645490034941485, 0.19634266938341383, 0.19621739301636196, 0.1962597319778938, 0.19626504347247847, 0.19622472275137645, 0.19624162361747322, 0.19622410917244285, 0.19618074528165452, 0.1961920484870725, 0.19612319613294507, 0.19609060389155908, 0.1961263759886187, 0.19622660141489018, 0.1960812904380945, 0.19605696028082828, 0.19599002456267706, 0.19597571697018248, 0.19605541550083266, 0.19597258331108444, 0.1958732026011546, 0.19586188584795075], [0.19595929288651415, 0.19611364568613818, 0.19613992374934303, 0.1960408622277184, 0.19597595858511177, 0.19605469195650932, 0.19608496136293324, 0.19609357409746125, 0.19617343990467137, 0.19613303432567528, 0.1960817144755744, 0.1961631286675147, 0.1961837906906616, 0.1963325617132317, 0.1967171049835478, 0.197343462807233, 0.19817861242578022, 0.19954255352011285, 0.20096567423442158, 0.2027233878519329, 0.20439143131423224, 0.2058881825158029, 0.20742478554664706, 0.20891645325218797, 0.2105721200945035, 0.21197352875421158, 0.2130532710043032, 0.21320070733361393, 0.21237543165011516, 0.21090402685959664, 0.20909745966629167, 0.20734461299257934, 0.2058863897788149, 0.20478769045184295, 0.20388552641044932, 0.2031339976641677, 0.2022661962914156, 0.2008646883429055, 0.19967293765833366, 0.19841419109206948, 0.19755520054029585, 0.19696718985071973, 0.19665314904648068, 0.196348893517311, 0.196304778756493, 0.1962119117495348, 0.19613585443919043, 0.1961148882787771, 0.19626286271895585, 0.1961892507026727, 0.196194234217203, 0.19618248322967788, 0.19610470560171558, 0.1960567119013606, 0.19615417112569022, 0.1960237219605578, 0.1960286554585883, 0.1960206838553716, 0.19599629581624112, 0.19594759284816632, 0.19601954807744032, 0.19597373645862792, 0.19592952878817657, 0.19604504262629072, 0.19590962030196826, 0.19586610939458612], [0.19595577100047482, 0.19595292626376007, 0.19597280767273012, 0.19608515175292895, 0.1960281363148339, 0.19608304760207793, 0.19610465154674356, 0.1960522057854947, 0.1960348293318492, 0.19603239531660765, 0.19595743856103545, 0.19598246410583742, 0.19595892582159619, 0.1960167993149684, 0.19613369087835272, 0.1964604187895999, 0.19707919200485977, 0.19811473883469902, 0.19977690029394474, 0.20190279188456528, 0.20439589488168794, 0.20716049955456534, 0.2100421747754471, 0.21238366298842692, 0.21398251254504824, 0.21464389032278985, 0.21406024205619525, 0.21245025745920948, 0.21043806092738734, 0.20829933399867992, 0.20629341016644479, 0.20477598879731415, 0.20408435427253493, 0.2037562997777192, 0.20378145914377968, 0.2036367064942779, 0.20290136883848553, 0.20202035218545036, 0.20073953700108832, 0.1995023879475032, 0.19838770955570295, 0.19744527653113686, 0.19699016620576168, 0.19666717692767932, 0.1966101936284767, 0.196422569968803, 0.19634803013323618, 0.1964482968089485, 0.19641116311908177, 0.1964079073863263, 0.19633242537840212, 0.19638809687603337, 0.19622462899837795, 0.19616628949209663, 0.19622144961682567, 0.1961884053343267, 0.1961940416368379, 0.19615026288686888, 0.19618901482768603, 0.19603013506878103, 0.1961234183035605, 0.1960347784092191, 0.1961287697997803, 0.19605663132873072, 0.19593885045760479, 0.19591230332277693], [0.19594214390854306, 0.1960382834622088, 0.19604675141170042, 0.19600086094241498, 0.19606833475024718, 0.19610782736360094, 0.19607761571947954, 0.19609971239134966, 0.1959477718069195, 0.19605665301292569, 0.1959728488564801, 0.19608334353897014, 0.19611274226677677, 0.1961131456120073, 0.19609401034325724, 0.1964442958164298, 0.1968773643867127, 0.1979392889934673, 0.19970345448052218, 0.20203781065074405, 0.20497449678539745, 0.20845804226864204, 0.21202236704969638, 0.2147953957139474, 0.21615242605980076, 0.21560421480325878, 0.21362994951289796, 0.2110399430160159, 0.20818560608718978, 0.20546365923693327, 0.2037684445542226, 0.20283948921617562, 0.2027881314578744, 0.20310199556361092, 0.20332581237979352, 0.20357187552124428, 0.20345316689007584, 0.20258174942639887, 0.2016837007206616, 0.20039989314035947, 0.19914424596261623, 0.19819741840630375, 0.1974128521822412, 0.1968686371637649, 0.19652847217586855, 0.19652201922635457, 0.19626055020571018, 0.19629912282153358, 0.19626361031452605, 0.19631360015475155, 0.19624639779314115, 0.1962008015866515, 0.19620181692527994, 0.19623674839119112, 0.19619657300623738, 0.1961992859827329, 0.19604886786062448, 0.19608852021717993, 0.19601291691266626, 0.19607500222294563, 0.19604126032353061, 0.19619232999113517, 0.19597713782673987, 0.19602124432051762, 0.19596836299086293, 0.19611288355742063], [0.19601591240561209, 0.19599590618319318, 0.1960733686059497, 0.19601209949720194, 0.19601997205492486, 0.19596210406779974, 0.19600573039429073, 0.1959852339649686, 0.19605401364957264, 0.19596404438356968, 0.19594354837792005, 0.19598430763203983, 0.19583433492709873, 0.19578395565220325, 0.19598840104743587, 0.19591565915726372, 0.19617537579202068, 0.1967908096224551, 0.1983020473220914, 0.20092784249825463, 0.20476880270310718, 0.20923225873660994, 0.21347991155369603, 0.2167028996172919, 0.21787843788877628, 0.21652011942592614, 0.21341498468459486, 0.20976019864039047, 0.20632134423263604, 0.20400762639379702, 0.20276749069743255, 0.20207188664286066, 0.20218337700241734, 0.20250860592992825, 0.20299119184708658, 0.20335862441070432, 0.20361128343633716, 0.2034709581680691, 0.2026980294598547, 0.2016384379954871, 0.20031173514814213, 0.19908750986126286, 0.19809062392746554, 0.1972920082949514, 0.19689954103822757, 0.19670421622979617, 0.19660430705889476, 0.19641626134225149, 0.19649238772585137, 0.19641838460269453, 0.19641491269690475, 0.1962912573826464, 0.19648969380691314, 0.19628622241111043, 0.19625983662060345, 0.19621900124344785, 0.19632017095571314, 0.19626684599531544, 0.19628143749878013, 0.19629781046317207, 0.19609819178368174, 0.19621794629765021, 0.19611991915435475, 0.19628516870411516, 0.19617087171035327, 0.19606811927622209], [0.19609664050938977, 0.19596061146776292, 0.19605512767769925, 0.19609498310543347, 0.19607712481052728, 0.19606834284008598, 0.1960067246896819, 0.19595679772495048, 0.19604140635346815, 0.1960073002372908, 0.19597160783713424, 0.19592883921350193, 0.19596400110513712, 0.1959409001199755, 0.19583021136487597, 0.19600312185726693, 0.19621635213335983, 0.19683623695244767, 0.198362300105355, 0.20130096300545905, 0.20554382881809277, 0.21014504061570236, 0.21401757068887794, 0.21679702758512703, 0.21755922252825802, 0.21590910769409977, 0.21254037204884857, 0.20844471792987276, 0.20536872944652934, 0.2033768313848089, 0.20233853216151929, 0.20188064336982692, 0.20183510216426756, 0.20203836186605573, 0.20236607745426963, 0.2029366262474682, 0.20337773450538, 0.20351850153252976, 0.20318441993550884, 0.20254151477361024, 0.201308418413794, 0.20002886520166432, 0.19880170914960874, 0.19794414437966973, 0.1972733997836439, 0.19692182101197514, 0.1966544894498799, 0.19656746894901833, 0.19642425452474221, 0.19650503296652955, 0.1962830147092313, 0.19625233116164126, 0.19617864641932375, 0.19632504056288633, 0.1963508963931171, 0.1962287244464372, 0.1962632876851254, 0.19624545350953293, 0.1961583674588591, 0.19615767864435874, 0.1960939418396171, 0.1961887528452899, 0.196191051137297, 0.19616057569509984, 0.19612571516173982, 0.19611726575224908], [0.19607444971142848, 0.1961898215105828, 0.19601794534881978, 0.19613269688183757, 0.1961115790071225, 0.19594797044225307, 0.19606060049942015, 0.19601649143183641, 0.19597117968108654, 0.19600638876654736, 0.19585852459355163, 0.19592987158748879, 0.19582747279527885, 0.19592104553233206, 0.1958682831669354, 0.19598332086854944, 0.19615225169112027, 0.1967838774701925, 0.19819486448997733, 0.20084172564989655, 0.20453998780643579, 0.20845655370367416, 0.21198728344842965, 0.2148873882480672, 0.21615934537757908, 0.21489274347491555, 0.21205462191790653, 0.20882030237821453, 0.20620280500936147, 0.20418167938482548, 0.20294472899264968, 0.2023932441616409, 0.20202318003705688, 0.20201125031642958, 0.20212929635222562, 0.20263187041710903, 0.2031365436421962, 0.20339549696421189, 0.20364806824036902, 0.20315412085529067, 0.2023225584137086, 0.20099695730986364, 0.1998064393751248, 0.19868537217754464, 0.1977823602121865, 0.1972001535939039, 0.1968637446241193, 0.1967000123370537, 0.1965303498833245, 0.19649829414028422, 0.1966050071366194, 0.19652201489364274, 0.19649120310187226, 0.19638046234338352, 0.1964448213978583, 0.1963468458790002, 0.19649997533935482, 0.19635072020703226, 0.19626907400642954, 0.19631798360830105, 0.19630977628555205, 0.19625576297777886, 0.19626365651755992, 0.19623638068297547, 0.19616082095080906, 0.19615395730801646]]
  in  "Projections":i32=27 min=1 max=1000 step=2
  out "Readouts per shift cycle":i32=132
  in  "Start continuous imaging":bool
  in  "Readouts per projection (pk-pk)":i32=66 min=2 max=10000 step=2
  in  "Shift stop":dbl=-1.8
  in  "Shift start":dbl=1.8
  out "Shift frequency":dbl=2.705627705627706
  out "Current readout":i32=5379
  in  "Number of pulses per image":i32=7013
  in  "Rotation orientation":bool=TRUE
  out "Time per Image":dbl=4.9896
  out "Motor pulse time (T/2)":dbl=0.0003557393412234422 format="%#_6p"
  in  "Max images":i32=3
  out "Images completed":i32=3
  in  "Save enable\n(before start)":bool=TRUE
  in  "name identifier":string="P_normal_test"
  in  "Path":path=path "D:/MPIdata"
  in  "Online recon":bool=TRUE
  out "Max ROs":dbl=5379.0
  in  "patch amp":dbl=0.5 format="%_3p"
  in  "patch phase":dbl=290.0 format="%.2p"
  out "patch freq":dbl=-1.0 format="%#_5p"
  # "Safety switches"
  # "Global variables"
  # "Receive parameters"
  # "Shift field control"
  # "Rotation control"
  # "Shift field control"
  # "Rotation control"
  # "Shift field control"
  # "Rotation control"
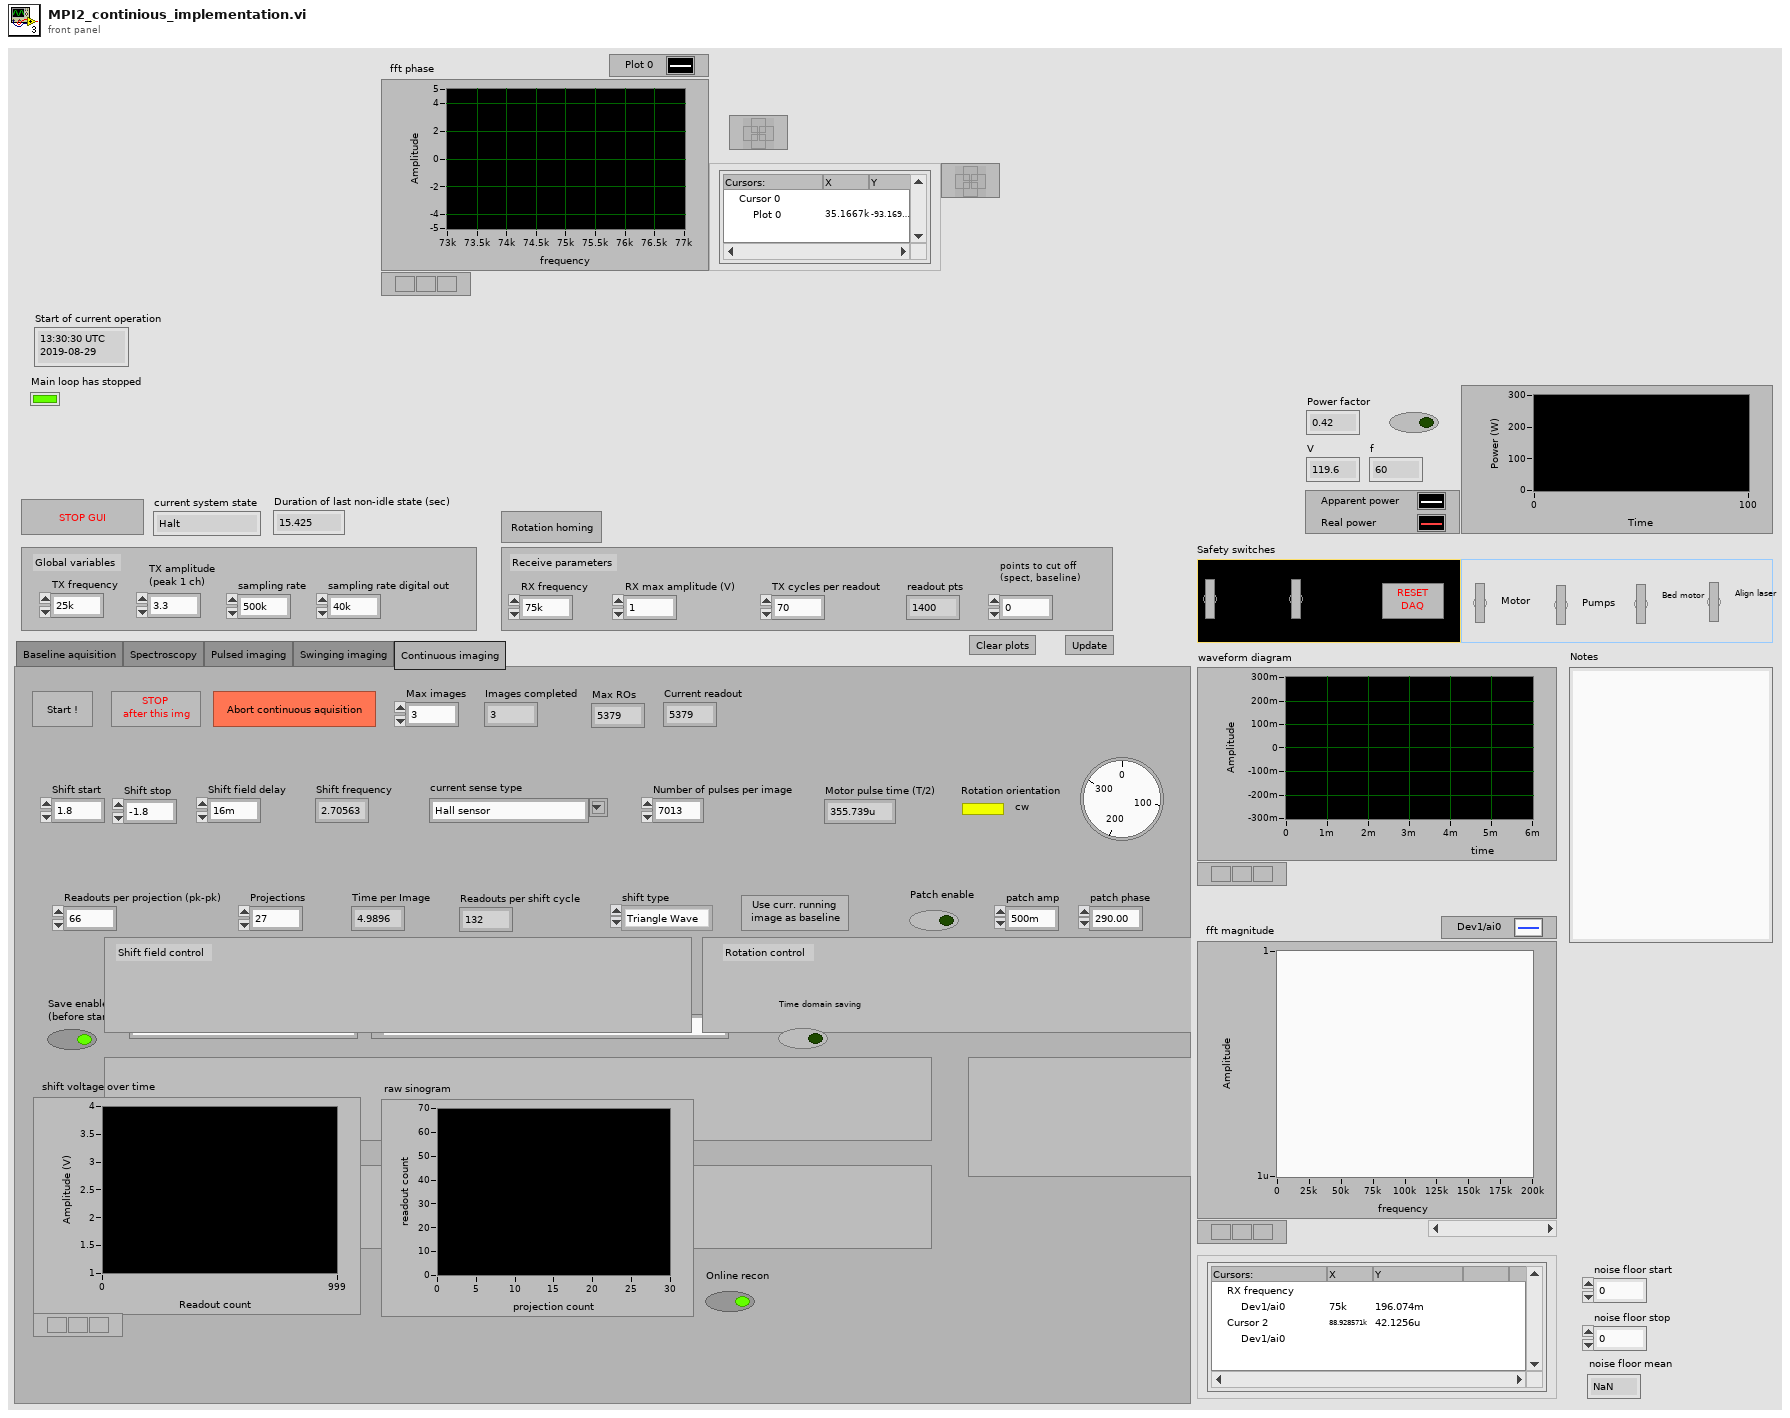
[diagram p1: front panel]
types:
  T1 = cluster{"apparant power (watt)":i32, "active power (watt)":i32}
  T2 = enum32{"Baseline aquisition", "Spectroscopy", "Pulsed imaging", "Swinging imaging", "Continuous imaging"}
  T3 = cluster{"Magnitude":dbl[], "Phase":dbl[], "Timing":dbl[], "Baseline magnitude":dbl, "Baseline phase":dbl, "Notes":string, "Cut-off points":i32, "Update delay (ms)":dbl, "Timestamp":timestamp, "Timing mode":string}
  T4 = cluster{"Magnitude meas.":dbl[], "Phase meas.":dbl[], "Shift meas.":dbl[], "cw":bool, "projections per image":i32, "ramp-up readouts":i32, "current sense type":string, "Number of pulses per image":i32, "Rotation enabled":bool, "Rotary position":dbl[], "Baseline magnitude":dbl, "Baseline phase":dbl, "Wait readouts":i32, "Shift waveform type":string, "Shift enabled":bool, "Time domain data":dbl[], "Motor pulse duration":dbl, "Shift start":dbl, "Shift stop":dbl, "Notes":string, "Reconstructed image":picture, "Rotary encoder type":string, "Image start":timestamp, "Image stop":timestamp, "readouts per projection":i32, "Recon enabled":bool, "Bidirectional shift":bool, "Imager mode":string, "Shift delay":dbl, "Shift frequency":dbl, "Image time (calc)":dbl, "Initial encoder position":dbl, "Recon data":dbl[][], "Trigger line values":i32[], "Bed position":dbl, "Sample image":picture, "Patch amplitude":dbl, "Patch frequency":dbl, "Patch phase":dbl}
  T5 = enum16{"open", "open or create", "create or replace", "create", "open (read-only)"}
  T6 = typedef "Tag-dbl.lvlib/))Channel.ctl" = refnum<queue>
  T7 = cluster{"relative position shaft":dbl, "relative position wheel":dbl}
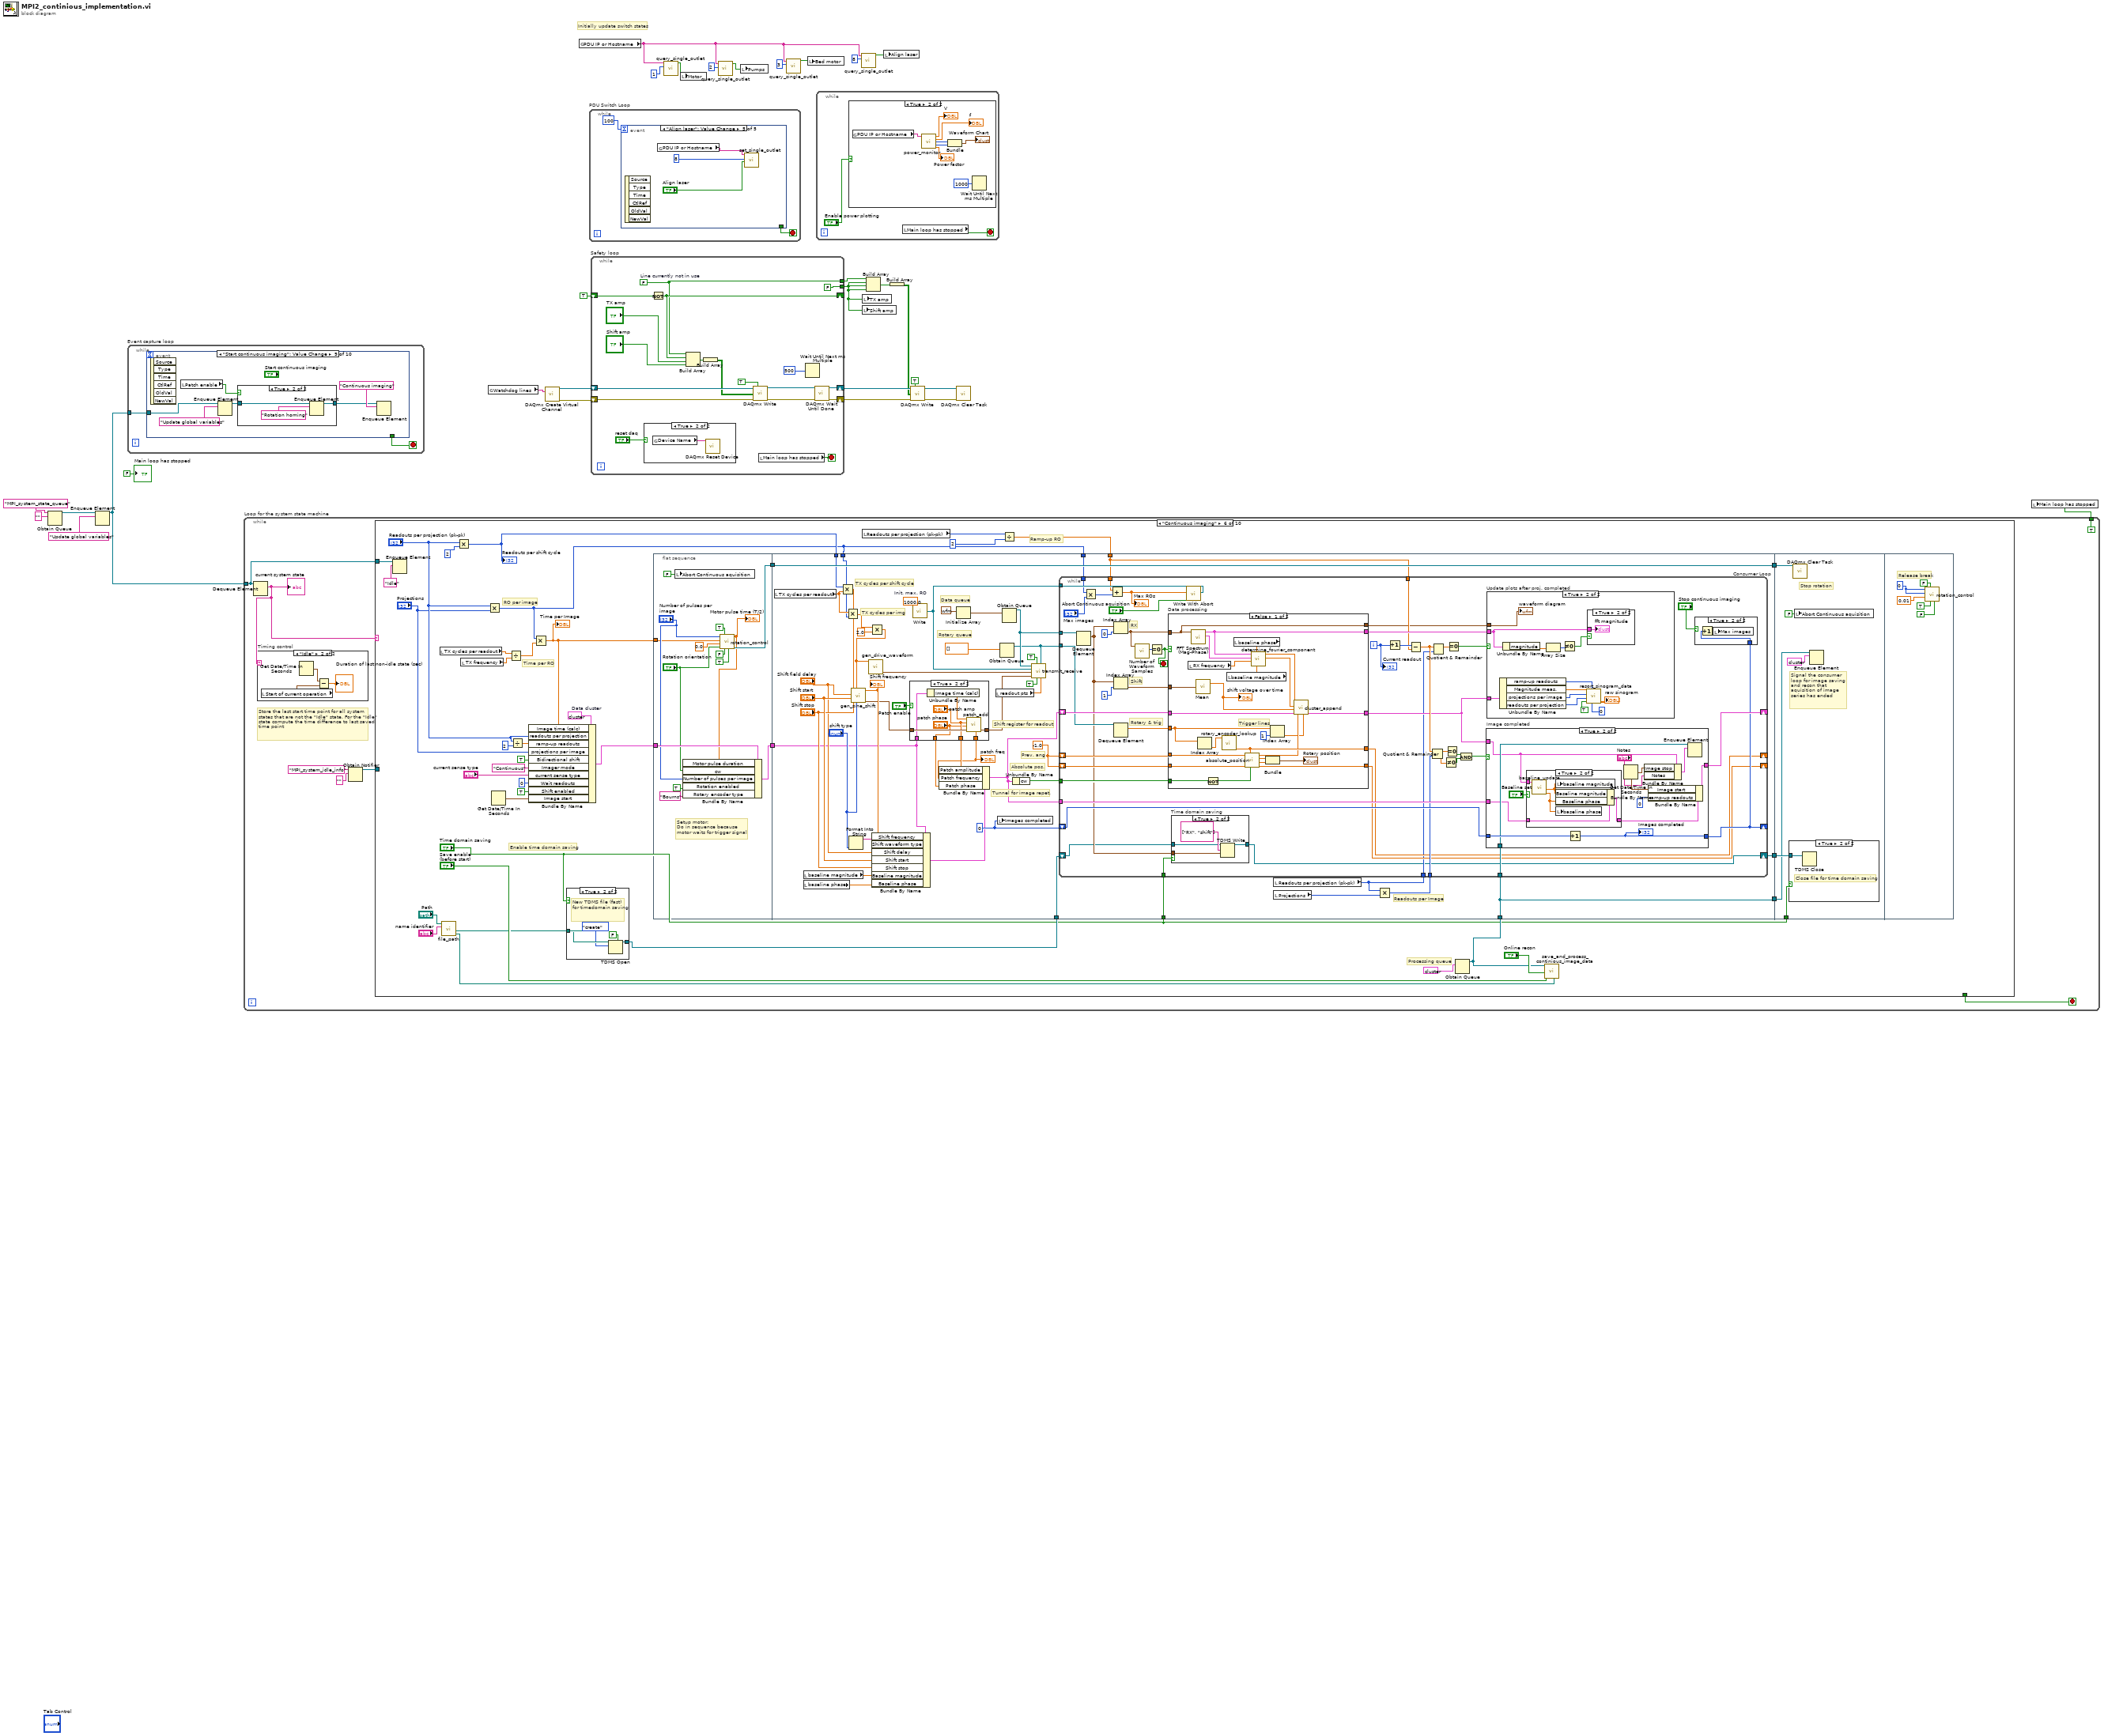
[diagram p0: block diagram]
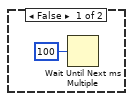
[diagram p2: hidden frame]
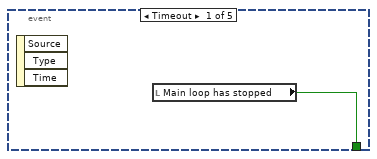
[diagram p3: hidden frame]
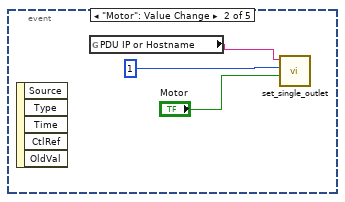
[diagram p4: hidden frame]
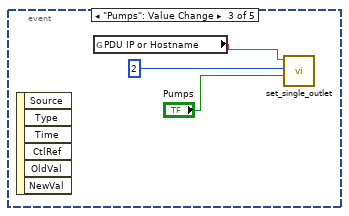
[diagram p5: hidden frame]
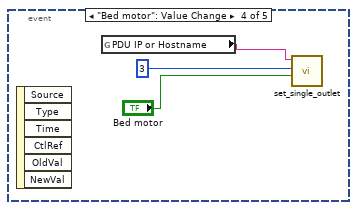
[diagram p6: hidden frame]
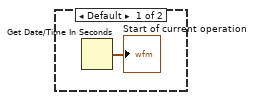
[diagram p8: hidden frame]
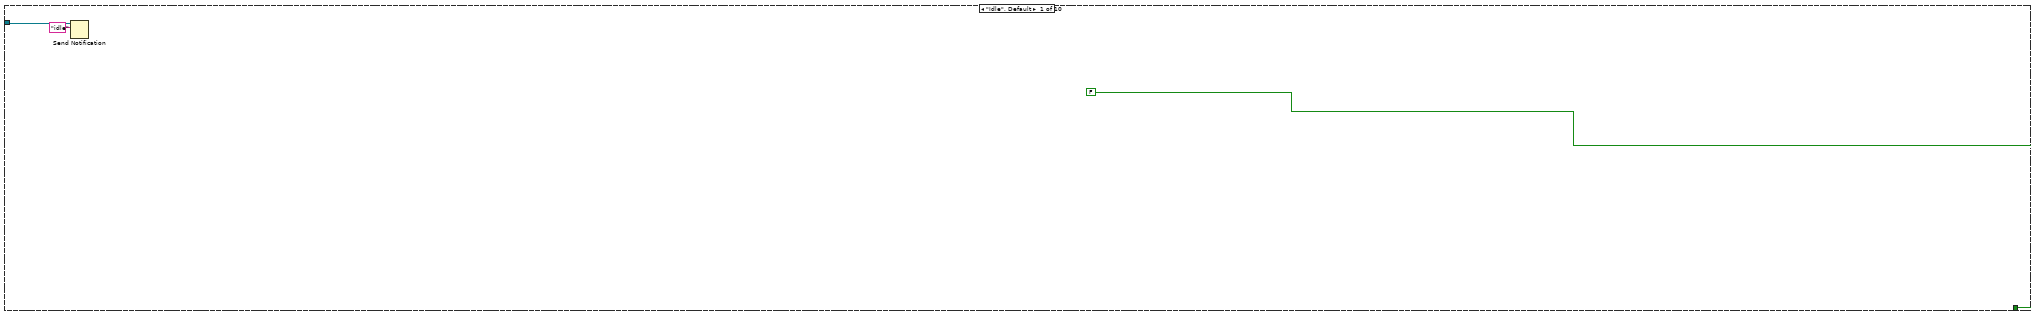
[diagram p9: hidden frame]
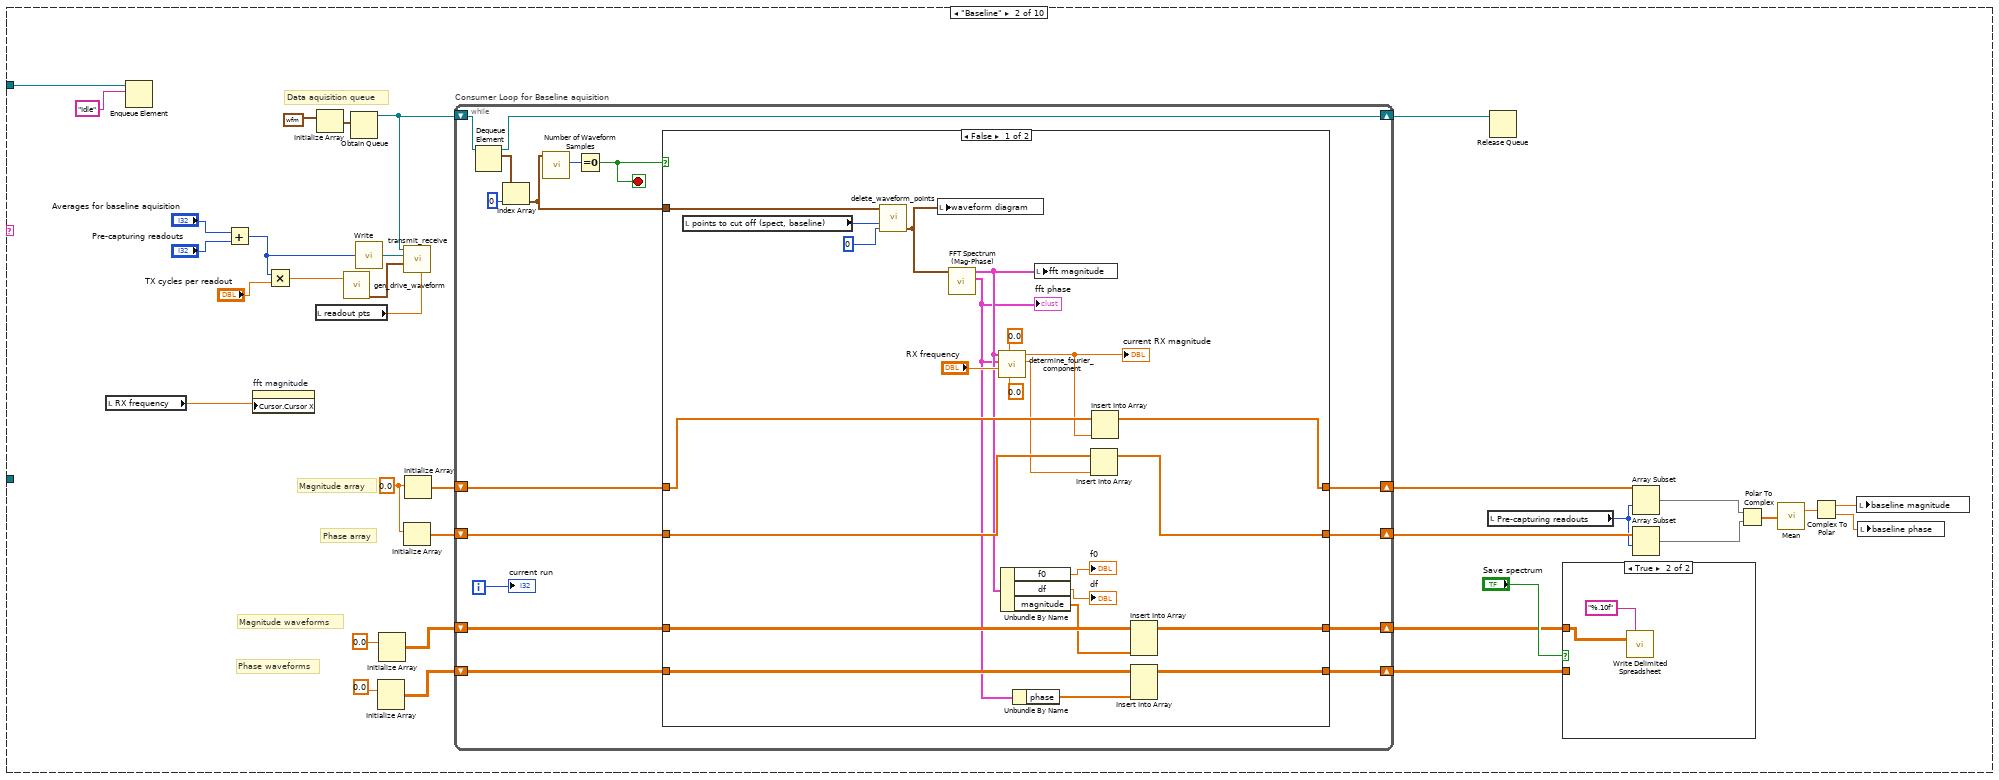
[diagram p10: hidden frame]
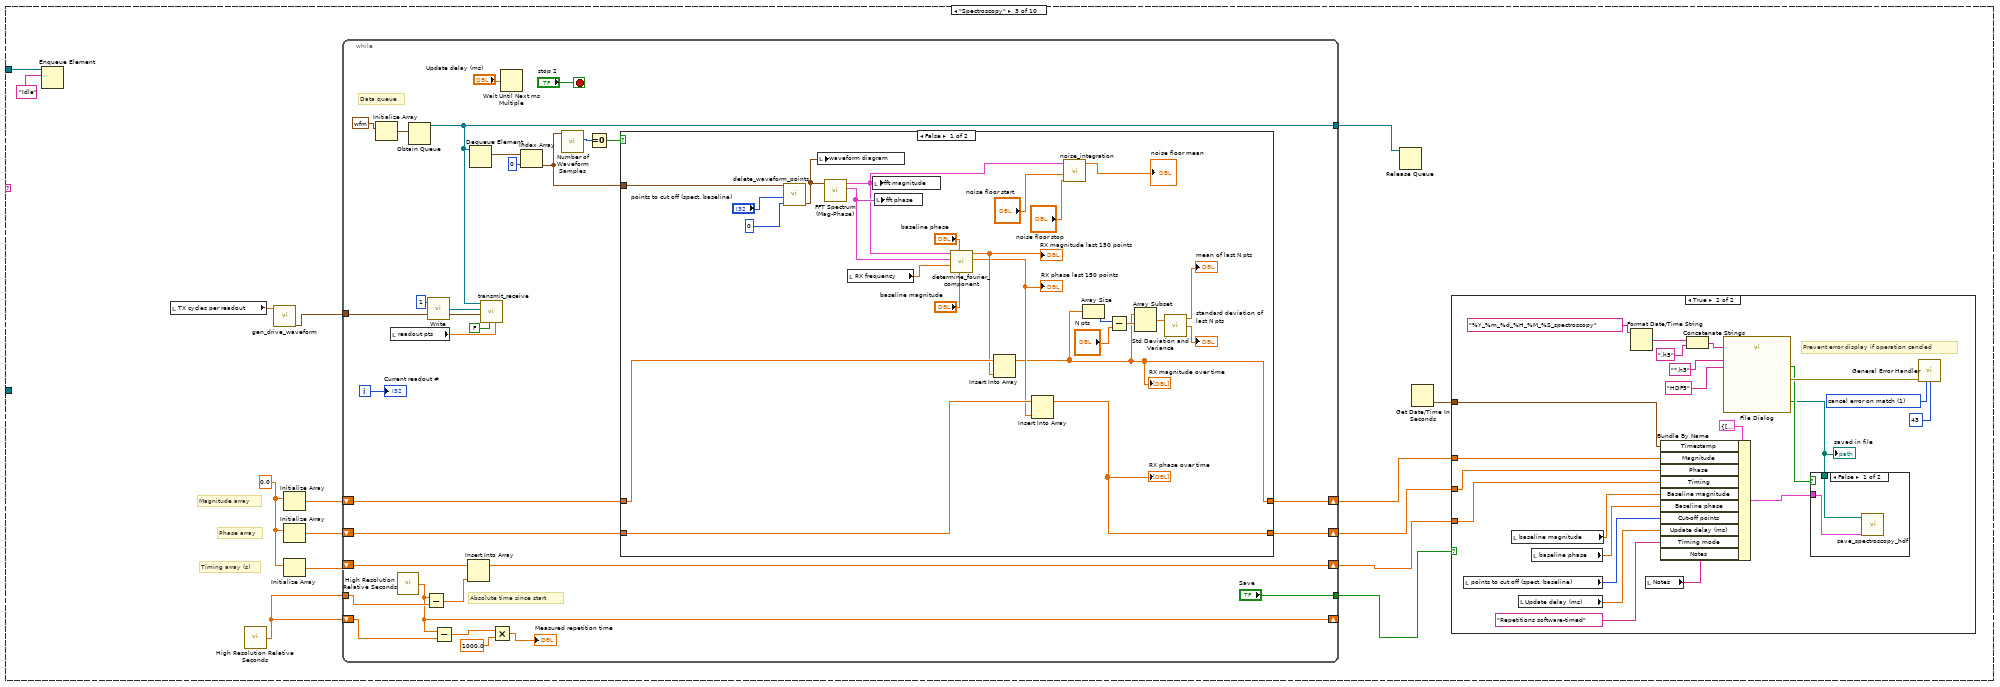
[diagram p13: hidden frame]
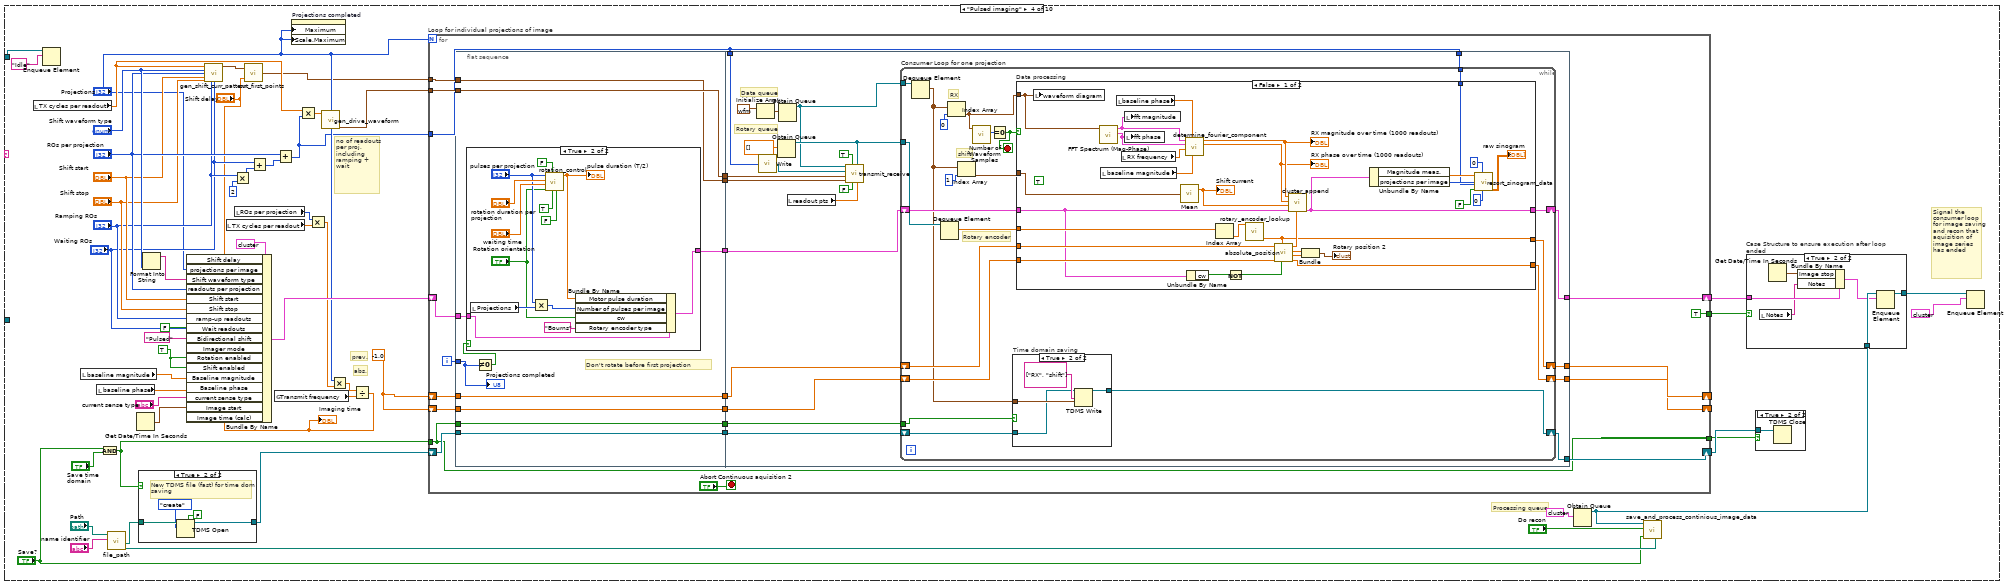
[diagram p17: hidden frame]
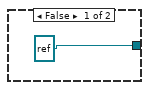
[diagram p20: hidden frame]
diagram:
  # "Initially update switch states"
  n1 = Obtain Queue(name (unnamed)="MPI_system_state_queue", element data type="" ("Type def")) -> (queue out=w25:refnum<queue>)  [unwired: 3 in, 2 out]
  n2 = Enqueue Element(queue=w25, element="Update global variables") -> (queue out=w27:refnum<queue>)  [unwired: 2 in, 2 out]
  n3 = while "Event capture loop" {
    tunnel: w27 -> [w30]
    stop <- w31 stop-if-true
    n4 = event shown="[8] \"Start continuous imaging\": Value Change" {
      selector: _ -> [_ _ _ _ _ _ _ _ _ _]
      dyn-events: _ -> [_ _ _ _ _ _ _ _ _ _]
      timeout: _ -> [_ _ _ _ _ _ _ _ _ _]
      tunnel: [FALSE TRUE _ _ _ _ _ _ _ _] -> w31
      tunnel: w30 -> [_ w34 w38 w40 w43 w46 w50 w55 w59 w66]
      event Timeout {
        n5 = event-data() -> ()  [unwired: 1 in, 3 out]
      }
      event "stop": Value Change {
        n6 = event-data() -> ()  [unwired: 1 in, 6 out]
        n7 = Enqueue Element(queue=w34, element="Halt") -> ()  [unwired: 2 in, 3 out]
      }
      event "Baseline state": Value Change {
        n8 = event-data() -> ()  [unwired: 1 in, 6 out]
        n9 = Enqueue Element(queue=w38, element="Update global variables") -> (queue out=w37:refnum<queue>)  [unwired: 2 in, 2 out]
        n10 = Enqueue Element(queue=w37, element="Baseline") -> ()  [unwired: 2 in, 3 out]
      }
      event "Clear plots": Value Change {
        n11 = event-data() -> ()  [unwired: 1 in, 6 out]
        n12 = Enqueue Element(queue=w40, element="Clear plots") -> ()  [unwired: 2 in, 3 out]
      }
      event "Update global variables Button": Value Change {
        n13 = event-data() -> ()  [unwired: 1 in, 6 out]
        n14 = Enqueue Element(queue=w43, element="Update global variables") -> ()  [unwired: 2 in, 3 out]
      }
      event "Start spectroscopy": Value Change {
        n15 = event-data() -> ()  [unwired: 1 in, 6 out]
        n16 = Enqueue Element(queue=w46, element="Update global variables") -> (queue out=w45:refnum<queue>)  [unwired: 2 in, 2 out]
        n17 = Enqueue Element(queue=w45, element="Spectroscopy") -> ()  [unwired: 2 in, 3 out]
      }
      event "Start imaging": Value Change {
        n18 = event-data() -> ()  [unwired: 1 in, 6 out]
        n19 = Enqueue Element(queue=w50, element="Update global variables") -> (queue out=w48:refnum<queue>)  [unwired: 2 in, 2 out]
        n20 = Enqueue Element(queue=w48, element="Pulsed imaging") -> ()  [unwired: 2 in, 3 out]
      }
      event "Start swinging imaging": Value Change {
        n21 = event-data() -> ()  [unwired: 1 in, 6 out]
        n22 = Enqueue Element(queue=w55, element="Update global variables") -> (queue out=w52:refnum<queue>)  [unwired: 2 in, 2 out]
        n23 = Enqueue Element(queue=w52, element="Swinging imaging") -> ()  [unwired: 2 in, 3 out]
      }
      event "Start continuous imaging": Value Change {
        n24 = event-data() -> ()  [unwired: 1 in, 6 out]
        n25 = local read "Patch enable"() -> (w58:bool)
        n26 = Enqueue Element(queue=w59, element="Update global variables") -> (queue out=w56:refnum<queue>)  [unwired: 2 in, 2 out]
        n27 = case shown="True" w58 {
          tunnel: [w62 w64] -> w57
          tunnel: w56 -> [w62 w65]
          frame False {
          }
          frame True {
            n28 = Enqueue Element(queue=w65, element="Rotation homing") -> (queue out=w64:refnum<queue>)  [unwired: 2 in, 2 out]
          }
        }
        n29 = Enqueue Element(queue=w57, element="Continuous imaging") -> ()  [unwired: 2 in, 3 out]
      }
      event "Rotation homing": Value Change {
        n30 = event-data() -> ()  [unwired: 1 in, 6 out]
        n31 = Enqueue Element(queue=w66, element="Rotation homing") -> ()  [unwired: 2 in, 3 out]
      }
    }
  }
  n32 = while "Loop for the system state machine" {
    tunnel: w27 -> [w73]
    tunnel: [TRUE] -> w23
    stop <- w74 stop-if-true
    # "Store the last start time point for all system states that are not the \"Idle\" state. For the \"Idle\" state compute the time difference to last saved time point"
    n33 = Dequeue Element(queue=w73) -> (element=w72:string)  [unwired: 2 in, 3 out]
    "current system state" <- w72
    n34 = case "Timing control" shown="\"Idle\"" w72 {
      frame Default {
        n35 = Get Date/Time In Seconds() -> (seconds since 1Jan1904=→"Start of current operation":timestamp)
      }
      frame "Idle" {
        n36 = local read "Start of current operation"() -> (w76:timestamp)
        n37 = Get Date/Time In Seconds() -> (seconds since 1Jan1904=w77:timestamp)
        n38 = Subtract(x=w77, y=w76) -> (x-y=→"Duration of last non-idle state (sec)":dbl)
      }
    }
    n39 = Obtain Notifier(name (unnamed)="MPI_system_idle_info", notification data type="") -> (notifier out=w69:refnum<notifier>)  [unwired: 2 in, 2 out]
    n40 = case shown="\"Continuous imaging\"" w72 {
      tunnel: [FALSE _ _ _ _ _ _ TRUE _ _] -> w74
      tunnel: w73 -> [_ w115 w174 w309 w462 w711 _ _ w928 w960]
      tunnel: w69 -> [w80 _ _ _ _ _ _ _ _ _]
      frame "Idle", Default {
        n41 = Send Notification(notification="idle", notifier=w80) -> ()  [unwired: 1 in, 2 out]
      }
      frame "Baseline" {
        w90 = 0.0 ("element")
        # "Phase waveforms"
        # "Magnitude waveforms"
        # "Data aquisition queue"
        # "Magnitude array"
        # "Phase array"
        n42 = local read "RX frequency"() -> (w89:dbl)
        n43 = Enqueue Element(queue=w115, element="Idle") -> ()  [unwired: 2 in, 3 out]
        n44 = Add(x="Averages for baseline aquisition", y="Pre-capturing readouts") -> (x+y=w92:i32)
        n45 = property on="fft magnitude" class="WFGraph (strict)"("Cursor.Cursor X"=w89) -> ()  [unwired: 2 in, 2 out]
        n46 = Multiply(x=w92, y="TX cycles per readout") -> (x*y=w103:dbl)
        n47 = local read "readout pts"() -> (w101:dbl)
        n48 = Initialize Array(waveform(dbl) {"t0"=timestamp(0 s since 1904-01-01), "dt"=1.0, "Y"=[]} ("Waveform")) -> (w93:waveform(dbl)[])  [unwired: 1 in]
        n49 = call "gen_drive_waveform.vi"("no of cycles"=w103) -> ("signal out"=w102:waveform(dbl))  [unwired: 10 in]
        n50 = Obtain Queue(element data type=w93) -> (queue out=w113:refnum<queue>)  [unwired: 4 in, 2 out]
        n51 = call <extravilib>:"Write.vi"("element"=w92) -> ("channel"=w91:T6)  [unwired: 1 out]
        n52 = Initialize Array(0.0 ("element")) -> (w87:dbl[][])  [unwired: 2 in]
        n53 = Initialize Array(0.0 ("element")) -> (w88:dbl[][])  [unwired: 2 in]
        n54 = call "transmit_receive.vi"("samples per readout"=w101, "Waveform drive"=w102, "channel input for max readouts"=w91, "measurement queue"=w113) -> ()  [unwired: 8 in]
        n55 = Initialize Array(w90) -> (w110:dbl[])  [unwired: 1 in]
        n56 = Initialize Array(w90) -> (w111:dbl[])  [unwired: 1 in]
        n57 = while "Consumer Loop for Baseline aquisition" {
          shift-right: [w131] -> w112
          shift-left: w113 -> [w133]
          shift-right: [w128] -> w106
          shift-left: w111 -> [w130]
          shift-right: [w127] -> w107
          shift-left: w110 -> [w129]
          shift-right: [w118] -> w85
          shift-left: w88 -> [w121]
          shift-right: [w119] -> w84
          shift-left: w87 -> [w120]
          i -> [w126]
          stop <- w122 stop-if-true
          n58 = Dequeue Element(queue=w133) -> (queue out=w131:refnum<queue>, element=w125:waveform(dbl)[])  [unwired: 2 in, 2 out]
          n59 = Index Array(array=w125, index=0) -> (element=w123:waveform(dbl))
          n60 = call-poly <vilib>:"Number of Waveform Samples.vi"("waveform in"=w123) -> ("number of samples"=w132:i32)  [unwired: 8 in, 2 out]
          n61 = Equal To 0?(x=w132) -> (x = 0?=w122:bool)
          n62 = case shown="False" w122 {
            tunnel: w123 -> [w145 _]
            tunnel: w130 -> [w156 w160]
            tunnel: w129 -> [w155 w159]
            tunnel: [w146 w160] -> w128
            tunnel: [w154 w159] -> w127
            tunnel: w121 -> [w143 w158]
            tunnel: w120 -> [w142 w157]
            tunnel: [w141 w157] -> w119
            tunnel: [w140 w158] -> w118
            frame False {
              n63 = local read "points to cut off (spect, baseline)"() -> (w148:i32)
              n64 = call "delete_waveform_points.vi"("index"=0, "length"=w148, "Original Waveform"=w145) -> ("New Waveform"=w144:waveform(dbl))  [unwired: 8 in]
              n65 = local write "waveform diagram"(w144) -> ()
              n66 = call-poly <vilib>:"FFT Spectrum (Mag-Phase).vi"("time signal"=w144) -> ("phase"=w136:cluster{"f0":dbl, "df":dbl, "phase":dbl[]}, "magnitude"=w139:cluster{"f0":dbl, "df":dbl, "magnitude":dbl[]})  [unwired: 6 in, 3 out]
              "fft phase" <- w136
              n67 = call "determine_fourier_component.vi"("baseline magnitude"=0.0, "baseline phase"=0.0, "RX frequency"="RX frequency", "phase"=w136, "magnitude"=w139) -> ("RX phase"=w149:dbl, "RX magnitude"=w150:dbl)  [unwired: 5 in]
              "current RX magnitude" <- w150
              n68 = Unbundle By Name(w139) -> ("f0"=→"f0":dbl, "df"=→"df":dbl, "magnitude"=w138:dbl[])
              n69 = Unbundle By Name(w136) -> ("phase"=w137:dbl[])
              n70 = local write "fft magnitude"(w139) -> ()
              n71 = Insert Into Array(array=w155, new element=w149) -> (w154:dbl[])  [unwired: 1 in]
              n72 = Insert Into Array(array=w156, new element=w150) -> (w146:dbl[])  [unwired: 1 in]
              n73 = Insert Into Array(array=w143, new element=w138) -> (w140:dbl[][])  [unwired: 2 in]
              n74 = Insert Into Array(array=w142, new element=w137) -> (w141:dbl[][])  [unwired: 2 in]
            }
            frame True {
            }
          }
          "current run" <- w126
        }
        n75 = local read "Pre-capturing readouts"() -> (w105:i32)
        n76 = Release Queue(queue=w112) -> ()  [unwired: 2 in, 3 out]
        n77 = case shown="True" "Save spectrum" {
          tunnel: w85 -> [_ w117]
          tunnel: w84 -> [_ _]
          frame False {
          }
          frame True {
            n78 = call-poly <vilib>:"Write Delimited Spreadsheet.vi"("format (%.3f)"="%.10f", "2D data"=w117) -> ()  [unwired: 12 in, 2 out]
          }
        }
        n79 = Array Subset(array=w106, index=w105) -> (w100:dbl[])  [unwired: 1 in]
        n80 = Array Subset(array=w107, index=w105) -> (w99:dbl[])  [unwired: 1 in]
        n81 = Polar To Complex(1:w99, 2:w100) -> (0:w98:cdb[])
        n82 = call-poly <vilib>:"Mean.vi"("X"=w98) -> ("mean"=w97:cdb)  [unwired: 1 out]
        n83 = Complex To Polar(r * e^(i*theta)=w97) -> (r=w96:dbl, theta=w95:dbl)
        n84 = local write "baseline magnitude"(w96) -> ()
        n85 = local write "baseline phase"(w95) -> ()
      }
      frame "Spectroscopy" {
        w167 = 0.0
        # "Timing array (s)"
        # "Phase array"
        # "Magnitude array"
        n86 = Enqueue Element(queue=w174, element="Idle") -> ()  [unwired: 2 in, 3 out]
        n87 = local read "TX cycles per readout"() -> (w171:dbl)
        n88 = call <vilib>:"High Resolution Relative Seconds.vi"() -> ("relative seconds"=w165:dbl)
        n89 = call "gen_drive_waveform.vi"("no of cycles"=w171) -> ("signal out"=w170:waveform(dbl))  [unwired: 10 in]
        n90 = Initialize Array(w167) -> (w173:dbl[])  [unwired: 1 in]
        n91 = Initialize Array(w167) -> (w172:dbl[])  [unwired: 1 in]
        n92 = Initialize Array(w167) -> (w166:dbl[])  [unwired: 1 in]
        n93 = while {
          tunnel: w170 -> [w230]
          shift-right: [w224] -> w169
          shift-left: w173 -> [w228]
          shift-right: [w221] -> w168
          shift-left: w172 -> [w222]
          shift-right: [w209] -> w162
          shift-left: w166 -> [w211]
          tunnel: w165 -> [w212]
          shift-right: [w207] -> _
          shift-left: w165 -> [w208]
          tunnel: [w206] -> w164
          tunnel: ["Save"] -> w163
          i -> [w201]
          stop <- "stop 2" stop-if-true
          # "Absolute time since start"
          # "Data queue"
          n94 = Initialize Array(waveform(dbl) {"t0"=timestamp(0 s since 1904-01-01), "dt"=1.0, "Y"=[]} ("Waveform")) -> (w219:waveform(dbl)[])  [unwired: 1 in]
          n95 = local read "readout pts"() -> (w229:dbl)
          n96 = call <vilib>:"High Resolution Relative Seconds.vi"() -> ("relative seconds"=w207:dbl)
          n97 = Obtain Queue(element data type=w219) -> (queue out=w206:refnum<queue>)  [unwired: 4 in, 2 out]
          n98 = Subtract(x=w207, y=w212) -> (x-y=w210:dbl)
          n99 = call <extravilib>:"Write.vi"("element"=1 ("number of readouts")) -> ("channel"=w213:T6)  [unwired: 1 out]
          n100 = Subtract(x=w207, y=w208) -> (x-y=w205:dbl)
          n101 = Insert Into Array(array=w211, new element=w210) -> (w209:dbl[])  [unwired: 1 in]
          n102 = Dequeue Element(queue=w206) -> (element=w217:waveform(dbl)[])  [unwired: 2 in, 3 out]
          n103 = call "transmit_receive.vi"("samples per readout"=w229, "Continious mode"=FALSE, "Waveform drive"=w230, "channel input for max readouts"=w213, "measurement queue"=w206) -> ()  [unwired: 7 in]
          n104 = Multiply(x=w205, y=1000.0) -> (x*y=→"Measured repetition time":dbl)
          n105 = Wait Until Next ms Multiple(millisecond multiple="Update delay (ms)") -> ()  [unwired: 1 out]
          n106 = Index Array(array=w217, index=0) -> (element=w218:waveform(dbl))
          n107 = call-poly <vilib>:"Number of Waveform Samples.vi"("waveform in"=w218) -> ("number of samples"=w226:i32)  [unwired: 8 in, 2 out]
          n108 = Equal To 0?(x=w226) -> (x = 0?=w225:bool)
          n109 = case shown="False" w225 {
            tunnel: w218 -> [w246 _]
            tunnel: w228 -> [w250 w256]
            tunnel: [w238 w256] -> w224
            tunnel: w222 -> [w248 w255]
            tunnel: [w247 w255] -> w221
            frame False {
              n110 = call "delete_waveform_points.vi"("index"=0, "length"="points to cut off (spect, baseline)", "Original Waveform"=w246) -> ("New Waveform"=w236:waveform(dbl))  [unwired: 8 in]
              n111 = local write "waveform diagram"(w236) -> ()
              n112 = call-poly <vilib>:"FFT Spectrum (Mag-Phase).vi"("time signal"=w236) -> ("phase"=w254:cluster{"f0":dbl, "df":dbl, "phase":dbl[]}, "magnitude"=w234:cluster{"f0":dbl, "df":dbl, "magnitude":dbl[]})  [unwired: 6 in, 3 out]
              n113 = local read "RX frequency"() -> (w253:dbl)
              n114 = local write "fft magnitude"(w234) -> ()
              n115 = local write "fft phase"(w254) -> ()
              n116 = call "determine_fourier_component.vi"("baseline magnitude"="baseline magnitude", "baseline phase"="baseline phase", "RX frequency"=w253, "phase"=w254, "magnitude"=w234) -> ("RX phase"=w243:dbl, "RX magnitude"=w249:dbl)  [unwired: 5 in]
              "RX magnitude last 150 points" <- w249
              "RX phase last 150 points" <- w243
              n117 = Insert Into Array(array=w250, new element=w249) -> (w238:dbl[])  [unwired: 1 in]
              "RX magnitude over time" <- w238
              n118 = Insert Into Array(array=w248, new element=w243) -> (w247:dbl[])  [unwired: 1 in]
              "RX phase over time" <- w247
              n119 = call "noise_integration.vi"("stop frequency"="noise floor stop", "start frequency"="noise floor start", "magnitude"=w234) -> ("mean"=→"noise floor mean":dbl)  [unwired: 8 in]
              n120 = Array Size(array=w238) -> (size(s)=w242:i32)
              n121 = Subtract(x=w242, y="N pts") -> (x-y=w241:dbl)
              n122 = Array Subset(array=w238, index=w241) -> (w240:dbl[])  [unwired: 1 in]
              n123 = call <vilib>:"Std Deviation and Variance.vi"("X"=w240) -> ("mean"=→"mean of last N pts":dbl, "standard deviation"=→"standard deviation of last N pts":dbl)  [unwired: 1 in, 1 out]
            }
            frame True {
            }
          }
          "Current readout #" <- w201
        }
        n124 = Release Queue(queue=w164) -> ()  [unwired: 2 in, 3 out]
        n125 = Get Date/Time In Seconds() -> (seconds since 1Jan1904=w161:timestamp)
        n126 = case shown="True" w163 {
          tunnel: w169 -> [_ w186]
          tunnel: w168 -> [_ w185]
          tunnel: w162 -> [_ w184]
          tunnel: w161 -> [_ w180]
          frame False {
          }
          frame True {
            w191 = 1 items=["no exception", "cancel error on match", "set error on match"] ("[exception action] (none:0)")
            # "Prevent error display if operation cancled"
            n127 = local read "points to cut off (spect, baseline)"() -> (w181:i32)
            n128 = local read "baseline magnitude"() -> (w183:dbl)
            n129 = local read "Update delay (ms)"() -> (w179:dbl)
            n130 = local read "baseline phase"() -> (w182:dbl)
            n131 = Format Date/Time String(time format string (%c)="%Y_%m_%d_%H_%M_%S_spectroscopy") -> (date/time string=w198:string)  [unwired: 2 in]
            n132 = local read "Notes"() -> (w176:string)
            n133 = Bundle By Name(cluster=T3 {"Magnitude"=[], "Phase"=[], "Timing"=[], "Baseline magnitude"=0.0, "Baseline phase"=0.0, "Notes"="", "Cut-off points"=0, "Update delay (ms)"=0.0, "Timestamp"=timestamp(0 s since 1904-01-01), "Timing mode"=""}, "Timestamp"=w180, "Magnitude"=w186, "Phase"=w185, "Timing"=w184, "Baseline magnitude"=w183, "Baseline phase"=w182, "Cut-off points"=w181, "Update delay (ms)"=w179, "Timing mode"="Repetitions software-timed", "Notes"=w176) -> (w177:T3)
            n134 = Concatenate Strings(w198, ".h5" ("string")) -> (w196:string)
            n135 = call "File Dialog"("default name"=w196, "pattern (all files)"="*.h5" ("pattern label"), "pattern label"="HDF5") -> ("selected path"=w188:path, "cancelled"=w189:bool, "error out"=w192:errorcluster)  [unwired: 9 in, 1 out]
            "saved in file" <- w188
            n136 = case shown="False" w189 {
              tunnel: w188 -> [w200 _]
              tunnel: w177 -> [w199 _]
              frame False {
                n137 = call "save_spectroscopy_hdf.vi"("Spectroscopy cluster in"=w199, "file path"=w200) -> ()  [unwired: 10 in]
              }
              frame True {
              }
            }
            n138 = call <vilib>:"General Error Handler.vi"("error in (no error)"=w192, "[exception action] (none:0)"=w191, "[exception code]"=43) -> ()  [unwired: 8 in, 5 out]
          }
        }
      }
      frame "Pulsed imaging" {
        w274 = -1.0
        w278 = TRUE ("Rotation enabled")
        # "Signal the consumer loop for image saving and recon that aquisition of image series has ended"
        # "abs."
        # "prev."
        # "Processing queue"
        # "no of readouts per proj,\nincluding ramping + wait"
        n139 = local read "TX cycles per readout"() -> (w305:dbl)
        n140 = Enqueue Element(queue=w309, element="Idle") -> ()  [unwired: 2 in, 3 out]
        n141 = local read "baseline magnitude"() -> (w293:dbl)
        n142 = local read "baseline phase"() -> (w292:dbl)
        n143 = And(x="Save?", y="Save time\ndomain") -> (x .and. y?=w275:bool)
        n144 = call "file_path.vi"("name identifier"="name identifier", "Base path"="Path") -> ("HDF path"=w287:path, "TDMS path"=w290:path)  [unwired: 8 in]
        n145 = Get Date/Time In Seconds() -> (seconds since 1Jan1904=w276:timestamp)
        n146 = case shown="True" w275 {
          tunnel: w290 -> [_ w322]
          tunnel: [refnum<k34> refnum ("tdms file out") w319] -> w283
          frame False {
          }
          frame True {
            # "New TDMS file (fast) for time dom  saving"
            n147 = TDMS Open(5:FALSE ("create index file? (T)"), 10:T5."create" ("operation (0:open)"), 11:w322) -> (3:w319:refnum<k34>)  [unwired: 4 in, 1 out]
          }
        }
        n148 = Format Into String("Shift waveform type") -> (resulting string=w302:string)  [unwired: 3 in, 1 out]
        n149 = call "gen_shift_curr_pattern.vi"("Cycles per readout"=w305, "Waveform type"="Shift waveform type", "Readouts per projection"="ROs per projection", "Ramp start"="Shift start", "Ramp stop"="Shift stop", "Ramp-up readouts"="Ramping ROs", "Wait readouts"="Waiting ROs") -> ("output waveform"=w266:waveform(dbl))  [unwired: 7 in, 1 out]
        n150 = local read "TX cycles per readout"() -> (w261:dbl)
        n151 = Multiply(x="Ramping ROs", y=2) -> (x*y=w307:i32)
        n152 = local read "ROs per projection"() -> (w262:i32)
        n153 = call "cut_first_points.vi"("time offset"="Shift delay", "waveform in"=w266) -> ("output waveform"=w265:waveform(dbl))
        n154 = Add(x="Waiting ROs", y=w307) -> (x+y=w306:i32)
        n155 = global read "global_variables.vi" "Transmit frequency"() -> (w279:dbl)
        n156 = Add(x="ROs per projection", y=w306) -> (x+y=w263:i32)
        n157 = property on="Projections completed" class="Slide (strict)"("Maximum"="Projections", "Scale.Maximum"="Projections") -> ()  [unwired: 2 in, 2 out]
        n158 = Multiply(x=w305, y=w263) -> (x*y=w281:dbl)
        n159 = Multiply(x=w262, y=w261) -> (x*y=w260:dbl)
        n160 = call "gen_drive_waveform.vi"("no of cycles"=w281) -> ("signal out"=w304:waveform(dbl))  [unwired: 10 in]
        n161 = Multiply(x="Projections", y=w260) -> (x*y=w280:dbl)
        n162 = Divide(x=w280, y=w279) -> (x/y=w277:dbl)
        "Imaging time" <- w277
        n163 = Bundle By Name(cluster=T4 {"Magnitude meas."=[], "Phase meas."=[], "Shift meas."=[], "cw"=TRUE, "projections per image"=0, "ramp-up readouts"=0, "current sense type"="", "Number of pulses per image"=0, "Rotation enabled"=TRUE, "Rotary position"=[], "Baseline magnitude"=0.0, "Baseline phase"=0.0, "Wait readouts"=0, "Shift waveform type"="", "Shift enabled"=TRUE, "Time domain data"=[], "Motor pulse duration"=0.0, "Shift start"=0.0, "Shift stop"=0.0, "Notes"="", "Reconstructed image"=bytes[0], "Rotary encoder type"="", "Image start"=timestamp(0 s since 1904-01-01), "Image stop"=timestamp(0 s since 1904-01-01), "readouts per projection"=0, "Recon enabled"=FALSE, "Bidirectional shift"=FALSE, "Imager mode"="", "Shift delay"=0.0, "Shift frequency"=0.0, "Image time (calc)"=0.0, "Initial encoder position"=0.0, "Recon data"=[], "Trigger line values"=[], "Bed position"=0.0, "Sample image"=bytes[0], "Patch amplitude"=0.0, "Patch frequency"=0.0, "Patch phase"=0.0}, "Shift delay"="Shift delay", "projections per image"="Projections", "Shift waveform type"=w302, "readouts per projection"="ROs per projection", "Shift start"="Shift start", "Shift stop"="Shift stop", "ramp-up readouts"="Ramping ROs", "Wait readouts"="Waiting ROs", "Bidirectional shift"=FALSE, "Imager mode"="Pulsed", "Rotation enabled"=w278, "Shift enabled"=w278, "Baseline magnitude"=w293, "Baseline phase"=w292, "current sense type"="current sense type", "Image start"=w276, "Image time (calc)"=w277) -> (w282:T4)
        n164 = for "Loop for individual projections of image" {
          N: "Projections" -> [_]
          tunnel: w265 -> [w329]
          tunnel: w304 -> [w331]
          tunnel: w263 -> [w323]
          shift-right: [w344] -> w271
          shift-left: w282 -> [w333]
          shift-right: [w340] -> w273
          shift-left: w283 -> [w343]
          shift-right: [w342] -> _
          shift-left: w274 -> [w326]
          shift-right: [w341] -> _
          shift-left: w274 -> [w325]
          tunnel: w275 -> [w334]
          tunnel: [w334] -> w272
          tunnel: [TRUE] -> w269
          i -> [w327]
          stop <- "Abort Continuous aquisition 2" stop-if-true
          n165 = flat-sequence {
            tunnel: w334 -> [w353]
            tunnel: w343 -> [w354]
            tunnel: [w354] -> w338
            tunnel: [w346] -> w337
            tunnel: [w353] -> w336
            tunnel: w333 -> [w351]
            tunnel: [w350] -> w332
            tunnel: w331 -> [w349]
            tunnel: [w349] -> w330
            tunnel: w329 -> [w348]
            tunnel: [w348] -> w328
            tunnel: w327 -> [w347]
            tunnel: w326 -> [w346]
            tunnel: w325 -> [w345]
            tunnel: [w345] -> w324
            tunnel: [w386] -> w344
            tunnel: [w384] -> w342
            tunnel: [w383] -> w341
            tunnel: [w380] -> w340
            tunnel: w338 -> [w385]
            tunnel: w337 -> [w382]
            tunnel: w336 -> [w379]
            tunnel: w332 -> [w371]
            tunnel: w330 -> [w389]
            tunnel: w328 -> [w390]
            tunnel: w324 -> [w381]
            tunnel: w323 -> [w370]
            tunnel: w323 -> [w369]
            frame #0 {
              # "Don't rotate before first projection"
              n166 = Not Equal To 0?(x=w347) -> (x != 0?=w352:bool)
              n167 = case shown="True" w352 {
                tunnel: [w355 w358] -> w350
                tunnel: w351 -> [w355 w356]
                frame False {
                }
                frame True {
                  n168 = local read "Projections"() -> (w363:i32)
                  n169 = Multiply(x="pulses per projection", y=w363) -> (x*y=w364:i32)
                  n170 = call "rotation_control.vi"("Continuous output"=FALSE, "Wait for completion?"=TRUE, "Triggered start?"=FALSE, "Rotation orientation"="Rotation orientation", "waiting time"="waiting time", "Duration of rotation"="rotation duration per projection", "Number of pulses"="pulses per projection") -> ("pulse duration (T/2)"=w359:dbl)  [unwired: 3 in, 1 out]
                  "pulse duration (T/2)" <- w359
                  n171 = Bundle By Name(cluster=w356, "Motor pulse duration"=w359, "Number of pulses per image"=w364, "cw"="Rotation orientation", "Rotary encoder type"="Bourns") -> (w358:T4)
                }
              }
              "Projections completed" <- w347
            }
            frame #1 {
              # "Rotary queue"
              # "Data queue"
              n172 = Initialize Array(waveform(dbl) {"t0"=timestamp(0 s since 1904-01-01), "dt"=1.0, "Y"=[]} ("Waveform")) -> (w377:waveform(dbl)[])  [unwired: 1 in]
              n173 = call <extravilib>:"Write.vi"("element"=w370) -> ("channel"=w372:T6)  [unwired: 1 out]
              n174 = Obtain Queue(element data type=dbl[] []) -> (queue out=w388:refnum<queue>)  [unwired: 4 in, 2 out]
              n175 = Obtain Queue(element data type=w377) -> (queue out=w387:refnum<queue>)  [unwired: 4 in, 2 out]
              n176 = local read "readout pts"() -> (w373:dbl)
              n177 = call "transmit_receive.vi"("samples per readout"=w373, "rotary queue"=w388, "Continious mode"=FALSE, "Enable rotary encoder"=TRUE, "Waveform shift"=w390, "Waveform drive"=w389, "channel input for max readouts"=w372, "measurement queue"=w387) -> ()  [unwired: 4 in]
              n178 = while "Consumer Loop for one projection" {
                tunnel: w388 -> [w402]
                tunnel: w387 -> [w403]
                shift-right: [w400] -> w386
                shift-left: w371 -> [w405]
                shift-right: [w397] -> w384
                shift-left: w382 -> [w399]
                shift-right: [w396] -> w383
                shift-left: w381 -> [w398]
                tunnel: w379 -> [w393]
                shift-right: [w392] -> w380
                shift-left: w385 -> [w395]
                tunnel: w369 -> [w391]
                stop <- w404 stop-if-true
                # "Rotary encoder"
                # "shift"
                # "RX"
                n179 = Dequeue Element(queue=w403) -> (element=w394:waveform(dbl)[])  [unwired: 2 in, 3 out]
                n180 = Dequeue Element(queue=w402) -> (element=w401:dbl[])  [unwired: 2 in, 3 out]
                n181 = Index Array(array=w394, index=0) -> (element=w409:waveform(dbl))
                n182 = Index Array(array=w394, index=1) -> (element=w406:waveform(dbl))
                n183 = call-poly <vilib>:"Number of Waveform Samples.vi"("waveform in"=w409) -> ("number of samples"=w410:i32)  [unwired: 8 in, 2 out]
                n184 = Equal To 0?(x=w410) -> (x = 0?=w404:bool)
                n185 = case "Time domain saving" shown="True" w393 {
                  tunnel: w394 -> [_ w414]
                  tunnel: w395 -> [w411 w413]
                  tunnel: [w411 w412] -> w392
                  frame False {
                  }
                  frame True {
                    n186 = TDMS Write(0:w413, 7:string[] ["RX", "shift"] ("channel name(s) in (Untitled)"), 9:w414) -> (4:w412:refnum<k34>)  [unwired: 3 in, 3 out]
                  }
                }
                n187 = case "Data processing" shown="False" w404 {
                  tunnel: w409 -> [w446 _]
                  tunnel: w406 -> [w438 _]
                  tunnel: w405 -> [w427 w449]
                  tunnel: w401 -> [w432 _]
                  tunnel: [w419 w449] -> w400
                  tunnel: w399 -> [w431 w448]
                  tunnel: w398 -> [w430 w447]
                  tunnel: [w429 w448] -> w397
                  tunnel: [w426 w447] -> w396
                  tunnel: w391 -> [w416 _]
                  frame False {
                    (unwired) TRUE ("Read")
                    n188 = local write "waveform diagram"(w446) -> ()
                    n189 = call-poly <vilib>:"FFT Spectrum (Mag-Phase).vi"("time signal"=w446) -> ("phase"=w444:cluster{"f0":dbl, "df":dbl, "phase":dbl[]}, "magnitude"=w445:cluster{"f0":dbl, "df":dbl, "magnitude":dbl[]})  [unwired: 6 in, 3 out]
                    n190 = local read "baseline magnitude"() -> (w442:dbl)
                    n191 = local read "baseline phase"() -> (w443:dbl)
                    n192 = local read "RX frequency"() -> (w441:dbl)
                    n193 = local write "fft magnitude"(w445) -> ()
                    n194 = local write "fft phase"(w444) -> ()
                    n195 = call-poly <vilib>:"Mean.vi"("X"=w438) -> ("mean"=w424:dbl)  [unwired: 1 out]
                    "Shift current" <- w424
                    n196 = call "determine_fourier_component.vi"("baseline magnitude"=w442, "baseline phase"=w443, "RX frequency"=w441, "phase"=w444, "magnitude"=w445) -> ("RX phase"=w439:dbl, "RX magnitude"=w440:dbl)  [unwired: 5 in]
                    "RX magnitude over time (1000 readouts)" <- w440
                    "RX phase over time (1000 readouts)" <- w439
                    n197 = Unbundle By Name(w427) -> ("cw"=w428:bool)
                    n198 = Index Array(array=w432) -> (element=w437:dbl)  [unwired: 1 in]
                    n199 = Not(x=w428) -> (.not. x?=w434:bool)
                    n200 = call "rotary_encoder_lookup.vi"("Code from Encoder"=w437) -> ("angle (deg)"=w429:dbl)  [unwired: 10 in]
                    n201 = call "absolute_position.vi"("Encoder rotates cw"=w434, "curr. angle"=w429, "Absolute position in"=w430, "prev. angle"=w431) -> ("Absolute position out"=w426:dbl, "relative position wheel"=w435:dbl, "relative position shaft"=w436:dbl, "Wheel Position (abs)"=w433:dbl)  [unwired: 4 in]
                    n202 = call "cluster_append.vi"("Rotary encoder"=w433, "Input Cluster"=w427, "shift value"=w424, "phase value"=w439, "magnitude value"=w440) -> ("Output Cluster"=w419:T4)  [unwired: 6 in]
                    n203 = Bundle("relative position shaft"=w436, "relative position wheel"=w435) -> (→"Rotary position 2":T7)  [unwired: 1 in]
                    n204 = Unbundle By Name(w419) -> ("Magnitude meas."=w423:dbl[], "projections per image"=w422:i32)
                    n205 = call "resort_sinogram_data.vi"("Ramp end"=0, "Ramp begin"=0, "Shift up and down"=FALSE, "pts per projection"=w416, "projections"=w422, "Input"=w423) -> ("Output"=→"raw sinogram":dbl[][])  [unwired: 5 in]
                  }
                  frame True {
                    # "In case that data aqusition finished, a waveform of length=0 is added to the queue. In this case we don't want to do the data processing (FFT, 3rd harmonic)."
                  }
                }
              }
            }
          }
        }
        n206 = Obtain Queue(element data type=T4 {"Magnitude meas."=[], "Phase meas."=[], "Shift meas."=[], "cw"=TRUE, "projections per image"=0, "ramp-up readouts"=0, "current sense type"="", "Number of pulses per image"=0, "Rotation enabled"=TRUE, "Rotary position"=[], "Baseline magnitude"=0.0, "Baseline phase"=0.0, "Wait readouts"=0, "Shift waveform type"="", "Shift enabled"=TRUE, "Time domain data"=[], "Motor pulse duration"=0.0, "Shift start"=0.0, "Shift stop"=0.0, "Notes"="", "Reconstructed image"=bytes[0], "Rotary encoder type"="", "Image start"=timestamp(0 s since 1904-01-01), "Image stop"=timestamp(0 s since 1904-01-01), "readouts per projection"=0, "Recon enabled"=FALSE, "Bidirectional shift"=FALSE, "Imager mode"="", "Shift delay"=0.0, "Shift frequency"=0.0, "Image time (calc)"=0.0, "Initial encoder position"=0.0, "Recon data"=[], "Trigger line values"=[], "Bed position"=0.0, "Sample image"=bytes[0], "Patch amplitude"=0.0, "Patch frequency"=0.0, "Patch phase"=0.0}) -> (queue out=w270:refnum<queue>)  [unwired: 4 in, 2 out]
        n207 = call "save_and_process_continious_image_data.vi"("Path"=w287, "Save"="Save?", "Enable online recon"="Do recon", "queue in"=w270) -> ()  [unwired: 8 in]
        n208 = case "Case Structure to ensure execution after loop ended" shown="True" w269 {
          tunnel: w271 -> [_ w315]
          tunnel: w270 -> [w310 w316]
          tunnel: [w310 w312] -> w268
          frame False {
          }
          frame True {
            n209 = local read "Notes"() -> (w311:string)
            n210 = Get Date/Time In Seconds() -> (seconds since 1Jan1904=w314:timestamp)
            n211 = Bundle By Name(cluster=w315, "Image stop"=w314, "Notes"=w311) -> (w313:T4)
            n212 = Enqueue Element(queue=w316, element=w313) -> (queue out=w312:refnum<queue>)  [unwired: 2 in, 2 out]
          }
        }
        n213 = case shown="True" w272 {
          tunnel: w273 -> [_ w317]
          frame False {
          }
          frame True {
            n214 = TDMS Close(11:w317) -> ()  [unwired: 1 in, 2 out]
          }
        }
        n215 = Enqueue Element(queue=w268, element=T4 {"Magnitude meas."=[], "Phase meas."=[], "Shift meas."=[], "cw"=TRUE, "projections per image"=0, "ramp-up readouts"=0, "current sense type"="", "Number of pulses per image"=0, "Rotation enabled"=TRUE, "Rotary position"=[], "Baseline magnitude"=0.0, "Baseline phase"=0.0, "Wait readouts"=0, "Shift waveform type"="", "Shift enabled"=TRUE, "Time domain data"=[], "Motor pulse duration"=0.0, "Shift start"=0.0, "Shift stop"=0.0, "Notes"="", "Reconstructed image"=bytes[0], "Rotary encoder type"="", "Image start"=timestamp(0 s since 1904-01-01), "Image stop"=timestamp(0 s since 1904-01-01), "readouts per projection"=0, "Recon enabled"=FALSE, "Bidirectional shift"=FALSE, "Imager mode"="", "Shift delay"=0.0, "Shift frequency"=0.0, "Image time (calc)"=0.0, "Initial encoder position"=0.0, "Recon data"=[], "Trigger line values"=[], "Bed position"=0.0, "Sample image"=bytes[0], "Patch amplitude"=0.0, "Patch frequency"=0.0, "Patch phase"=0.0}) -> ()  [unwired: 2 in, 3 out]
      }
      frame "Swinging imaging" {
        # "Processing queue"
        n216 = Enqueue Element(queue=w462, element="Idle") -> ()  [unwired: 2 in, 3 out]
        n217 = call "file_path.vi"("name identifier"="name identifier", "Base path"="Path") -> ("HDF path"=w452:path, "TDMS path"=w455:path)  [unwired: 8 in]
        n218 = flat-sequence "Sequence to notify saving and reconstruction cumser that image aquisition is done" {
          tunnel: [w463] -> w460
          tunnel: [w468] -> w459
          tunnel: [w467] -> w458
          tunnel: w455 -> [w466]
          tunnel: ["Save enable\n(before start)"] -> w451
          tunnel: w453 -> [w463]
          tunnel: w460 -> [w672]
          tunnel: w459 -> [w671]
          tunnel: w458 -> [w670]
          frame #0 {
            w465 = -1.0
            # "Absolute pos."
            # "Prev. ang"
            n219 = call <vilib>:"High Resolution Relative Seconds.vi"() -> ("relative seconds"=w473:dbl)
            n220 = local write "Images completed"(0 ("Images completed")) -> ()
            n221 = And(x="Time domain saving", y="Save enable\n(before start)") -> (x .and. y?=w469:bool)
            n222 = case shown="True" w469 {
              tunnel: w466 -> [_ w478]
              tunnel: [refnum<k34> refnum ("tdms file out") w475] -> w470
              frame False {
              }
              frame True {
                # "New TDMS file (fast) for time dom  saving"
                n223 = TDMS Open(5:FALSE ("create index file? (T)"), 10:T5."create" ("operation (0:open)"), 11:w478) -> (3:w475:refnum<k34>)  [unwired: 4 in, 1 out]
              }
            }
            n224 = while "image repetition loop" {
              shift-right: [w518] -> _
              shift-left: w473 -> [w522]
              tunnel: w463 -> [w498]
              tunnel: w469 -> [w492]
              shift-right: [w493] -> w467
              shift-left: w470 -> [w497]
              tunnel: [w492] -> w468
              shift-right: [w484] -> _
              shift-left: w465 -> [w488]
              shift-right: [w485] -> _
              shift-left: w465 -> [w491]
              i -> [w524]
              stop <- w523 stop-if-true
              # "image repetition timing"
              n225 = local read "TX cycles per readout"() -> (w531:dbl)
              n226 = local read "baseline magnitude"() -> (w501:dbl)
              n227 = call <vilib>:"High Resolution Relative Seconds.vi"() -> ("relative seconds"=w518:dbl)
              n228 = local read "baseline phase"() -> (w500:dbl)
              n229 = case shown="True" "Enable shift" {
                tunnel: [enum16{"None", "Stair", "Ramp", "Sine"}."None" ("Waveform type") "shift waveform"] -> w507
                frame False {
                }
                frame True {
                }
              }
              n230 = Subtract(x=w518, y=w522) -> (x-y=w520:dbl)
              n231 = Divide(x=w520, y=u32 1000) -> (x/y=→"image repetition time (sec)":dbl)
              n232 = call "gen_shift_curr_pattern.vi"("Cycles per readout"=w531, "Waveform type"=w507, "Readouts per projection"="Readouts per projection", "Ramp start"="Shift start", "Ramp stop"="Shift stop", "Ramp-up readouts"="Ramp ROs", "Wait readouts"="Wait ROs") -> ("output waveform"=w528:waveform(dbl))  [unwired: 7 in, 1 out]
              n233 = Format Into String(w507) -> (resulting string=w505:string)  [unwired: 3 in, 1 out]
              n234 = Bundle By Name(cluster=T4 {"Magnitude meas."=[], "Phase meas."=[], "Shift meas."=[], "cw"=TRUE, "projections per image"=0, "ramp-up readouts"=0, "current sense type"="", "Number of pulses per image"=0, "Rotation enabled"=TRUE, "Rotary position"=[], "Baseline magnitude"=0.0, "Baseline phase"=0.0, "Wait readouts"=0, "Shift waveform type"="", "Shift enabled"=TRUE, "Time domain data"=[], "Motor pulse duration"=0.0, "Shift start"=0.0, "Shift stop"=0.0, "Notes"="", "Reconstructed image"=bytes[0], "Rotary encoder type"="", "Image start"=timestamp(0 s since 1904-01-01), "Image stop"=timestamp(0 s since 1904-01-01), "readouts per projection"=0, "Recon enabled"=FALSE, "Bidirectional shift"=FALSE, "Imager mode"="", "Shift delay"=0.0, "Shift frequency"=0.0, "Image time (calc)"=0.0, "Initial encoder position"=0.0, "Recon data"=[], "Trigger line values"=[], "Bed position"=0.0, "Sample image"=bytes[0], "Patch amplitude"=0.0, "Patch frequency"=0.0, "Patch phase"=0.0}, "Shift delay"="shift delay", "projections per image"="projections per image", "Shift waveform type"=w505, "readouts per projection"="Readouts per projection", "Shift start"="Shift start", "Shift stop"="Shift stop", "ramp-up readouts"="Ramp ROs", "Wait readouts"="Wait ROs", "Shift enabled"="Enable shift", "current sense type"="current sense type", "Imager mode"="Swinging", "Bidirectional shift"=FALSE, "Baseline magnitude"=w501, "Baseline phase"=w500) -> (w525:T4)
              n235 = local read "readout pts"() -> (w530:dbl)
              n236 = local read "TX cycles per readout"() -> (w517:dbl)
              n237 = call "repeat_waveform.vi"("waveform repetitions"="projections per image", "signal in"=w528) -> ("waveform length"=w532:i32, "signal out"=w482:waveform(dbl))  [unwired: 8 in]
              n238 = Divide(x=w532, y=w530) -> (x/y=w516:dbl)
              "Readouts per image" <- w516
              n239 = call "cut_first_points.vi"("time offset"="shift delay", "waveform in"=w482) -> ("output waveform"=w481:waveform(dbl))
              n240 = Multiply(x=w516, y=w517) -> (x*y=w529:dbl)
              n241 = call "gen_drive_waveform.vi"("no of cycles"=w529) -> ("signal out"=w527:waveform(dbl))  [unwired: 10 in]
              n242 = flat-sequence "Sequence for 1 image: 1. Set up rotation, 2. run image, 3. storage & rotation control" {
                tunnel: w532 -> [w554]
                tunnel: w525 -> [w548]
                tunnel: [w549] -> w503
                tunnel: [w547] -> w499
                tunnel: w497 -> [w542]
                tunnel: [w542] -> w496
                tunnel: w492 -> [w541]
                tunnel: [w541] -> w495
                tunnel: w491 -> [w540]
                tunnel: [w540] -> w490
                tunnel: w488 -> [w539]
                tunnel: [w539] -> w489
                tunnel: ["Rotation orientation"] -> w487
                tunnel: w481 -> [w583]
                tunnel: w527 -> [w582]
                tunnel: [w579] -> w526
                tunnel: [w573] -> w504
                tunnel: w503 -> [w573]
                tunnel: w499 -> [w578]
                tunnel: w496 -> [w572]
                tunnel: w495 -> [w571]
                tunnel: [w570] -> w494
                tunnel: w490 -> [w566]
                tunnel: w489 -> [w565]
                tunnel: w487 -> [w564]
                tunnel: [w563] -> w486
                tunnel: [w562] -> w483
                tunnel: [w657] -> w523
                tunnel: w526 -> [w654]
                tunnel: w524 -> [w660]
                tunnel: w504 -> [w645]
                tunnel: w498 -> [w652]
                tunnel: [w651] -> w493
                tunnel: w494 -> [w651]
                tunnel: [w648] -> w485
                tunnel: w486 -> [w648]
                tunnel: [w647] -> w484
                tunnel: w483 -> [w647]
                frame #0 {
                  # "Rotation control"
                  n243 = global read "global_variables.vi" "sample rate"() -> (w555:dbl)
                  n244 = Not(x="Disable rotation") -> (.not. x?=w545:bool)
                  "Rotation on" <- w545
                  n245 = Divide(x=w554, y=w555) -> (x/y=w543:dbl)
                  "imaging time (sec, calc)" <- w543
                  n246 = case shown="False" "Disable rotation" {
                    tunnel: [w558 w560] -> w550
                    tunnel: w543 -> [w558 w560]
                    tunnel: [0.0 ("y") w560] -> w553
                    tunnel: "Number of pulses" -> [w557 _]
                    tunnel: [w557 0 ("Number of pulses")] -> w536
                    frame False {
                      # "Rotation enabled"
                    }
                    frame True {
                    }
                  }
                  n247 = call "rotation_control.vi"("Continuous output"=FALSE, "Wait for completion?"=FALSE, "Triggered start?"=TRUE, "Rotation orientation"="Rotation orientation", "waiting time"=w553, "Duration of rotation"=w550, "Number of pulses"=w536) -> ("task out"=w549:refnum<k21>, "pulse duration (T/2)"=w546:dbl)  [unwired: 3 in]
                  "motor pulse duration (T/2)" <- w546
                  n248 = Bundle By Name(cluster=w548, "Motor pulse duration"=w546, "Number of pulses per image"=w536, "cw"="Rotation orientation", "Rotation enabled"=w545, "Rotary encoder type"="Bourns", "Image time (calc)"=w543) -> (w547:T4)
                }
                frame #1 {
                  # "Rotary queue"
                  # "Data queue"
                  n249 = Get Date/Time In Seconds() -> (seconds since 1Jan1904=w576:timestamp)
                  n250 = local read "Readouts per image"() -> (w575:dbl)
                  n251 = Bundle By Name(cluster=w578, "Image start"=w576) -> (w577:T4)
                  n252 = Initialize Array(waveform(dbl) {"t0"=timestamp(0 s since 1904-01-01), "dt"=1.0, "Y"=[]} ("Waveform")) -> (w580:waveform(dbl)[])  [unwired: 1 in]
                  n253 = local read "readout pts"() -> (w585:dbl)
                  n254 = Obtain Queue(element data type=dbl[] []) -> (queue out=w567:refnum<queue>)  [unwired: 4 in, 2 out]
                  n255 = Obtain Queue(element data type=w580) -> (queue out=w584:refnum<queue>)  [unwired: 4 in, 2 out]
                  n256 = call <extravilib>:"Write.vi"("element"=w575) -> ("channel"=w574:T6)  [unwired: 1 out]
                  n257 = call "transmit_receive.vi"("samples per readout"=w585, "rotary queue"=w567, "Enable rotary encoder"=TRUE, "Waveform shift"=w583, "Waveform drive"=w582, "channel input for max readouts"=w574, "measurement queue"=w584) -> ()  [unwired: 5 in]
                  n258 = while "Consumer Loop" {
                    tunnel: w584 -> [w605]
                    shift-right: [w598] -> w579
                    shift-left: w577 -> [w599]
                    shift-right: [w593] -> w570
                    shift-left: w572 -> [w596]
                    tunnel: w571 -> [w594]
                    tunnel: w567 -> [w592]
                    shift-right: [w588] -> w563
                    shift-left: w566 -> [w590]
                    shift-right: [w587] -> w562
                    shift-left: w565 -> [w589]
                    tunnel: w564 -> [w586]
                    stop <- w597 stop-if-true
                    # "RX"
                    # "Shift"
                    # "Rotary"
                    n259 = Dequeue Element(queue=w605) -> (element=w595:waveform(dbl)[])  [unwired: 2 in, 3 out]
                    n260 = Dequeue Element(queue=w592) -> (element=w591:dbl[])  [unwired: 2 in, 3 out]
                    n261 = Index Array(array=w595, index=1) -> (element=w601:waveform(dbl))
                    n262 = Index Array(array=w595, index=0) -> (element=w602:waveform(dbl))
                    n263 = call-poly <vilib>:"Number of Waveform Samples.vi"("waveform in"=w602) -> ("number of samples"=w604:i32)  [unwired: 8 in, 2 out]
                    n264 = Equal To 0?(x=w604) -> (x = 0?=w597:bool)
                    n265 = case "Time domain saving" shown="True" w594 {
                      tunnel: w595 -> [_ w609]
                      tunnel: w596 -> [w606 w608]
                      tunnel: [w606 w607] -> w593
                      frame False {
                      }
                      frame True {
                        n266 = TDMS Write(0:w608, 7:string[] ["RX", "shift"] ("channel name(s) in (Untitled)"), 9:w609) -> (4:w607:refnum<k34>)  [unwired: 3 in, 3 out]
                      }
                    }
                    n267 = case shown="False" w597 {
                      tunnel: w602 -> [w632 _]
                      tunnel: w601 -> [w631 _]
                      tunnel: w599 -> [w636 w644]
                      tunnel: [w634 w644] -> w598
                      tunnel: w591 -> [w617 _]
                      tunnel: w590 -> [w615 w643]
                      tunnel: w589 -> [w614 w642]
                      tunnel: [w613 w643] -> w588
                      tunnel: [w612 w642] -> w587
                      tunnel: w586 -> [w611 _]
                      frame False {
                        n268 = call-poly <vilib>:"FFT Spectrum (Mag-Phase).vi"("time signal"=w632) -> ("phase"=w640:cluster{"f0":dbl, "df":dbl, "phase":dbl[]}, "magnitude"=w641:cluster{"f0":dbl, "df":dbl, "magnitude":dbl[]})  [unwired: 6 in, 3 out]
                        n269 = local write "waveform diagram"(w632) -> ()
                        n270 = call-poly <vilib>:"Mean.vi"("X"=w631) -> ("mean"=w630:dbl)  [unwired: 1 out]
                        "shift voltage over time" <- w630
                        n271 = Index Array(array=w617) -> (element=w622:dbl)  [unwired: 1 in]
                        n272 = Not(x=w611) -> (.not. x?=w618:bool)
                        n273 = call "rotary_encoder_lookup.vi"("Code from Encoder"=w622) -> ("angle (deg)"=w613:dbl)  [unwired: 10 in]
                        n274 = local read "baseline magnitude"() -> (w638:dbl)
                        n275 = local read "baseline phase"() -> (w639:dbl)
                        n276 = local write "fft magnitude"(w641) -> ()
                        n277 = local write "fft phase"(w640) -> ()
                        n278 = local read "RX frequency"() -> (w637:dbl)
                        n279 = call "absolute_position.vi"("Encoder rotates cw"=w618, "curr. angle"=w613, "Absolute position in"=w614, "prev. angle"=w615) -> ("Absolute position out"=w612:dbl, "relative position wheel"=w619:dbl, "relative position shaft"=w620:dbl, "Wheel Position (abs)"=w616:dbl)  [unwired: 4 in]
                        n280 = Bundle("relative position shaft"=w620, "relative position wheel"=w619) -> (→"Rotary position":T7)  [unwired: 1 in]
                        n281 = call "determine_fourier_component.vi"("baseline magnitude"=w638, "baseline phase"=w639, "RX frequency"=w637, "phase"=w640, "magnitude"=w641) -> ("RX phase"=w635:dbl, "RX magnitude"=w633:dbl)  [unwired: 5 in]
                        "RX magnitude over time (1000 readouts)" <- w633
                        "RX phase over time (1000 readouts)" <- w635
                        n282 = call "cluster_append.vi"("Rotary encoder"=w616, "Input Cluster"=w636, "shift value"=w630, "phase value"=w635, "magnitude value"=w633) -> ("Output Cluster"=w634:T4)  [unwired: 6 in]
                        n283 = Unbundle By Name(w634) -> ("Magnitude meas."=w629:dbl[], "projections per image"=w627:i32, "readouts per projection"=w623:i32)
                        n284 = call "resort_sinogram_data.vi"("Ramp end"=0, "Ramp begin"=0, "Shift up and down"=FALSE, "pts per projection"=w623, "projections"=w627, "Input"=w629) -> ("Output"=→"raw sinogram":dbl[][])  [unwired: 5 in]
                      }
                      frame True {
                      }
                    }
                  }
                }
                frame #2 {
                  # "Release motor handles"
                  n285 = local read "Notes"() -> (w646:string)
                  n286 = Get Date/Time In Seconds() -> (seconds since 1Jan1904=w653:timestamp)
                  n287 = Bundle By Name(cluster=w654, "Image stop"=w653, "Notes"=w646) -> (w650:T4)
                  n288 = call <vilib>:"DAQmx Clear Task.vi"("task in"=w645) -> ()  [unwired: 14 in, 1 out]
                  n289 = local read "Rotation on"() -> (w661:bool)
                  n290 = case "Baseline update" shown="True" "Continious baseline set" {
                    tunnel: w650 -> [_ w666]
                    frame False {
                    }
                    frame True {
                      n291 = local read "baseline magnitude"() -> (w664:dbl)
                      n292 = local read "baseline phase"() -> (w665:dbl)
                      n293 = call "baseline_update.vi"("current baseline phase"=w665, "current baseline magnitude"=w664, "Cluster in"=w666) -> ("new baseline phase"=w662:dbl, "new baseline magnitude"=w663:dbl)  [unwired: 7 in]
                      n294 = local write "baseline magnitude"(w663) -> ()
                      n295 = local write "baseline phase"(w662) -> ()
                    }
                  }
                  n296 = Enqueue Element(queue=w652, element=w650) -> ()  [unwired: 2 in, 3 out]
                  n297 = case "Switch Rotation orientation" shown="True" w661 {
                    frame False {
                    }
                    frame True {
                      n298 = local read "Rotation orientation"() -> (w668:bool)
                      n299 = Not(x=w668) -> (.not. x?=w667:bool)
                      n300 = local write "Rotation orientation"(w667) -> ()
                    }
                  }
                  n301 = Increment(x=w660) -> (x+1=w659:i32)
                  "Images completed" <- w659
                  n302 = Greater Or Equal?(x=w659, y="Max images") -> (x >= y?=w655:bool)
                  n303 = Or(x="stop 3", y=w655) -> (x .or. y?=w657:bool)
                }
              }
              "shift on" <- "Enable shift"
            }
          }
          frame #1 {
            # "Signal the consumer loop for image saving and recon that aquisition of image series has ended"
            n304 = case shown="True" w671 {
              tunnel: w670 -> [_ w673]
              frame False {
              }
              frame True {
                n305 = TDMS Close(11:w673) -> ()  [unwired: 1 in, 2 out]
              }
            }
            n306 = Enqueue Element(queue=w672, element=T4 {"Magnitude meas."=[], "Phase meas."=[], "Shift meas."=[], "cw"=TRUE, "projections per image"=0, "ramp-up readouts"=0, "current sense type"="", "Number of pulses per image"=0, "Rotation enabled"=TRUE, "Rotary position"=[], "Baseline magnitude"=0.0, "Baseline phase"=0.0, "Wait readouts"=0, "Shift waveform type"="", "Shift enabled"=TRUE, "Time domain data"=[], "Motor pulse duration"=0.0, "Shift start"=0.0, "Shift stop"=0.0, "Notes"="", "Reconstructed image"=bytes[0], "Rotary encoder type"="", "Image start"=timestamp(0 s since 1904-01-01), "Image stop"=timestamp(0 s since 1904-01-01), "readouts per projection"=0, "Recon enabled"=FALSE, "Bidirectional shift"=FALSE, "Imager mode"="", "Shift delay"=0.0, "Shift frequency"=0.0, "Image time (calc)"=0.0, "Initial encoder position"=0.0, "Recon data"=[], "Trigger line values"=[], "Bed position"=0.0, "Sample image"=bytes[0], "Patch amplitude"=0.0, "Patch frequency"=0.0, "Patch phase"=0.0}) -> ()  [unwired: 2 in, 3 out]
          }
        }
        n307 = Obtain Queue(element data type=T4 {"Magnitude meas."=[], "Phase meas."=[], "Shift meas."=[], "cw"=TRUE, "projections per image"=0, "ramp-up readouts"=0, "current sense type"="", "Number of pulses per image"=0, "Rotation enabled"=TRUE, "Rotary position"=[], "Baseline magnitude"=0.0, "Baseline phase"=0.0, "Wait readouts"=0, "Shift waveform type"="", "Shift enabled"=TRUE, "Time domain data"=[], "Motor pulse duration"=0.0, "Shift start"=0.0, "Shift stop"=0.0, "Notes"="", "Reconstructed image"=bytes[0], "Rotary encoder type"="", "Image start"=timestamp(0 s since 1904-01-01), "Image stop"=timestamp(0 s since 1904-01-01), "readouts per projection"=0, "Recon enabled"=FALSE, "Bidirectional shift"=FALSE, "Imager mode"="", "Shift delay"=0.0, "Shift frequency"=0.0, "Image time (calc)"=0.0, "Initial encoder position"=0.0, "Recon data"=[], "Trigger line values"=[], "Bed position"=0.0, "Sample image"=bytes[0], "Patch amplitude"=0.0, "Patch frequency"=0.0, "Patch phase"=0.0}) -> (queue out=w453:refnum<queue>)  [unwired: 4 in, 2 out]
        n308 = call "save_and_process_continious_image_data.vi"("Path"=w452, "Save"=w451, "Enable online recon"="Online recon", "queue in"=w453) -> ()  [unwired: 8 in]
      }
      frame "Continuous imaging" {
        w675 = T4 {"Magnitude meas."=[], "Phase meas."=[], "Shift meas."=[], "cw"=TRUE, "projections per image"=0, "ramp-up readouts"=0, "current sense type"="", "Number of pulses per image"=0, "Rotation enabled"=TRUE, "Rotary position"=[], "Baseline magnitude"=0.0, "Baseline phase"=0.0, "Wait readouts"=0, "Shift waveform type"="", "Shift enabled"=TRUE, "Time domain data"=[], "Motor pulse duration"=0.0, "Shift start"=0.0, "Shift stop"=0.0, "Notes"="", "Reconstructed image"=bytes[0], "Rotary encoder type"="", "Image start"=timestamp(0 s since 1904-01-01), "Image stop"=timestamp(0 s since 1904-01-01), "readouts per projection"=0, "Recon enabled"=FALSE, "Bidirectional shift"=FALSE, "Imager mode"="", "Shift delay"=0.0, "Shift frequency"=0.0, "Image time (calc)"=0.0, "Initial encoder position"=0.0, "Recon data"=[], "Trigger line values"=[], "Bed position"=0.0, "Sample image"=bytes[0], "Patch amplitude"=0.0, "Patch frequency"=0.0, "Patch phase"=0.0}  # Data cluster
        # "Enable time domain saving"
        # "Processing queue"
        # "Ramp-up RO"
        # "RO per image"
        # "Time per RO"
        n309 = Enqueue Element(queue=w711, element="Idle") -> ()  [unwired: 2 in, 3 out]
        n310 = local read "TX cycles per readout"() -> (w707:dbl)
        n311 = call "file_path.vi"("name identifier"="name identifier", "Base path"="Path") -> ("HDF path"=w681:path, "TDMS path"=w680:path)  [unwired: 8 in]
        n312 = Multiply(x="Readouts per projection (pk-pk)", y=2) -> (x*y=w702:i32)
        "Readouts per shift cycle" <- w702
        n313 = local read "TX frequency"() -> (w706:dbl)
        n314 = Multiply(x="Readouts per projection (pk-pk)", y="Projections") -> (x*y=w676:i32)
        n315 = Get Date/Time In Seconds() -> (seconds since 1Jan1904=w693:timestamp)
        n316 = Divide(x=w707, y=w706) -> (x/y=w705:dbl)
        n317 = Divide(x="Readouts per projection (pk-pk)", y=2) -> (x/y=w700:dbl)
        n318 = Multiply(x=w676, y=w705) -> (x*y=w701:dbl)
        "Time per Image" <- w701
        n319 = Bundle By Name(cluster=w675, "Image time (calc)"=w701, "readouts per projection"="Readouts per projection (pk-pk)", "ramp-up readouts"=w700, "projections per image"="Projections", "Bidirectional shift"=TRUE, "Imager mode"="Continuous", "current sense type"="current sense type", "Wait readouts"=0, "Shift enabled"=TRUE, "Image start"=w693) -> (w692:T4)
        n320 = case shown="True" "Time domain saving" {
          tunnel: w680 -> [_ w717]
          tunnel: [refnum<k34> refnum ("tdms file out") w714] -> w684
          frame False {
          }
          frame True {
            # "New TDMS file (fast) for timedomain saving"
            n321 = TDMS Open(5:FALSE ("create index file? (T)"), 10:T5."create" ("operation (0:open)"), 11:w717) -> (3:w714:refnum<k34>)  [unwired: 4 in, 1 out]
          }
        }
        n322 = flat-sequence {
          tunnel: [w727] -> w710
          tunnel: w701 -> [w720]
          tunnel: w692 -> [w725]
          tunnel: [w721] -> w691
          tunnel: w710 -> [w774]
          tunnel: [w774] -> w709
          tunnel: w702 -> [w773]
          tunnel: w703 -> [w746]
          tunnel: w691 -> [w742]
          tunnel: w676 -> [w760]
          tunnel: w688 -> [w757]
          tunnel: "Time domain saving" -> [w753]
          tunnel: w684 -> [w750]
          tunnel: [w749] -> w679
          tunnel: [w746] -> w678
          tunnel: w676 -> [w740]
          tunnel: w709 -> [w916]
          tunnel: w679 -> [w914]
          tunnel: "Time domain saving" -> [w913]
          tunnel: w678 -> [w912]
          frame #0 {
            # "Setup motor:\nDo in sequence because\nmotor waits for trigger signal"
            n323 = local write "Abort Continuous aquisition"(FALSE ("Abort Continuous aquisition")) -> ()
            n324 = call "rotation_control.vi"("Continuous output"=TRUE, "Wait for completion?"=FALSE, "Triggered start?"=TRUE, "Rotation orientation"="Rotation orientation", "waiting time"=0.0, "Duration of rotation"=w720, "Number of pulses"="Number of pulses per image") -> ("task out"=w727:refnum<k21>, "pulse duration (T/2)"=w719:dbl)  [unwired: 3 in]
            "Motor pulse time (T/2)" <- w719
            n325 = Bundle By Name(cluster=w725, "Motor pulse duration"=w719, "cw"="Rotation orientation", "Number of pulses per image"="Number of pulses per image", "Rotation enabled"=TRUE, "Rotary encoder type"="Bourns") -> (w721:T4)
          }
          frame #1 {
            w758 = -1.0
            w768 = 1000.0  # Init. max. RO
            w769 = 0 ("Images completed")
            # "TX cycles per img"
            # "Rotary queue"
            # "Absolute pos."
            # "Prev. ang"
            # "Shift register for readout"
            # "Tunnel for image repet."
            # "TX cycles per shift cycle"
            # "Readouts per Image"
            # "Data queue"
            n326 = local read "TX cycles per readout"() -> (w741:dbl)
            n327 = local read "baseline magnitude"() -> (w751:dbl)
            n328 = local read "baseline phase"() -> (w752:dbl)
            n329 = Multiply(x=w773, y=w741) -> (x*y=w778:dbl)
            n330 = Multiply(x=w741, y=w740) -> (x*y=w739:dbl)
            n331 = Format Into String("shift type") -> (resulting string=w762:string)  [unwired: 3 in, 1 out]
            n332 = Multiply(x=w739, y=2.0) -> (x*y=w737:dbl)
            n333 = call "gen_sine_shift.vi"("signal type"="shift type", "no of TX cycles per image"=w737, "Shift stop"="Shift stop", "Shift start"="Shift start", "time lag of shift system"="Shift field delay", "no of TX cycles per shift cycle"=w778) -> ("signal out"=w745:waveform(dbl), "Shift frequency"=w763:dbl)  [unwired: 4 in]
            "Shift frequency" <- w763
            n334 = call "gen_drive_waveform.vi"("no of cycles"=w737) -> ("signal out"=w776:waveform(dbl))  [unwired: 10 in]
            n335 = Bundle By Name(cluster=w742, "Shift frequency"=w763, "Shift waveform type"=w762, "Shift delay"="Shift field delay", "Shift start"="Shift start", "Shift stop"="Shift stop", "Baseline magnitude"=w751, "Baseline phase"=w752) -> (w736:T4)
            n336 = case shown="True" "Patch enable" {
              tunnel: w745 -> [w783 w790]
              tunnel: [w783 w789] -> w744
              tunnel: w742 -> [_ w788]
              tunnel: [0.0 ("patch amp") "patch amp"] -> w734
              tunnel: [-1.0 ("patch freq") w785] -> w733
              tunnel: [0.0 ("patch phase") "patch phase"] -> w732
              frame False {
              }
              frame True {
                n337 = Unbundle By Name(w788) -> ("Image time (calc)"=w787:dbl)
                n338 = call "patch_add.vi"("signal in"=w790, "phase"="patch phase", "amplitude"="patch amp", "image time"=w787) -> ("signal out"=w789:waveform(dbl), "patch freq"=w785:dbl)  [unwired: 6 in]
              }
            }
            "patch freq" <- w733
            n339 = call <extravilib>:"Write.vi"("element"=w768) -> ("channel"=w767:T6)  [unwired: 1 out]
            n340 = Bundle By Name(cluster=w736, "Patch amplitude"=w734, "Patch frequency"=w733, "Patch phase"=w732) -> (w735:T4)
            n341 = Initialize Array(waveform(dbl) {"t0"=timestamp(0 s since 1904-01-01), "dt"=1.0, "Y"=[]} ("Waveform")) -> (w771:waveform(dbl)[])  [unwired: 1 in]
            n342 = local read "readout pts"() -> (w775:dbl)
            n343 = local write "Images completed"(w769) -> ()
            n344 = Obtain Queue(element data type=dbl[] []) -> (queue out=w754:refnum<queue>)  [unwired: 4 in, 2 out]
            n345 = Obtain Queue(element data type=w771) -> (queue out=w779:refnum<queue>)  [unwired: 4 in, 2 out]
            n346 = Unbundle By Name(w735) -> ("cw"=w759:bool)
            n347 = call "transmit_receive.vi"("samples per readout"=w775, "rotary queue"=w754, "Continious mode"=TRUE, "Enable rotary encoder"=TRUE, "Waveform shift"=w744, "Waveform drive"=w776, "channel input for max readouts"=w767, "measurement queue"=w779) -> ()  [unwired: 4 in]
            n348 = local read "Readouts per projection (pk-pk)"() -> (w756:i32)
            n349 = local read "Projections"() -> (w765:i32)
            n350 = Multiply(x=w756, y=w765) -> (x*y=w770:i32)
            n351 = while "Consumer Loop" {
              tunnel: w779 -> [w835]
              shift-right: [w824] -> _
              shift-left: w735 -> [w833]
              tunnel: w770 -> [w815]
              shift-right: [w813] -> _
              shift-left: w769 -> [w819]
              tunnel: w735 -> [w818]
              tunnel: w767 -> [w817]
              tunnel: w746 -> [w812]
              tunnel: w760 -> [w811]
              tunnel: w759 -> [w809]
              shift-right: [w806] -> _
              shift-left: w758 -> [w808]
              shift-right: [w805] -> _
              shift-left: w758 -> [w807]
              tunnel: w757 -> [w801]
              tunnel: w757 -> [w800]
              tunnel: w756 -> [w798]
              tunnel: w754 -> [w797]
              tunnel: w753 -> [w793]
              shift-right: [w791] -> w749
              shift-left: w750 -> [w792]
              i -> [w795]
              stop <- w810 stop-if-true
              # "Rotary & trig"
              # "Shift"
              # "RX"
              n352 = Dequeue Element(queue=w835) -> (element=w794:waveform(dbl)[])  [unwired: 2 in, 3 out]
              n353 = Multiply(x=w811, y="Max images") -> (x*y=w803:i32)
              n354 = Add(x=w801, y=w803) -> (x+y=w802:dbl)
              "Max ROs" <- w802
              n355 = Index Array(array=w794, index=0) -> (element=w829:waveform(dbl))
              n356 = Index Array(array=w794, index=1) -> (element=w834:waveform(dbl))
              n357 = Dequeue Element(queue=w797) -> (element=w796:dbl[])  [unwired: 2 in, 3 out]
              n358 = call-poly <vilib>:"Number of Waveform Samples.vi"("waveform in"=w829) -> ("number of samples"=w838:i32)  [unwired: 8 in, 2 out]
              n359 = Equal To 0?(x=w838) -> (x = 0?=w810:bool)
              n360 = case "Data processing" shown="False" w810 {
                tunnel: w829 -> [w884 _]
                tunnel: w834 -> [w901 _]
                tunnel: w833 -> [w905 w910]
                tunnel: [w885 w910] -> w825
                tunnel: [w902 cluster{"f0":dbl, "df":dbl, "magnitude":dbl[]} {"f0"=0.0, "df"=0.0, "magnitude"=[]} ("magnitude")] -> w830
                tunnel: w809 -> [w887 _]
                tunnel: w808 -> [w894 w908]
                tunnel: w807 -> [w893 w907]
                tunnel: [w892 w908] -> w806
                tunnel: [w891 w907] -> w805
                tunnel: [w884 waveform(dbl) {"t0"=timestamp(0 s since 1904-01-01), "dt"=1.0, "Y"=[]} ("Waveform")] -> w799
                tunnel: w796 -> [w882 _]
                frame False {
                  # "Trigger lines"
                  n361 = local read "RX frequency"() -> (w895:dbl)
                  n362 = call-poly <vilib>:"FFT Spectrum (Mag-Phase).vi"("time signal"=w884) -> ("phase"=w904:cluster{"f0":dbl, "df":dbl, "phase":dbl[]}, "magnitude"=w902:cluster{"f0":dbl, "df":dbl, "magnitude":dbl[]})  [unwired: 6 in, 3 out]
                  n363 = call-poly <vilib>:"Mean.vi"("X"=w901) -> ("mean"=w900:dbl)  [unwired: 1 out]
                  "shift voltage over time" <- w900
                  n364 = Index Array(array=w882) -> (element=w899:dbl)  [unwired: 1 in]
                  n365 = Not(x=w887) -> (.not. x?=w886:bool)
                  n366 = call "rotary_encoder_lookup.vi"("Code from Encoder"=w899) -> ("angle (deg)"=w892:dbl)  [unwired: 10 in]
                  n367 = local read "baseline magnitude"() -> (w896:dbl)
                  n368 = local read "baseline phase"() -> (w897:dbl)
                  n369 = call "absolute_position.vi"("Encoder rotates cw"=w886, "curr. angle"=w892, "Absolute position in"=w893, "prev. angle"=w894) -> ("Absolute position out"=w891:dbl, "relative position wheel"=w889:dbl, "relative position shaft"=w890:dbl, "Wheel Position (abs)"=w888:dbl)  [unwired: 4 in]
                  n370 = call "determine_fourier_component.vi"("baseline magnitude"=w896, "baseline phase"=w897, "RX frequency"=w895, "phase"=w904, "magnitude"=w902) -> ("RX phase"=w903:dbl, "RX magnitude"=w883:dbl)  [unwired: 5 in]
                  n371 = Bundle("relative position shaft"=w890, "relative position wheel"=w889) -> (→"Rotary position":T7)  [unwired: 1 in]
                  n372 = Index Array(array=w882, index=1) -> (element=w880:dbl)
                  n373 = call "cluster_append.vi"("Trigger line"=w880, "Rotary encoder"=w888, "Input Cluster"=w905, "shift value"=w900, "phase value"=w903, "magnitude value"=w883) -> ("Output Cluster"=w885:T4)  [unwired: 5 in]
                }
                frame True {
                }
              }
              n374 = case "Time domain saving" shown="True" w793 {
                tunnel: w794 -> [_ w842]
                tunnel: w792 -> [w839 w841]
                tunnel: [w839 w840] -> w791
                frame False {
                }
                frame True {
                  n375 = TDMS Write(0:w841, 7:string[] ["RX", "shift"] ("channel name(s) in (Untitled)"), 9:w842) -> (4:w840:refnum<k34>)  [unwired: 3 in, 3 out]
                }
              }
              n376 = call <extravilib>:"Write With Abort.vi"("abort"="Abort Continuous aquisition", "element"=w802) -> ("channel"=w817:T6)  [unwired: 7 in, 2 out]
              n377 = Increment(x=w795) -> (x+1=w828:i32)
              n378 = Subtract(x=w828, y=w800) -> (x-y=w827:dbl)
              n379 = Quotient & Remainder(x=w827, y=w815) -> (x-y*floor(x/y)=w826:dbl, floor(x/y)=w823:dbl)
              n380 = Quotient & Remainder(x=w827, y=w798) -> (x-y*floor(x/y)=w832:dbl)  [unwired: 1 out]
              n381 = Not Equal To 0?(x=w823) -> (x != 0?=w820:bool)
              n382 = Equal To 0?(x=w826) -> (x = 0?=w822:bool)
              n383 = Equal To 0?(x=w832) -> (x = 0?=w831:bool)
              n384 = And(x=w822, y=w820) -> (x .and. y?=w821:bool)
              n385 = case "Image completed" shown="True" w821 {
                tunnel: w825 -> [w847 w852]
                tunnel: [w847 w856] -> w824
                tunnel: w819 -> [w846 w859]
                tunnel: [w846 w858] -> w813
                tunnel: w818 -> [_ w851]
                tunnel: w812 -> [_ w857]
                frame False {
                }
                frame True {
                  n386 = case shown="True" "Baseline set" {
                    tunnel: w852 -> [_ w865]
                    tunnel: w851 -> [w860 w864]
                    tunnel: [w860 w863] -> w850
                    frame False {
                    }
                    frame True {
                      n387 = call "baseline_update.vi"("Cluster in"=w865) -> ("new baseline phase"=w861:dbl, "new baseline magnitude"=w862:dbl)  [unwired: 9 in]
                      n388 = local write "baseline magnitude"(w862) -> ()
                      n389 = Bundle By Name(cluster=w864, "Baseline magnitude"=w862, "Baseline phase"=w861) -> (w863:T4)
                      n390 = local write "baseline phase"(w861) -> ()
                    }
                  }
                  n391 = Increment(x=w859) -> (x+1=w858:i32)
                  "Images completed" <- w858
                  n392 = Get Date/Time In Seconds() -> (seconds since 1Jan1904=w854:timestamp)
                  n393 = Bundle By Name(cluster=w852, "Image stop"=w854, "Notes"="Notes") -> (w853:T4)
                  n394 = Bundle By Name(cluster=w850, "Image start"=w854, "ramp-up readouts"=0) -> (w856:T4)
                  n395 = Enqueue Element(queue=w857, element=w853) -> ()  [unwired: 2 in, 3 out]
                }
              }
              n396 = case "Update plots after proj. completed" shown="True" w831 {
                tunnel: w825 -> [_ w877]
                tunnel: w830 -> [_ w871]
                tunnel: w799 -> [_ w874]
                frame False {
                }
                frame True {
                  n397 = Unbundle By Name(w877) -> ("ramp-up readouts"=w866:i32, "Magnitude meas."=w876:dbl[], "projections per image"=w868:i32, "readouts per projection"=w867:i32)
                  n398 = Unbundle By Name(w871) -> ("magnitude"=w870:dbl[])
                  n399 = Array Size(array=w870) -> (size(s)=w869:i32)
                  n400 = Not Equal To 0?(x=w869) -> (x != 0?=w872:bool)
                  n401 = call "resort_sinogram_data.vi"("Ramp end"=0, "Ramp begin"=w866, "Shift up and down"=TRUE, "pts per projection"=w867, "projections"=w868, "Input"=w876) -> ("Output"=→"raw sinogram":dbl[][])  [unwired: 5 in]
                  n402 = case shown="True" w872 {
                    tunnel: w871 -> [_ w879]
                    frame False {
                    }
                    frame True {
                      "fft magnitude" <- w879
                    }
                  }
                  "waveform diagram" <- w874
                }
              }
              n403 = case shown="True" "Stop continuous imaging" {
                tunnel: w813 -> [_ w844]
                frame False {
                }
                frame True {
                  n404 = Increment(x=w844) -> (x+1=w845:i32)
                  n405 = local write "Max images"(w845) -> ()
                }
              }
              "Current readout" <- w795
            }
          }
          frame #2 {
            # "Stop rotation"
            # "Signal the consumer loop for image saving and recon that aquisition of image series has ended"
            n406 = case shown="True" w913 {
              tunnel: w914 -> [_ w917]
              frame False {
              }
              frame True {
                # "Close file for time domain saving"
                n407 = TDMS Close(11:w917) -> ()  [unwired: 1 in, 2 out]
              }
            }
            n408 = call <vilib>:"DAQmx Clear Task.vi"("task in"=w916) -> ()  [unwired: 14 in, 1 out]
            n409 = local write "Abort Continuous aquisition"(FALSE ("Abort Continuous aquisition")) -> ()
            n410 = Enqueue Element(queue=w912, element=T4 {"Magnitude meas."=[], "Phase meas."=[], "Shift meas."=[], "cw"=TRUE, "projections per image"=0, "ramp-up readouts"=0, "current sense type"="", "Number of pulses per image"=0, "Rotation enabled"=TRUE, "Rotary position"=[], "Baseline magnitude"=0.0, "Baseline phase"=0.0, "Wait readouts"=0, "Shift waveform type"="", "Shift enabled"=TRUE, "Time domain data"=[], "Motor pulse duration"=0.0, "Shift start"=0.0, "Shift stop"=0.0, "Notes"="", "Reconstructed image"=bytes[0], "Rotary encoder type"="", "Image start"=timestamp(0 s since 1904-01-01), "Image stop"=timestamp(0 s since 1904-01-01), "readouts per projection"=0, "Recon enabled"=FALSE, "Bidirectional shift"=FALSE, "Imager mode"="", "Shift delay"=0.0, "Shift frequency"=0.0, "Image time (calc)"=0.0, "Initial encoder position"=0.0, "Recon data"=[], "Trigger line values"=[], "Bed position"=0.0, "Sample image"=bytes[0], "Patch amplitude"=0.0, "Patch frequency"=0.0, "Patch phase"=0.0}) -> ()  [unwired: 2 in, 3 out]
          }
          frame #3 {
            w918 = 0 ("Number of pulses")
            # "Release break"
            n411 = call "rotation_control.vi"("Continuous output"=FALSE, "Wait for completion?"=TRUE, "Triggered start?"=FALSE, "waiting time"=0.01, "Duration of rotation"=w918, "Number of pulses"=w918) -> ()  [unwired: 4 in, 2 out]
          }
        }
        n412 = local read "Readouts per projection (pk-pk)"() -> (w690:i32)
        n413 = Divide(x=w690, y=2) -> (x/y=w688:dbl)
        n414 = Obtain Queue(element data type=T4 {"Magnitude meas."=[], "Phase meas."=[], "Shift meas."=[], "cw"=TRUE, "projections per image"=0, "ramp-up readouts"=0, "current sense type"="", "Number of pulses per image"=0, "Rotation enabled"=TRUE, "Rotary position"=[], "Baseline magnitude"=0.0, "Baseline phase"=0.0, "Wait readouts"=0, "Shift waveform type"="", "Shift enabled"=TRUE, "Time domain data"=[], "Motor pulse duration"=0.0, "Shift start"=0.0, "Shift stop"=0.0, "Notes"="", "Reconstructed image"=bytes[0], "Rotary encoder type"="", "Image start"=timestamp(0 s since 1904-01-01), "Image stop"=timestamp(0 s since 1904-01-01), "readouts per projection"=0, "Recon enabled"=FALSE, "Bidirectional shift"=FALSE, "Imager mode"="", "Shift delay"=0.0, "Shift frequency"=0.0, "Image time (calc)"=0.0, "Initial encoder position"=0.0, "Recon data"=[], "Trigger line values"=[], "Bed position"=0.0, "Sample image"=bytes[0], "Patch amplitude"=0.0, "Patch frequency"=0.0, "Patch phase"=0.0}) -> (queue out=w703:refnum<queue>)  [unwired: 4 in, 2 out]
        n415 = call "save_and_process_continious_image_data.vi"("Path"=w681, "Save"="Save enable\n(before start)", "Enable online recon"="Online recon", "queue in"=w703) -> ()  [unwired: 8 in]
      }
      frame "Rotation homing" {
        n416 = call "rotation_homing.vi"() -> ()  [unwired: 12 in]
      }
      frame "Halt" {
      }
      frame "Update global variables" {
        w924 = dbl[] [131.0, 135.0, 139.0, 143.0, 147.0, 151.0, 155.0, 159.0, 163.0, 167.0, 171.0, 175.0, 179.0, 183.0, 187.0, 191.0, 195.0, 199.0, 203.0, 207.0, 211.0, 215.0, 219.0, 223.0, 227.0, 231.0, 235.0, 239.0, 243.0, 247.0, 251.0, 255.0, 1279.0, 2303.0, 3327.0, 4351.0, 5375.0, 6399.0, 7423.0, 8447.0, 9471.0, 10495.0, 11519.0, 12543.0, 13567.0, 14591.0, 15615.0, 16639.0, 17663.0, 18687.0, 19711.0, 20735.0, 21759.0, 22783.0, 23807.0, 24831.0, 25855.0, 26879.0, 27903.0, 28927.0, 29951.0, 30975.0, 31999.0, 33023.0, 33791.0, 34815.0, 35839.0, 36863.0, 37887.0, 38911.0, 39935.0, 40959.0, 41983.0, 43007.0, 44031.0, 45055.0, 46079.0, 47103.0, 48127.0, 49151.0, 50175.0, 51199.0, 52223.0, 53247.0, 54271.0, 55295.0, 56319.0, 57343.0, 58367.0, 59391.0, 60415.0, 61439.0, 62463.0, 63487.0, 64511.0, 65535.0, 327675.0, 589815.0, 851955.0, 1114095.0, 1376235.0, 1638375.0, 1900515.0, 2162655.0, 2424795.0, 2686935.0, 2949075.0, 3211215.0, 3473355.0, 3735495.0, 3997635.0, 4259775.0, 4521915.0, 4784055.0, 5046195.0, 5308335.0, 5570475.0, 5832615.0, 6094755.0, 6356895.0, 6619035.0, 6881175.0, 7143315.0, 7405455.0, 7667595.0, 7929735.0, 8191875.0, 8454016.0, 8650620.0, 8912760.0, 9174900.0, 9437040.0, 9699180.0, 9961320.0, 10223460.0, 10485600.0, 10747740.0, 11009880.0, 11272020.0, 11534160.0, 11796300.0, 12058440.0, 12320580.0, 12582720.0, 12844860.0, 13107000.0, 13369140.0, 13631280.0, 13893420.0, 14155560.0, 14417700.0, 14679840.0, 14941980.0, 15204120.0, 15466260.0, 15728400.0, 15990540.0, 16252680.0, 16514820.0, 16776960.0, 16775936.0, 16774912.0, 16773888.0, 16772864.0, 16771840.0, 16770816.0, 16769792.0, 16768768.0, 16767744.0, 16766720.0, 16765696.0, 16764672.0, 16763648.0, 16762624.0, 16761600.0, 16760576.0, 16759552.0, 16758528.0, 16757504.0, 16756480.0, 16755456.0, 16754432.0, 16753408.0, 16752384.0, 16751360.0, 16750336.0, 16749312.0, 16748288.0, 16747264.0, 16746240.0, 16745216.0, 16744448.0, 16743424.0, 16742400.0, 16741376.0, 16740352.0, 16739328.0, 16738304.0, 16737280.0, 16736256.0, 16735232.0, 16734208.0, 16733184.0, 16732160.0, 16731136.0, 16730112.0, 16729088.0, 16728064.0, 16727040.0, 16726016.0, 16724992.0, 16723968.0, 16722944.0, 16721920.0, 16720896.0, 16719872.0, 16718848.0, 16717824.0, 16716800.0, 16715776.0, 16714752.0, 16713728.0, 16712704.0, 16711680.0, 16449536.0, 16187392.0, 15925248.0, 15663104.0, 15400960.0, 15138816.0, 14876672.0, 14614528.0, 14352384.0, 14090240.0, 13828096.0, 13565952.0, 13303808.0, 13041664.0, 12779520.0, 12517376.0, 12255232.0, 11993088.0, 11730944.0, 11468800.0, 11206656.0, 10944512.0, 10682368.0, 10420224.0, 10158080.0, 9895936.0, 9633792.0, 9371648.0, 9109504.0, 8847360.0, 8585216.0] ("output array")
        # "Don't delete this array constant! It was a pain to build the jet colormap from MATLAB in LabVIEW!"
        n417 = flat-sequence {
          frame #0 {
            # "Reset DAQ"
            n418 = global read "global_variables.vi" "Device Name"() -> (w930:tag)
            n419 = call <vilib>:"DAQmx Reset Device.vi"("device in"=w930) -> ()  [unwired: 14 in, 1 out]
          }
          frame #1 {
            n420 = global write "global_variables.vi" "Receive range"("RX max amplitude (V)") -> ()
            n421 = global write "global_variables.vi" "Transmit amplitude"("TX amplitude\n(peak 1 ch)") -> ()
            n422 = local read "TX frequency"() -> (w934:dbl)
            n423 = local read "sampling rate"() -> (w935:dbl)
            n424 = local read "RX frequency"() -> (w932:dbl)
            n425 = local read "TX cycles per readout"() -> (w931:dbl)
            n426 = global write "global_variables.vi" "sample rate digital out"("sampling rate digital out") -> ()
            n427 = Divide(x=w935, y=w934) -> (x/y=w933:dbl)
            n428 = global write "global_variables.vi" "Receive frequency"(w932) -> ()
            n429 = Multiply(x=w933, y=w931) -> (x*y=w937:dbl)
            n430 = Round To Nearest(number=w937) -> (nearest integer value=→"readout pts":dbl)
            n431 = global write "global_variables.vi" "TX cycles"(w931) -> ()
            n432 = global write "global_variables.vi" "Transmit frequency"("TX frequency") -> ()
            n433 = global write "global_variables.vi" "sample rate"("sampling rate") -> ()
          }
          frame #2 {
            w943 = 0 ("Number of pulses")
            # "Release break"
            n434 = call "rotation_control.vi"("Continuous output"=FALSE, "Wait for completion?"=TRUE, "Triggered start?"=FALSE, "waiting time"=0.01, "Duration of rotation"=w943, "Number of pulses"=w943) -> ()  [unwired: 4 in, 2 out]
          }
        }
        n435 = Enqueue Element(queue=w928, element="Idle") -> ()  [unwired: 2 in, 3 out]
        n436 = local read "RX frequency"() -> (w926:dbl)
        n437 = property on="fft magnitude" class="WFGraph (strict)"("Active Cursor"=u32 0, "Cursor.Cursor X"=w926) -> ()  [unwired: 2 in, 2 out]
        n438 = property on="fft magnitude" class="WFGraph (strict)"("BG Color"=u32 16448250) -> ()  [unwired: 2 in, 2 out]
        n439 = property on="raw sinogram" class="IntGraph (strict)"("Color Table"=w924) -> ()  [unwired: 2 in, 2 out]
        n440 = property on="raw sinogram" class="IntGraph (strict)"("Color Table"=w924) -> ()  [unwired: 2 in, 2 out]
        n441 = property on="raw sinogram" class="IntGraph (strict)"("Color Table"=w924) -> ()  [unwired: 2 in, 2 out]
      }
      frame "Clear plots" {
        w953 = waveform(dbl) {"t0"=timestamp(0 s since 1904-01-01), "dt"=1.0, "Y"=[]} ("Waveform")
        w956 = 0.0
        w958 = waveform(dbl) {"t0"=timestamp(0 s since 1904-01-01), "dt"=1.0, "Y"=[]} ("Waveform")
        w959 = waveform(dbl) {"t0"=timestamp(0 s since 1904-01-01), "dt"=1.0, "Y"=[]} ("Waveform")
        # "Swinging imaging"
        # "Pulsed imaging"
        # "Init the spectroscopy plots"
        n442 = Enqueue Element(queue=w960, element="Idle") -> ()  [unwired: 2 in, 3 out]
        n443 = local write "waveform diagram"(waveform(dbl) {"t0"=timestamp(0 s since 1904-01-01), "dt"=1.0, "Y"=[]} ("Waveform")) -> ()
        n444 = local write "RX phase over time"(w959) -> ()
        n445 = local write "RX magnitude over time"(w959) -> ()
        n446 = property on="RX phase last 150 points" class="WFChart (strict)"("History Data"=w959) -> ()  [unwired: 2 in, 2 out]
        n447 = property on="RX magnitude last 150 points" class="WFChart (strict)"("History Data"=w959) -> ()  [unwired: 2 in, 2 out]
        n448 = local write "Projections completed"(w956) -> ()
        n449 = Initialize Array(w956) -> (w957:dbl[][])  [unwired: 2 in]
        n450 = property on="RX magnitude over time (1000 readouts)" class="WFChart (strict)"("History Data"=w958) -> ()  [unwired: 2 in, 2 out]
        n451 = property on="RX phase over time (1000 readouts)" class="WFChart (strict)"("History Data"=w958) -> ()  [unwired: 2 in, 2 out]
        n452 = property on="Shift current" class="WFChart (strict)"("History Data"=w958) -> ()  [unwired: 2 in, 2 out]
        n453 = local write "raw sinogram"(w957) -> ()
        n454 = Initialize Array(0.0) -> (w954:dbl[][])  [unwired: 2 in]
        n455 = property on="RX magnitude over time (1000 readouts)" class="WFChart (strict)"("History Data"=w953) -> ()  [unwired: 2 in, 2 out]
        n456 = property on="RX phase over time (1000 readouts)" class="WFChart (strict)"("History Data"=w953) -> ()  [unwired: 2 in, 2 out]
        n457 = property on="shift voltage over time" class="WFChart (strict)"("History Data"=w953) -> ()  [unwired: 2 in, 2 out]
        n458 = local write "raw sinogram"(w954) -> ()
        n459 = Initialize Array(0.0) -> (w949:dbl[][])  [unwired: 2 in]
        n460 = property on="shift voltage over time" class="WFChart (strict)"("History Data"=waveform(dbl) {"t0"=timestamp(0 s since 1904-01-01), "dt"=1.0, "Y"=[]} ("Waveform")) -> ()  [unwired: 2 in, 2 out]
        n461 = local write "fft magnitude"(cluster{dbl, dbl, dbl[]} {0.0, 0.0, []} ("fft magnitude")) -> ()
        n462 = local write "raw sinogram"(w949) -> ()
      }
    }
  }
  n463 = global read "global_variables.vi" "Watchdog lines"() -> (w10:tag)
  n464 = call-poly <vilib>:"DAQmx Create Virtual Channel.vi"("lines"=w10) -> ("task out"=w22:refnum<k21>, "error out"=w21:errorcluster)  [unwired: 13 in]
  n465 = global read "global_variables.vi" "PDU IP or Hostname"() -> (w2:string)
  n466 = while "PDU Switch Loop" {
    stop <- w962 stop-if-true
    n467 = event shown="[4] \"Align laser\": Value Change" {
      selector: _ -> [_ _ _ _ _]
      dyn-events: _ -> [_ _ _ _ _]
      timeout: 100 -> [_ _ _ _ _]
      tunnel: [w964 _ _ _ _] -> w962
      event Timeout {
        n468 = event-data() -> ()  [unwired: 1 in, 3 out]
        n469 = local read "Main loop has stopped"() -> (w964:bool)
      }
      event "Motor": Value Change {
        n470 = event-data() -> ()  [unwired: 1 in, 5 out]
        n471 = global read "global_variables.vi" "PDU IP or Hostname"() -> (w965:string)
        n472 = call "set_single_outlet.vi"("Switch state"="Motor", "Outlet #"=1, "IP / Hostname"=w965) -> ()  [unwired: 9 in]
      }
      event "Pumps": Value Change {
        n473 = event-data() -> ()  [unwired: 1 in, 6 out]
        n474 = global read "global_variables.vi" "PDU IP or Hostname"() -> (w970:string)
        n475 = call "set_single_outlet.vi"("Switch state"="Pumps", "Outlet #"=2, "IP / Hostname"=w970) -> ()  [unwired: 9 in]
      }
      event "Bed motor": Value Change {
        n476 = event-data() -> ()  [unwired: 1 in, 6 out]
        n477 = global read "global_variables.vi" "PDU IP or Hostname"() -> (w973:string)
        n478 = call "set_single_outlet.vi"("Switch state"="Bed motor", "Outlet #"=3, "IP / Hostname"=w973) -> ()  [unwired: 9 in]
      }
      event "Align laser": Value Change {
        n479 = event-data() -> ()  [unwired: 1 in, 6 out]
        n480 = global read "global_variables.vi" "PDU IP or Hostname"() -> (w976:string)
        n481 = call "set_single_outlet.vi"("Switch state"="Align laser", "Outlet #"=8, "IP / Hostname"=w976) -> ()  [unwired: 9 in]
      }
    }
  }
  n482 = while "Safety loop" {
    shift-right: [w989] -> w20
    shift-left: w22 -> [w993]
    shift-right: [w987] -> w19
    shift-left: w21 -> [w992]
    tunnel: [w977] -> w14
    tunnel: [FALSE ("auto start")] -> w12
    shift-right: [w978] -> _
    shift-left: TRUE -> [w979]
    stop <- w994 stop-if-true
    w977 = FALSE  # Line currently not in use
    n483 = case shown="True" "reset daq" {
      frame False {
      }
      frame True {
        n484 = global read "global_variables.vi" "Device Name"() -> (w995:tag)
        n485 = call <vilib>:"DAQmx Reset Device.vi"("device in"=w995) -> ()  [unwired: 14 in, 1 out]
      }
    }
    n486 = Not(x=w979) -> (.not. x?=w978:bool)
    n487 = Build Array(w977, w978, "TX amp", "Shift amp") -> (w982:bool[])
    n488 = Build Array(w982) -> (w981:bool[][])
    n489 = call-poly <vilib>:"DAQmx Write.vi"("task/channels in"=w993, "auto start"=TRUE, "data"=w981, "error in"=w992) -> ("task out"=w990:refnum<k21>, "error out"=w988:errorcluster)  [unwired: 9 in, 1 out]
    n490 = local read "Main loop has stopped"() -> (w994:bool)
    n491 = Wait Until Next ms Multiple(millisecond multiple=u32 500) -> ()  [unwired: 1 out]
    n492 = call <vilib>:"DAQmx Wait Until Done.vi"("task/channels in"=w990, "error in"=w988) -> ("task out"=w989:refnum<k21>, "error out"=w987:errorcluster)  [unwired: 12 in]
  }
  n493 = call "query_single_outlet.vi"("outlet #"=1, "IP / Hostname"=w2) -> ("status"=w8:bool)  [unwired: 9 in]
  n494 = local write "Motor"(w8) -> ()
  n495 = call "query_single_outlet.vi"("outlet #"=2, "IP / Hostname"=w2) -> ("status"=w7:bool)  [unwired: 9 in]
  n496 = local write "Pumps"(w7) -> ()
  n497 = call "query_single_outlet.vi"("outlet #"=3, "IP / Hostname"=w2) -> ("status"=w4:bool)  [unwired: 9 in]
  n498 = local write "Bed motor"(w4) -> ()
  n499 = while {
    stop <- w997 stop-if-true
    n500 = case shown="True" "Enable power plotting" {
      frame False {
        n501 = Wait Until Next ms Multiple(millisecond multiple=u32 100) -> ()  [unwired: 1 out]
      }
      frame True {
        n502 = global read "global_variables.vi" "PDU IP or Hostname"() -> (w1006:string)
        n503 = call "power_monitor.vi"("IP / Hostname"=w1006) -> ("voltage"=→"V":dbl, "frequency"=→"f":dbl, "apparant power (watt)"=w1003:i32, "active power (watt)"=w1002:i32, "power factor"=→"Power factor":dbl)  [unwired: 10 in]
        n504 = Bundle("apparant power (watt)"=w1003, "active power (watt)"=w1002) -> (→"Waveform Chart":T1)  [unwired: 1 in]
        n505 = Wait Until Next ms Multiple(millisecond multiple=u32 1000) -> ()  [unwired: 1 out]
      }
    }
    n506 = local read "Main loop has stopped"() -> (w997:bool)
  }
  n507 = call "query_single_outlet.vi"("outlet #"=8, "IP / Hostname"=w2) -> ("status"=w1:bool)  [unwired: 9 in]
  n508 = local write "Shift amp"(w12) -> ()
  n509 = local write "TX amp"(w12) -> ()
  n510 = Build Array(w14, w12, w12, w12) -> (w15:bool[])
  n511 = local write "Align laser"(w1) -> ()
  n512 = Build Array(w15) -> (w13:bool[][])
  n513 = call-poly <vilib>:"DAQmx Write.vi"("task/channels in"=w20, "auto start"=TRUE, "data"=w13, "error in"=w19) -> ("task out"=w17:refnum<k21>, "error out"=w18:errorcluster)  [unwired: 9 in, 1 out]
  n514 = call <vilib>:"DAQmx Clear Task.vi"("task in"=w17, "error in"=w18) -> ()  [unwired: 13 in, 1 out]
  n515 = local write "Main loop has stopped"(w23) -> ()
  "Main loop has stopped" <- FALSE ("Main loop has stopped")
